vi "FRAM.vi"() -> ()   [LabVIEW 2019]
panel:
  out "PI-02- Bruto":dbl
  in  "P2-LIMITE":bool
  out "SHD-PI-02-AUX":dbl
  in  "Atualizar_Velocidades":bool
  out "JW_aux":dbl
  out "JK_aux":dbl
  out "JG_aux":dbl
  in  "JG_Title":string
  in  "JK_Title":string
  in  "JW_Title":string
  out "JG_Lam [m/s]":dbl
  out "T_K [°C]":dbl
  out "T_W [°C]":dbl
  in  "automatico/M_manual":bool
  in  "M_manual":dbl
  out "T_mis [°C]":dbl
  out "T_Atm_CLP":dbl
  out "Ll":dbl
  out "Lm":dbl
  out "T_Atm [°C]":dbl
  out "Lk":dbl
  out "Lw":dbl
  out "JL [m/s]":dbl
  out "T_W_CLP":dbl
  out "T_K_CLP":dbl
  out "SKM-NC-CV-COR":bool
  out "SKM-NC-CV-LAM":bool
  out "T_Ar_CLP":dbl
  out "DP_Lam_CLP":dbl
  out "SKM-AI-KF-COR_CLP [kg/m³]":dbl
  out "P_Bar_CLP":dbl
  out "P_Lam_CLP":dbl
  out "M_K_CLP":dbl
  out "P_Lam [KPa]":dbl
  out "P_Bar [KPa]":dbl
  out "Q_W_CLP":dbl
  out "Q_W [m³/s]":dbl
  out "DP_Lam [KPa]":dbl
  out "SKM-FIC-AR-COR_CLP  [kg/s]":dbl
  out "T_Ar [°C]":dbl
  out "Rho_K [Kg/m³]":dbl
  out "Rho_W [Kg/m³]":dbl
  out "SIT-NC-CV-001":bool
  out "SIA-NC-CV-001":bool
  out "SKS-NC-CV-006":bool
  out "SIW-NC-CV-001":bool
  out "SKS-NC-CV-003":bool
  out "SKS-NC-CV-002":bool
  out "SIT-NC-CV-002":bool
  in  "Certificado_Calibracao 2":bool
  in  "Certificado_Calibracao1":bool
  out "Execution:State":T1(ring)
  out "SHD-PI-02":dbl(knob) scale=2.0..2000.0
  out "STRING":string
  in  "Teste 234":bool
  in  "MWU2987":i16
  out "String Caracter de Comunicação":string
  out "JG [m/s]":dbl
  out "JW [m/s]":dbl
  out "JK [m/s]":dbl
  in  "MWU2986":i16
  in  "MWU2985":i16
  in  "MWU2984":i16
  in  "MWU2983":i16
  in  "MWU2982":i16
  in  "MWU2981":i16
  in  "MWU2980":i16
  in  "MWU2979":i16
  in  "MWU2978":i16
  in  "MWU2977":i16
  in  "MWU2976":i16
  in  "MWU2975":i16
  in  "MWU2925":i16
  out "MWU1100":i16
  in  "caixinha":bool
  out "Altura Líquido-régua":dbl
  out "Altura Kerosene-régua":dbl
  out "Altura Água-régua":dbl
  out "Hk Mer erro":dbl format="%.6g"
  out "Hw Mer erro":dbl format="%.6g"
  out "Vazio Mer erro":dbl format="%.6g"
  out "Hk Free erro":dbl format="%.6g"
  out "Hw Free erro":dbl format="%.6g"
  out "Vazio Free erro":dbl format="%.6g"
  out "Hk  Misto erro":dbl format="%.6g"
  out "Hw Misto erro":dbl format="%.6g"
  out "Vazio Misto erro":dbl format="%.6g"
  out "led Hw":bool
  out "led Hk":bool
  out "led Vazio":bool
  out "led SHD":bool
  out "Altura Liquido erro":dbl format="%#_1g"
  in  "Calibração":bool
  out "Altura Kerosene erro":dbl format="%#_4g"
  out "Altura Água erro":dbl format="%#_4g"
  out "Hw Mer":dbl format="%#_3g"
  out "Hk Mer":dbl format="%#_3g"
  out "Vazio Mer":dbl format="%#_3g"
  in  "Documentação":bool
  in  "Cluster 2":T2
  in  "Cluster":T3 {"Progresso Sensor" scale=0.0..90.0}
  out "SHD-PI-01":dbl(knob) scale=2.0..2000.0
  out "Gráfico":dbl[][](graph)
  out "Hw Free":dbl format="%#_3g"
  out "Hk Free":dbl format="%#_3g"
  out "Vazio  Free":dbl format="%#_3g"
  out "Hw":dbl format="%#_3g"
  out "Hk":dbl format="%#_3g"
  out "Vazio":dbl format="%#_3g"
  out "Altura Líquido":dbl
  in  "Alinhamento":bool
  in  "Gravar teste":bool
  in  "Parar Teste":bool
  out "SHD-PI-02-Ind.":dbl
  out "SHD-PI-01-Ind.":dbl
  out "T roxo":bool
  out "SIT-CV-AT":bool
  out "cano roxo h":bool
  out "SIT-CV-ST":bool
  out "SIT-CV-ST":bool
  out "cano roxo":bool
  out "Altura Kerosene":dbl
  out "Altura Água":dbl
  in  "Medição":bool
  in  "Teste":bool
  in  "stop VI":bool
  out "reference":refnum<vi>
  in  "Tempo de comunicação":i32
  in  "String 12":string
  in  "String 11":string
  in  "String 10":string
  in  "String 9":string
  in  "String 8":string
  in  "String 7":string
  in  "String 6":string
  in  "String 5":string
  in  "String 4":string
  in  "String 3":string
  in  "String 2":string
  in  "String 1":string
  out "UHk":dbl
  out "UHw":dbl
  out "Ua":dbl
  out "ULw":dbl
  out "Lw(valor mais provavel)":dbl
  out "Calculo de gama":dbl
  out "(Uwp2)²":dbl
  out "(Uwp1)²":dbl
  out "Lwp2":dbl
  out "Lwp1":dbl
  out "Uwd(incerteza free)":dbl
  out "L_w":dbl
  out "L_k":dbl
  in  "HELP-SIT":bool
  out "JANELA":bool
  out "HKSO":dbl
  out "HWSO":dbl
  out "L_a":dbl
  out "H L":dbl
  out "Rho_Ar [kg/m³]":dbl
  out "P1-P2":dbl
  out "PM":dbl
  out "Valores":T4
  out "Hexa p OPC":string
  in  "Pressão02-CLP[0-4095]":dbl
  in  "Pressão01_CLP[0-4095]":dbl
  out "T azul":bool
  out "cano azul h":bool
  out "cano verde":bool
  out "cano amarelo":bool
  out "cano azul v":bool
  # "FreeScale"
  # "Pressão"
  # "Ótico"
  # "Régua"
  # "Altura\nLíquido"
  # "+"
  # "mm"
  # "mm"
  # "mm"
  # "-"
  # "Altura\nÁgua"
  # "+"
  # "mm"
  # "mm"
  # "mm"
  # "-"
  # "Altura \nQuerosene"
  # "+"
  # "mm"
  # "mm"
  # "mm"
  # "-"
  # "Merge"
  # "FreeScale"
  # "Misto"
  # "[%]"
  # "[Erro]"
  # "[%]"
  # "[Erro]"
  # "[%]"
  # "[Erro]"
  # "+"
  # "+"
  # "Vazão Mássica - Manual"
  # "+"
  # "-"
  # "-"
  # "-"
  # "+"
  # "+"
  # "+"
  # "-"
  # "-"
  # "-"
  # "Variaveis Merge"
  # "+"
  # "+"
  # "+"
  # "-"
  # "-"
  # "-"
  # "mm"
  # "mmH2O"
  # "Smar"
  # "Emerson"
  # "Insira os valores de JW, JK e JG para criação do título do arquivo gravado:"
  # "mm"
  # "mm²"
  # "ms"
  # "mmH2O"
  # "mm"
  # "mm"
  # "mm²"
  # "mm"
  # "mm"
  # "JW [m/s]"
  # "COMUNICA敲O SERIAL"
  # "mm"
  # "mm"
  # "mm"
  # "JK [m/s]"
  # "mm"
  # "mm"
  # "Kg/m³"
  # "JG [m/s]"
  # "mm"
  # "mm"
  # "KPa Abs."
  # "mmH2O"
  # "[s]"
  # "MAX"
  # "MIN"
  # "mmH2O"
  # "mmH2O"
  # "mm"
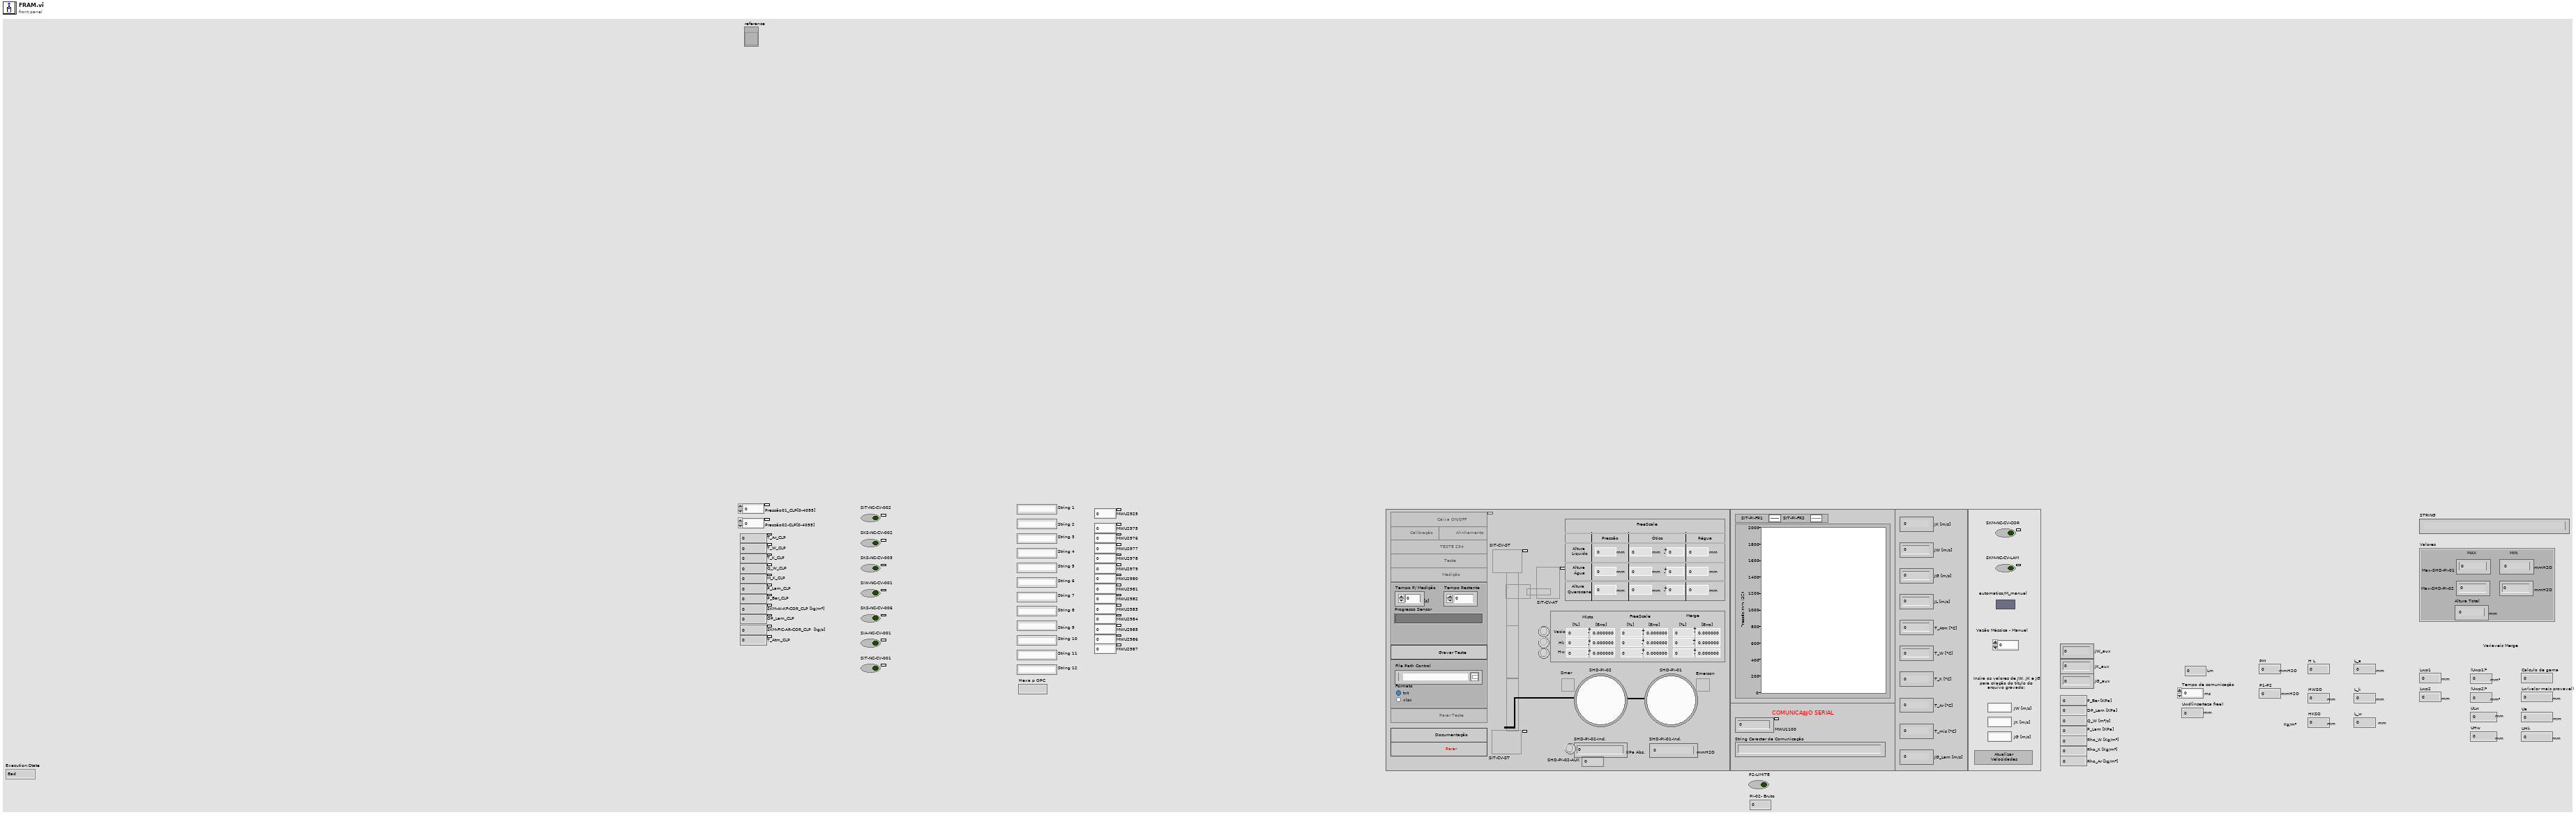
[diagram p1: front panel]
types:
  T1 = enum32{"Bad", "Idle", "Run top level", "Running"}
  T2 = cluster{"File Path Control":path, "Formato":enum32{"Item 0", "Item 1"}}
  T3 = cluster{"Tempo P/ Medição":dbl, "Tempo Restante":dbl, "Home":bool, "Progresso Sensor":dbl}
  T4 = cluster{"Max-SHD-PI-01":i32, "Min-SIT-PI-FR1":i32, "Max-SHD-PI-02":i32, "Min-SIT-PI-FR2":i32, "Altura Total":i32}
  T5 = enum8{"Enabled", "Disabled", "Disabled and Grayed Out"}
  T6 = enum32{"Invalid", "Standard", "Closed", "Hidden", "Minimized", "Maximized"}
  T7 = cluster{"String para labview 1":string, "String para labview 2":string, "String para labview 3":string, "String para labview 4":string, "String para labview 5":string, "String para labview 6":string, "String para labview 7":string, "String para labview 8":string, "String para labview 9":string, "String para labview 10":string, "String para labview 11":string, "String para labview 12":string}
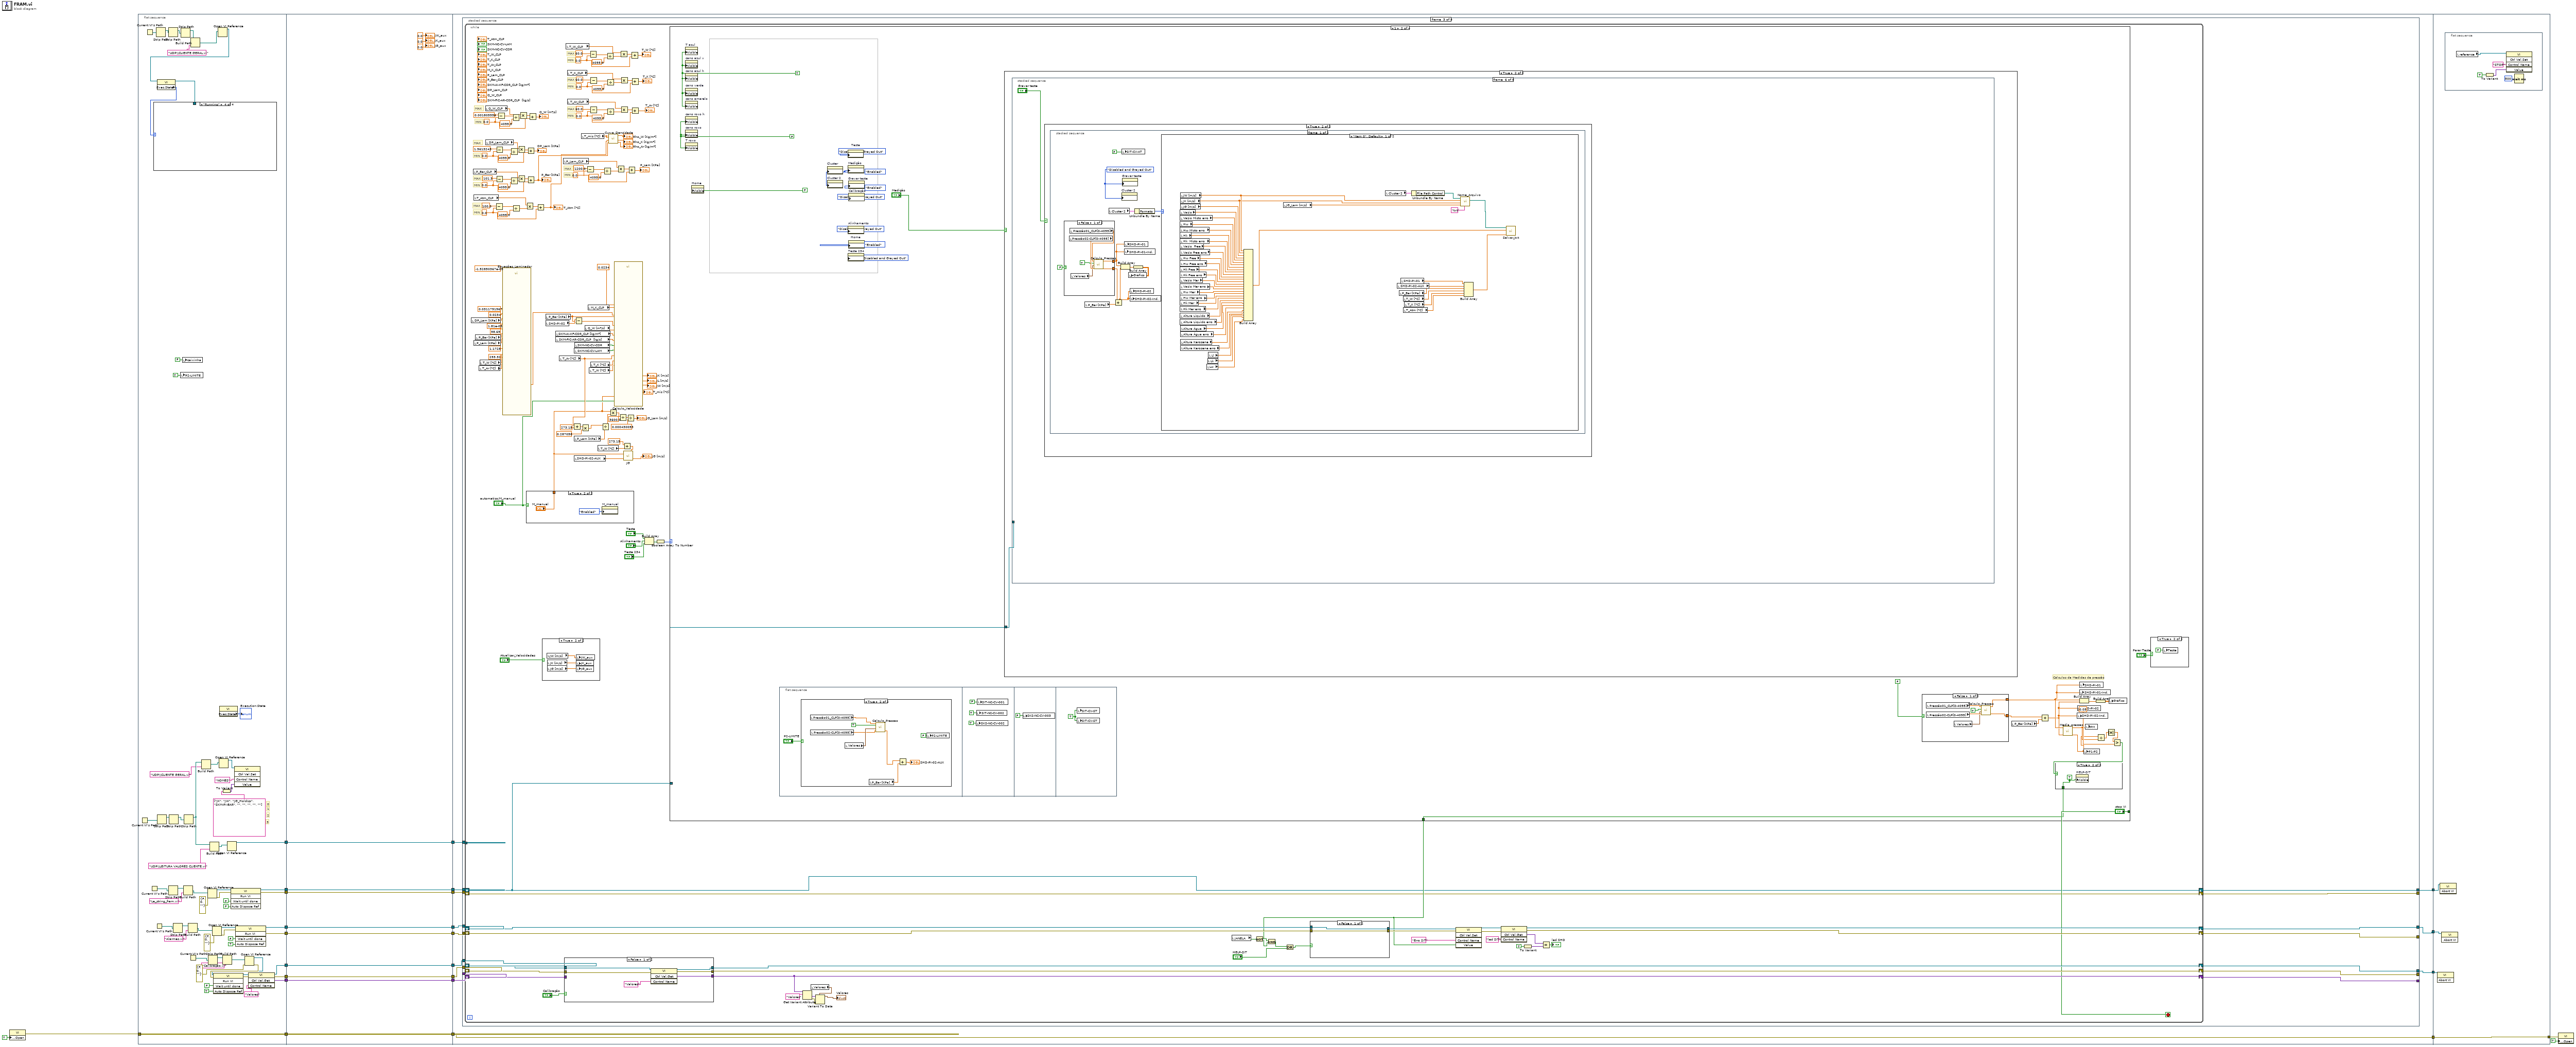
[diagram p0: block diagram]
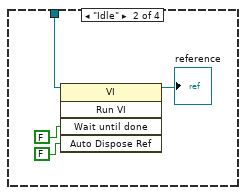
[diagram p3: hidden frame]
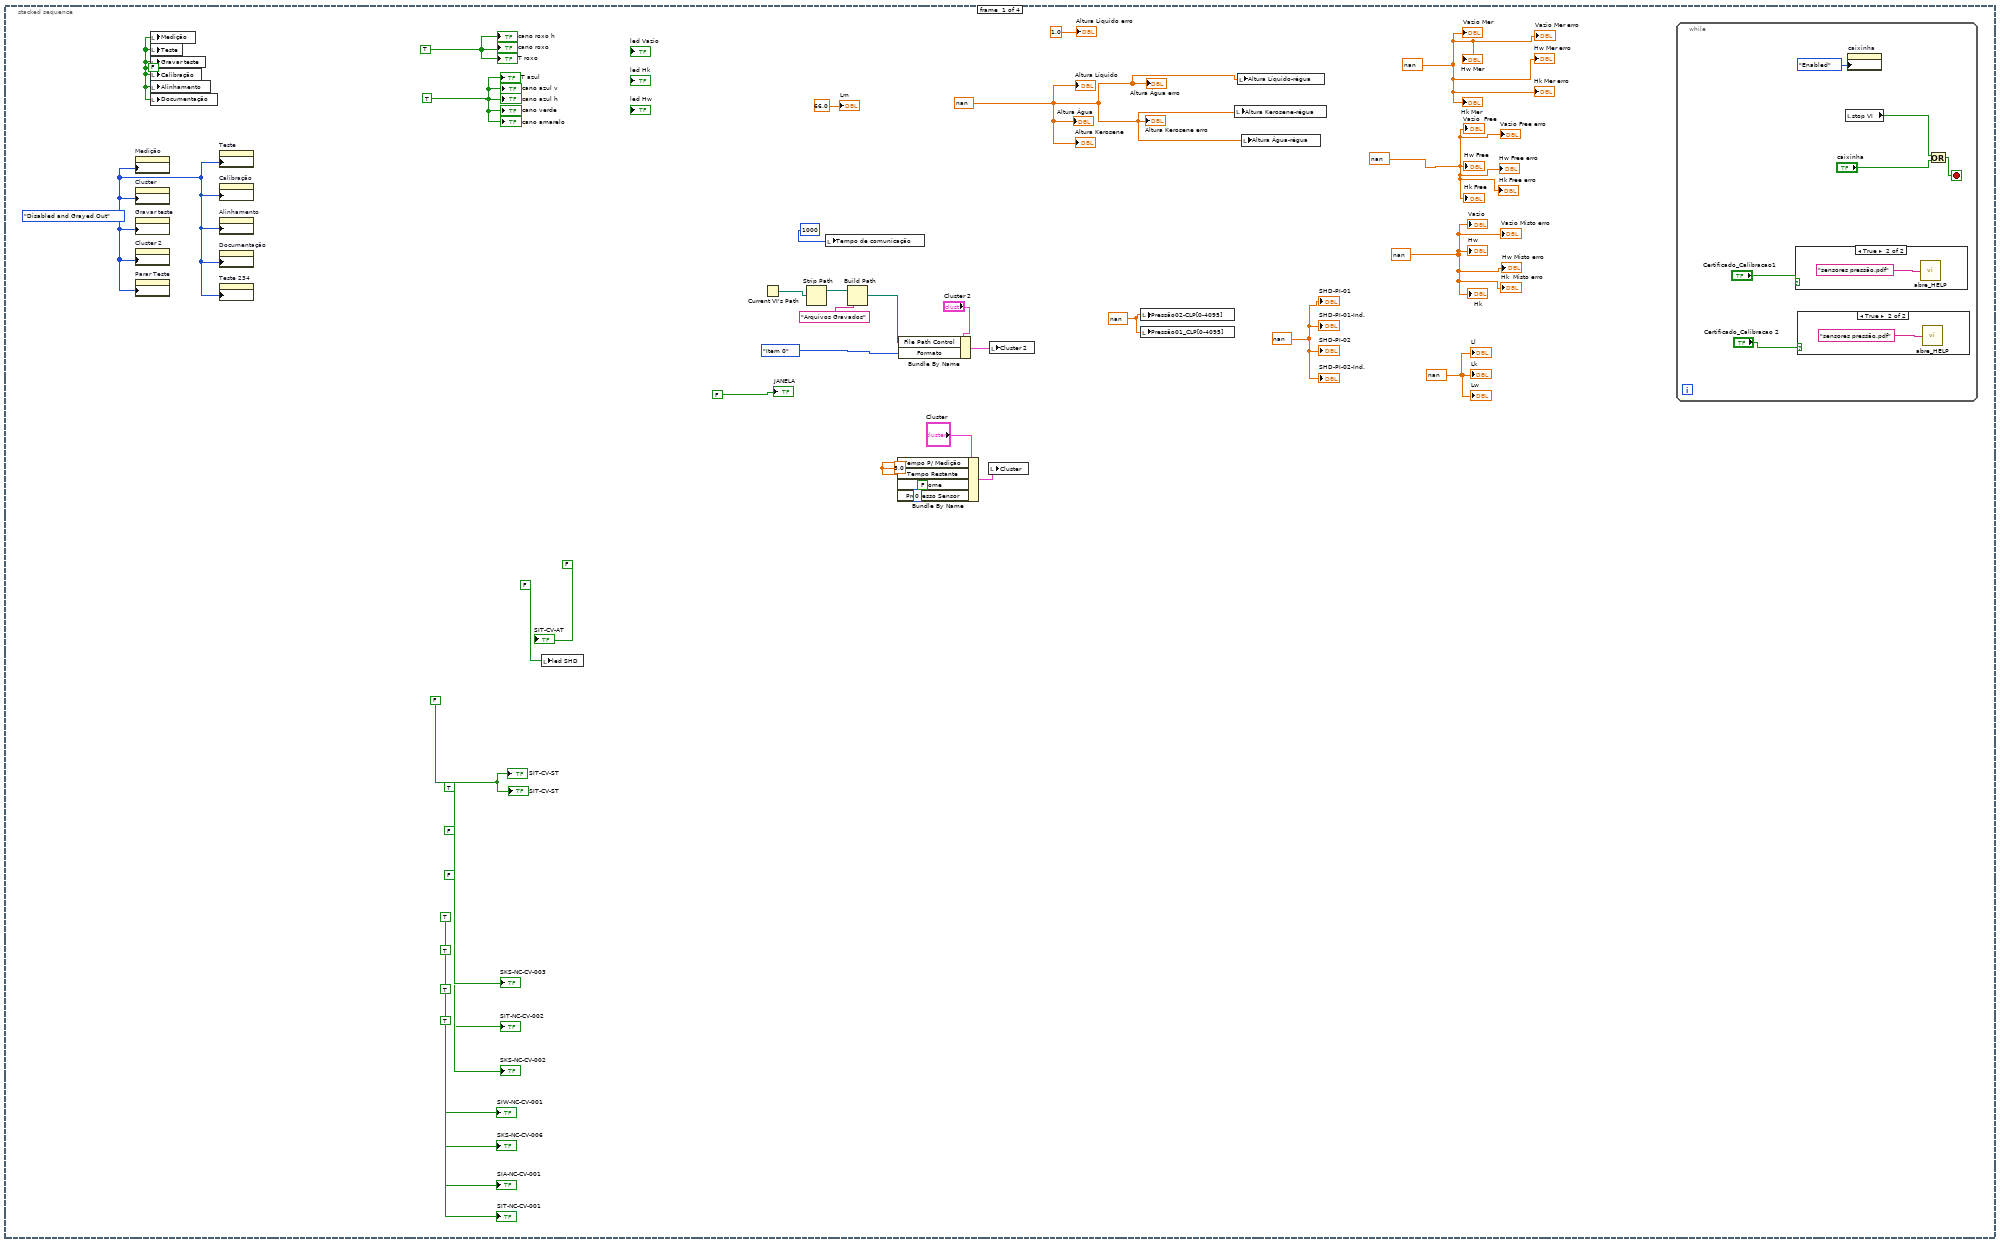
[diagram p5: hidden frame]
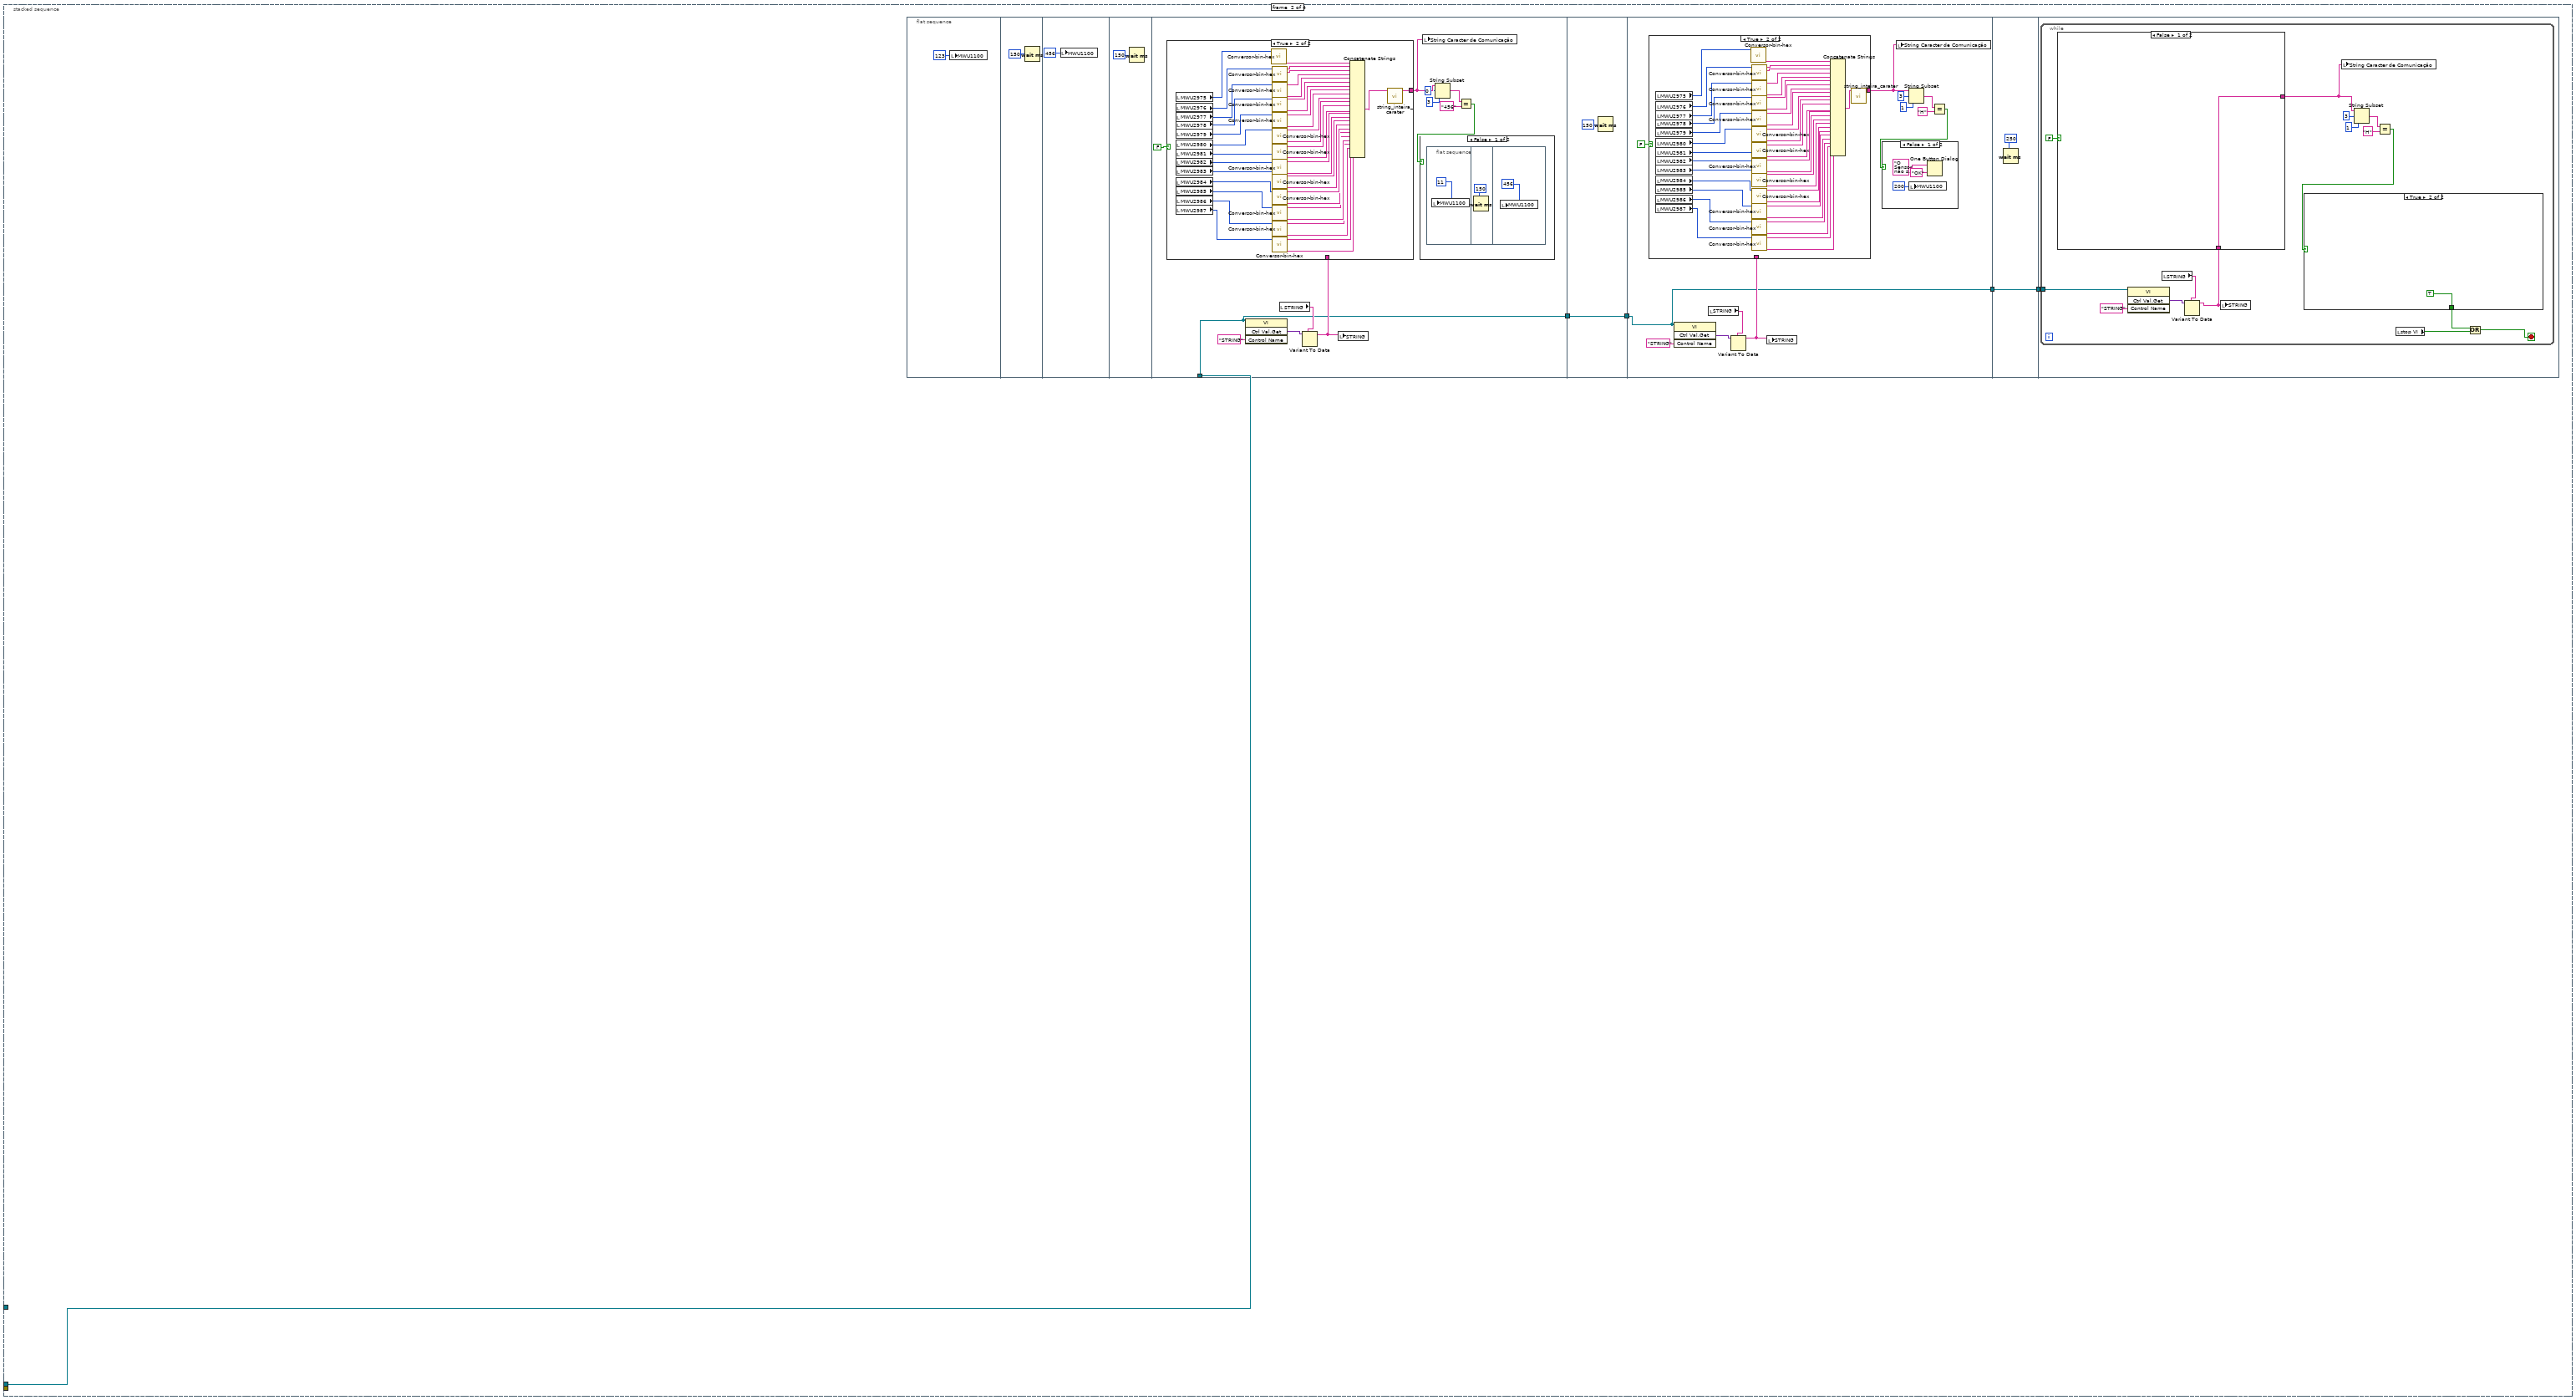
[diagram p8: hidden frame]
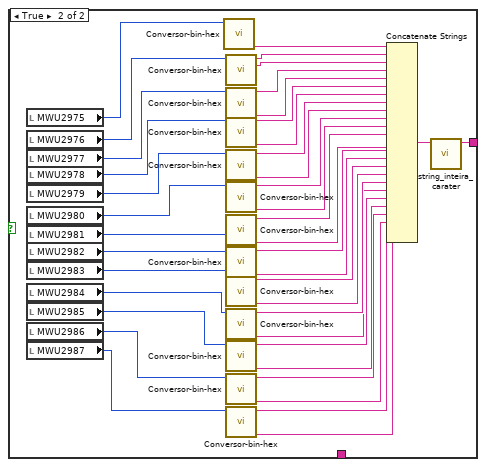
[diagram p13: hidden frame]
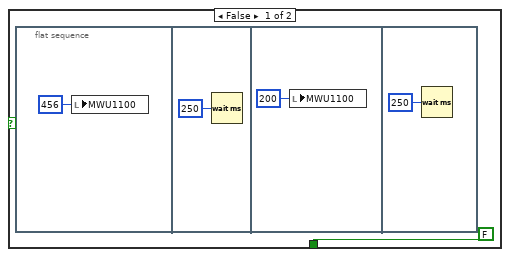
[diagram p14: hidden frame]
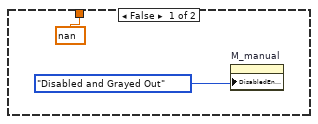
[diagram p16: hidden frame]
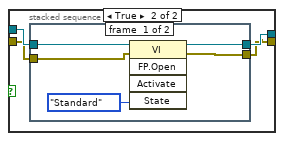
[diagram p17: hidden frame]
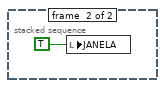
[diagram p18: hidden frame]
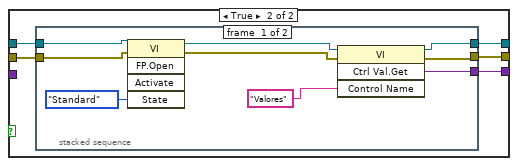
[diagram p19: hidden frame]
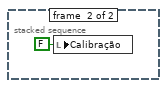
[diagram p20: hidden frame]
diagram:
  n1 = property class="VI"("Front Panel.Open"=TRUE ("Front Panel Window:Open")) -> (error out=w26:errorcluster)  [unwired: 2 in, 1 out]
  n2 = flat-sequence {
    tunnel: w26 -> [w89]
    tunnel: [w89] -> w18
    tunnel: [w73] -> w16
    tunnel: [w59] -> w14
    tunnel: [w58] -> w12
    tunnel: [w57] -> w10
    tunnel: [w44] -> w8
    tunnel: [w43] -> w6
    tunnel: [w33] -> w4
    tunnel: [w32] -> w2
    tunnel: w18 -> [w105]
    tunnel: [w105] -> w17
    tunnel: w16 -> [w104]
    tunnel: [w104] -> w15
    tunnel: w14 -> [w103]
    tunnel: [w103] -> w13
    tunnel: w12 -> [w102]
    tunnel: [w102] -> w11
    tunnel: w10 -> [w101]
    tunnel: [w101] -> w9
    tunnel: w8 -> [w100]
    tunnel: [w100] -> w7
    tunnel: w6 -> [w99]
    tunnel: [w99] -> w5
    tunnel: w4 -> [w98]
    tunnel: [w98] -> w3
    tunnel: w2 -> [w97]
    tunnel: [w97] -> w1
    tunnel: [w117] -> w22
    tunnel: w17 -> [w117]
    tunnel: w15 -> [w106]
    tunnel: w13 -> [w116]
    tunnel: w11 -> [w115]
    tunnel: w9 -> [w114]
    tunnel: [w113] -> w21
    tunnel: w7 -> [w112]
    tunnel: w5 -> [w111]
    tunnel: [w110] -> w20
    tunnel: w3 -> [w109]
    tunnel: w1 -> [w108]
    tunnel: [w107] -> w19
    tunnel: [w2033] -> w25
    tunnel: w22 -> [w2033]
    tunnel: w21 -> [w2032]
    tunnel: w20 -> [w2031]
    tunnel: w19 -> [w2030]
    frame #0 {
      # "3"
      # "2"
      # "1"
      # "0"
      n3 = Current VI's Path() -> (path=w77:path)
      n4 = Current VI's Path() -> (path=w84:path)
      n5 = Current VI's Path() -> (path=w37:path)
      n6 = Current VI's Path() -> (path=w50:path)
      n7 = Strip Path(path=w84) -> (stripped path=w85:path)  [unwired: 1 out]
      n8 = Strip Path(path=w77) -> (stripped path=w76:path)  [unwired: 1 out]
      n9 = Strip Path(path=w85) -> (stripped path=w86:path)  [unwired: 1 out]
      n10 = Strip Path(path=w37) -> (stripped path=w38:path)  [unwired: 1 out]
      n11 = Strip Path(path=w76) -> (stripped path=w79:path)  [unwired: 1 out]
      n12 = Strip Path(path=w50) -> (stripped path=w49:path)  [unwired: 1 out]
      n13 = local write "P2-LIMITE"(TRUE) -> ()
      n14 = Strip Path(path=w86) -> (stripped path=w87:path)  [unwired: 1 out]
      n15 = local write "caixinha"(FALSE ("caixinha")) -> ()
      n16 = Build Path(base path=w38, name or relative path="Le_string_fram.vi") -> (appended path=w35:path)
      n17 = Strip Path(path=w79) -> (stripped path=w80:path)  [unwired: 1 out]
      n18 = Build Path(base path=w49, name or relative path="Alarmes.vi") -> (appended path=w52:path)
      n19 = Current VI's Path() -> (path=w55:path)
      n20 = Build Path(base path=w87, name or relative path="UDP\\CLIENTE GERAL.vi") -> (appended path=w88:path)
      n21 = Build Path(base path=w80, name or relative path="UDP\\CLIENTE GERAL.vi") -> (appended path=w78:path)
      n22 = Open VI Reference(vi path=w35, error in (no error)=errorcluster {"status"=FALSE, "code"=0, "source"=""}) -> (vi reference=w36:refnum<vi>, error out=w34:errorcluster)  [unwired: 4 in]
      n23 = Strip Path(path=w55) -> (stripped path=w54:path)  [unwired: 1 out]
      n24 = Build Path(base path=w80, name or relative path="UDP\\LEITURA VALORES CLIENTE.vi") -> (appended path=w81:path)
      n25 = Open VI Reference(vi path=w52, error in (no error)=errorcluster {"status"=FALSE, "code"=0, "source"=""}) -> (vi reference=w51:refnum<vi>, error out=w53:errorcluster)  [unwired: 4 in]
      n26 = Open VI Reference(vi path=w88) -> (vi reference=w30:refnum<vi>)  [unwired: 5 in, 1 out]
      n27 = property class="VI"(reference=w30) -> (reference out=w28:refnum<vi>, "Exec.State"=w29:T1)  [unwired: 1 in, 1 out]
      n28 = case shown="\"Running\"" w29 {
        tunnel: w28 -> [_ w91 _ _]
        frame "Bad", Default {
        }
        frame "Idle" {
          n29 = invoke class="VI" method="Run VI"(reference=w91, "Wait until done"=FALSE ("Wait Until Done"), "Auto Dispose Ref"=FALSE ("Auto Dispose Reference")) -> (reference out=→"reference":refnum<vi>)  [unwired: 2 in, 4 out]
        }
        frame "Run top level" {
        }
        frame "Running" {
        }
      }
      n30 = Open VI Reference(vi path=w78) -> (vi reference=w69:refnum<vi>)  [unwired: 5 in, 1 out]
      n31 = property class="VI"() -> ("Exec.State"=→"Execution:State":T1)  [unwired: 2 in, 2 out]
      n32 = To Variant(anything=string[] ["JK", "JW", "JG_HoldUp", "SKM-PI-BAR", "", "", "", "", ""] ("NOMES")) -> (Variant=w72:variant)
      n33 = Build Path(base path=w54, name or relative path="Calibração.vi") -> (appended path=w67:path)
      n34 = Open VI Reference(vi path=w81) -> (vi reference=w73:refnum<vi>)  [unwired: 5 in, 1 out]
      n35 = invoke class="VI" method="Run VI"(reference=w36, error in=w34, "Wait until done"=FALSE ("Wait Until Done"), "Auto Dispose Ref"=FALSE ("Auto Dispose Reference")) -> (reference out=w33:refnum<vi>, error out=w32:errorcluster)  [unwired: 1 in, 3 out]
      n36 = invoke class="VI" method="Ctrl Val.Set"(reference=w69, "Control Name"="NOMES", "Value"=w72) -> ()  [unwired: 2 in, 5 out]
      n37 = invoke class="VI" method="Run VI"(reference=w51, error in=w53, "Wait until done"=FALSE ("Wait Until Done"), "Auto Dispose Ref"=TRUE ("Auto Dispose Reference")) -> (reference out=w44:refnum<vi>, error out=w43:errorcluster)  [unwired: 1 in, 3 out]
      n38 = Open VI Reference(vi path=w67, error in (no error)=errorcluster {"status"=FALSE, "code"=0, "source"=""}) -> (vi reference=w56:refnum<vi>, error out=w68:errorcluster)  [unwired: 4 in]
      n39 = invoke class="VI" method="Run VI"(reference=w56, error in=w68, "Wait until done"=FALSE ("Wait Until Done"), "Auto Dispose Ref"=TRUE ("Auto Dispose Reference")) -> (reference out=w65:refnum<vi>, error out=w66:errorcluster)  [unwired: 1 in, 3 out]
      n40 = invoke class="VI" method="Ctrl Val.Get"(reference=w65, error in=w66, "Control Name"="Valores") -> (reference out=w59:refnum<vi>, error out=w58:errorcluster, "Get Control Value Variant"=w57:variant)  [unwired: 1 in, 1 out]
    }
    frame #1 {
      "JG_aux" <- 0.0 ("JG_aux")
      "JK_aux" <- 0.0 ("JK_aux")
      "JW_aux" <- 0.0 ("JW_aux")
    }
    frame #2 {
      n41 = stacked-sequence {
        tunnel: w116 -> [_ _ w365 _]
        tunnel: w115 -> [_ _ w364 _]
        tunnel: w114 -> [_ _ w363 _]
        tunnel: [_ _ w362 _] -> w113
        tunnel: [_ _ w361 _] -> _
        tunnel: [_ _ w360 _] -> _
        tunnel: w112 -> [_ _ w359 _]
        tunnel: w111 -> [_ _ w358 _]
        tunnel: [_ _ w357 _] -> w110
        tunnel: [_ _ w356 _] -> _
        tunnel: w109 -> [_ w163 w355 _]
        tunnel: w108 -> [_ _ w354 _]
        tunnel: [_ _ w353 _] -> w107
        tunnel: [_ _ w352 _] -> _
        tunnel: w106 -> [_ _ w351 _]
        frame #0 {
          w118 = nan ("Ll")
          w119 = nan ("SKM1")
          w129 = T5."Disabled and Grayed Out" ("Disabled")
          w128 = nan
          w139 = nan
          w140 = nan
          w141 = nan
          w146 = 5.0 ("Tempo para Medir")
          w152 = nan ("SKM1")
          w145 = FALSE ("SKT 1")
          w132 = FALSE ("Alinhamento")
          w154 = TRUE
          w153 = TRUE
          n42 = property on="Medição" class="Bool (strict)"("DisabledEnum"=w129) -> ()  [unwired: 2 in, 2 out]
          n43 = property on="Cluster" class="Clust (strict)"("DisabledEnum"=w129) -> ()  [unwired: 2 in, 2 out]
          n44 = property on="Gravar teste" class="Bool (strict)"("DisabledEnum"=w129) -> ()  [unwired: 2 in, 2 out]
          n45 = property on="Cluster 2" class="Clust (strict)"("DisabledEnum"=w129) -> ()  [unwired: 2 in, 2 out]
          n46 = property on="Parar Teste" class="Bool"("DisabledEnum"=w129) -> ()  [unwired: 2 in, 2 out]
          n47 = local write "Medição"(w132) -> ()
          n48 = local write "Teste"(w132) -> ()
          n49 = local write "Gravar teste"(w132) -> ()
          n50 = local write "Calibração"(w132) -> ()
          n51 = local write "Alinhamento"(w132) -> ()
          n52 = local write "Documentação"(w132) -> ()
          n53 = property on="Teste" class="Bool (strict)"("DisabledEnum"=w129) -> ()  [unwired: 2 in, 2 out]
          n54 = property on="Calibração" class="Bool (strict)"("DisabledEnum"=w129) -> ()  [unwired: 2 in, 2 out]
          n55 = property on="Alinhamento" class="Bool (strict)"("DisabledEnum"=w129) -> ()  [unwired: 2 in, 2 out]
          n56 = property on="Documentação" class="Bool (strict)"("DisabledEnum"=w129) -> ()  [unwired: 2 in, 2 out]
          n57 = property on="Teste 234" class="Bool (strict)"("DisabledEnum"=w129) -> ()  [unwired: 2 in, 2 out]
          n58 = local write "led SHD"(FALSE ("Botão erro")) -> ()
          n59 = Current VI's Path() -> (path=w137:path)
          n60 = Strip Path(path=w137) -> (stripped path=w138:path)  [unwired: 1 out]
          n61 = local write "Tempo de comunicação"(1000 ("Tempo de comunicação")) -> ()
          n62 = Build Path(base path=w138, name or relative path="Arquivos Gravados") -> (appended path=w135:path)
          n63 = Bundle By Name(cluster="Cluster", "Tempo P/ Medição"=w146, "Tempo Restante"=w146, "Home"=FALSE, "Progresso Sensor"=0) -> (w151:T3)
          n64 = Bundle By Name(cluster="Cluster 2", "File Path Control"=w135, "Formato"=enum32{"Item 0", "Item 1"}."Item 0") -> (w150:T2)
          n65 = local write "Cluster"(w151) -> ()
          n66 = local write "Cluster 2"(w150) -> ()
          n67 = local write "Pressão02-CLP[0-4095]"(w119) -> ()
          n68 = local write "Pressão01_CLP[0-4095]"(w119) -> ()
          n69 = local write "Altura Kerosene-régua"(w128) -> ()
          n70 = local write "Altura Líquido-régua"(w128) -> ()
          n71 = local write "Altura Água-régua"(w128) -> ()
          n72 = while {
            stop <- w158 stop-if-true
            n73 = case shown="True" "Certificado_Calibracao1" {
              frame False {
              }
              frame True {
                n74 = call "abre_HELP.vi"("nome"="sensores pressão.pdf") -> ()  [unwired: 1 out]
              }
            }
            n75 = case shown="True" "Certificado_Calibracao 2" {
              frame False {
              }
              frame True {
                n76 = call "abre_HELP.vi"("nome"="sensores pressão.pdf") -> ()  [unwired: 1 out]
              }
            }
            n77 = local read "stop VI"() -> (w159:bool)
            n78 = property on="caixinha" class="Bool (strict)"("DisabledEnum"=T5."Enabled" ("Disabled")) -> ()  [unwired: 2 in, 2 out]
            n79 = Or(x=w159, y="caixinha") -> (x .or. y?=w158:bool)
          }
          "Altura Água" <- w128
          "Altura Kerosene" <- w128
          "Altura Líquido" <- w128
          "cano azul v" <- w153
          "cano amarelo" <- w153
          "cano verde" <- w153
          "cano roxo" <- w154
          "cano azul h" <- w153
          "cano roxo h" <- w154
          "SHD-PI-01" <- w152
          "SHD-PI-02" <- w152
          "T azul" <- w153
          "T roxo" <- w154
          "SHD-PI-01-Ind." <- w152
          "SHD-PI-02-Ind." <- w152
          "Vazio" <- w141
          "Hk" <- w141
          "Hw" <- w141
          "Vazio  Free" <- w140
          "Hk Free" <- w140
          "Hw Free" <- w140
          "Vazio Mer" <- w139
          "Hk Mer" <- w139
          "Hw Mer" <- w139
          "Altura Água erro" <- w128
          "Altura Kerosene erro" <- w128
          "SIT-CV-ST" <- w145
          "SIT-CV-ST" <- w145
          "SIT-CV-AT" <- FALSE ("SKT 3")
          "Altura Liquido erro" <- 1.0 ("Altura Liquido erro")
          "JANELA" <- FALSE ("ERRO-AUX")
          "Vazio Misto erro" <- w141
          "Hw Misto erro" <- w141
          "Hk  Misto erro" <- w141
          "Vazio Free erro" <- w140
          "Hw Free erro" <- w140
          "Hk Free erro" <- w140
          "Vazio Mer erro" <- w139
          "Hw Mer erro" <- w139
          "Hk Mer erro" <- w139
          "SIT-NC-CV-002" <- FALSE ("SIT-NC-CV-002")
          "SKS-NC-CV-002" <- FALSE ("SKS-NC-CV-002")
          "SKS-NC-CV-003" <- TRUE ("SKS-NC-CV-003")
          "SIW-NC-CV-001" <- TRUE ("SIW-NC-CV-001")
          "SKS-NC-CV-006" <- TRUE ("SKS-NC-CV-006")
          "SIA-NC-CV-001" <- TRUE ("SIA-NC-CV-001")
          "SIT-NC-CV-001" <- TRUE ("SIT-NC-CV-001")
          "Lm" <- 66.0 ("Ll")
          "Lk" <- w118
          "Lw" <- w118
          "Ll" <- w118
        }
        frame #1 {
          n80 = flat-sequence {
            tunnel: w163 -> [w173]
            tunnel: [w173] -> w167
            tunnel: w167 -> [w228]
            tunnel: [w228] -> w166
            tunnel: w166 -> [w230]
            tunnel: [w230] -> w165
            tunnel: w165 -> [w286]
            tunnel: [w286] -> w164
            tunnel: w164 -> [w288]
            frame #0 {
              n81 = local write "MWU1100"(i16 123 ("MWU1100")) -> ()
            }
            frame #1 {
              n82 = Wait (ms)(milliseconds to wait=u32 150) -> ()  [unwired: 1 out]
            }
            frame #2 {
              n83 = local write "MWU1100"(i16 456 ("MWU1100")) -> ()
            }
            frame #3 {
              n84 = Wait (ms)(milliseconds to wait=u32 150) -> ()  [unwired: 1 out]
            }
            frame #4 {
              n85 = invoke class="VI" method="Ctrl Val.Get"(reference=w173, "Control Name"="STRING") -> ("Get Control Value Variant"=w176:variant)  [unwired: 2 in, 3 out]
              n86 = local read "STRING"() -> (w177:string)
              n87 = Variant To Data(type=w177, Variant=w176) -> (data=w174:string)  [unwired: 1 in, 1 out]
              n88 = case shown="True" FALSE {
                tunnel: [w184 w185] -> w183
                tunnel: w174 -> [w184 _]
                frame False {
                }
                frame True {
                  n89 = local read "MWU2975"() -> (w202:i16)
                  n90 = local read "MWU2976"() -> (w201:i16)
                  n91 = local read "MWU2977"() -> (w200:i16)
                  n92 = local read "MWU2978"() -> (w199:i16)
                  n93 = local read "MWU2979"() -> (w198:i16)
                  n94 = local read "MWU2980"() -> (w197:i16)
                  n95 = local read "MWU2981"() -> (w196:i16)
                  n96 = local read "MWU2982"() -> (w195:i16)
                  n97 = local read "MWU2983"() -> (w194:i16)
                  n98 = local read "MWU2984"() -> (w193:i16)
                  n99 = local read "MWU2985"() -> (w192:i16)
                  n100 = local read "MWU2986"() -> (w191:i16)
                  n101 = local read "MWU2987"() -> (w190:i16)
                  n102 = call "Conversor-bin-hex.vi"("Numeric"=w202) -> ("hex integer string"=w224:string)  [unwired: 9 in, 1 out]
                  n103 = call "Conversor-bin-hex.vi"("Numeric"=w201) -> ("hex integer string"=w222:string, "hex integer string 2"=w223:string)  [unwired: 9 in]
                  n104 = call "Conversor-bin-hex.vi"("Numeric"=w200) -> ("hex integer string"=w220:string, "hex integer string 2"=w221:string)  [unwired: 9 in]
                  n105 = call "Conversor-bin-hex.vi"("Numeric"=w199) -> ("hex integer string"=w218:string, "hex integer string 2"=w219:string)  [unwired: 9 in]
                  n106 = call "Conversor-bin-hex.vi"("Numeric"=w198) -> ("hex integer string"=w216:string, "hex integer string 2"=w217:string)  [unwired: 9 in]
                  n107 = call "Conversor-bin-hex.vi"("Numeric"=w197) -> ("hex integer string"=w214:string, "hex integer string 2"=w215:string)  [unwired: 9 in]
                  n108 = call "Conversor-bin-hex.vi"("Numeric"=w196) -> ("hex integer string"=w212:string, "hex integer string 2"=w213:string)  [unwired: 9 in]
                  n109 = call "Conversor-bin-hex.vi"("Numeric"=w195) -> ("hex integer string"=w210:string, "hex integer string 2"=w211:string)  [unwired: 9 in]
                  n110 = call "Conversor-bin-hex.vi"("Numeric"=w194) -> ("hex integer string"=w208:string, "hex integer string 2"=w209:string)  [unwired: 9 in]
                  n111 = call "Conversor-bin-hex.vi"("Numeric"=w193) -> ("hex integer string"=w206:string, "hex integer string 2"=w207:string)  [unwired: 9 in]
                  n112 = call "Conversor-bin-hex.vi"("Numeric"=w192) -> ("hex integer string"=w204:string, "hex integer string 2"=w205:string)  [unwired: 9 in]
                  n113 = call "Conversor-bin-hex.vi"("Numeric"=w191) -> ("hex integer string"=w189:string, "hex integer string 2"=w203:string)  [unwired: 9 in]
                  n114 = call "Conversor-bin-hex.vi"("Numeric"=w190) -> ("hex integer string"=w187:string, "hex integer string 2"=w188:string)  [unwired: 9 in]
                  n115 = Concatenate Strings(w224, w223, w222, w221, w220, w219, w218, w217, w216, w215, w214, w213, w212, w211, w210, w209, w208, w207, w206, w205, w204, w203, w189, w188, w187) -> (w186:string)
                  n116 = call "string_inteira_carater.vi"("String in"=w186) -> ("String out"=w185:string)  [unwired: 10 in]
                }
              }
              n117 = local write "STRING"(w174) -> ()
              n118 = local write "String Caracter de Comunicação"(w183) -> ()
              n119 = String Subset(string=w183, offset (0)=0, length (rest)=3 ("length (rest)")) -> (substring=w180:string)
              n120 = Equal?(x=w180, y="456") -> (x = y?=w172:bool)
              n121 = case shown="False" w172 {
                frame False {
                  n122 = flat-sequence {
                    frame #0 {
                      n123 = local write "MWU1100"(i16 11 ("MWU1100")) -> ()
                    }
                    frame #1 {
                      n124 = Wait (ms)(milliseconds to wait=u32 150) -> ()  [unwired: 1 out]
                    }
                    frame #2 {
                      n125 = local write "MWU1100"(i16 456 ("MWU1100")) -> ()
                    }
                  }
                }
                frame True {
                }
              }
            }
            frame #5 {
              n126 = Wait (ms)(milliseconds to wait=u32 150) -> ()  [unwired: 1 out]
            }
            frame #6 {
              n127 = invoke class="VI" method="Ctrl Val.Get"(reference=w230, "Control Name"="STRING") -> ("Get Control Value Variant"=w233:variant)  [unwired: 2 in, 3 out]
              n128 = local read "STRING"() -> (w232:string)
              n129 = Variant To Data(type=w232, Variant=w233) -> (data=w231:string)  [unwired: 1 in, 1 out]
              n130 = case shown="True" FALSE {
                tunnel: [w242 w282] -> w236
                tunnel: w231 -> [w242 _]
                frame False {
                }
                frame True {
                  n131 = local read "MWU2975"() -> (w265:i16)
                  n132 = local read "MWU2976"() -> (w266:i16)
                  n133 = local read "MWU2977"() -> (w267:i16)
                  n134 = local read "MWU2978"() -> (w268:i16)
                  n135 = local read "MWU2979"() -> (w269:i16)
                  n136 = local read "MWU2980"() -> (w270:i16)
                  n137 = local read "MWU2981"() -> (w271:i16)
                  n138 = local read "MWU2982"() -> (w272:i16)
                  n139 = local read "MWU2983"() -> (w273:i16)
                  n140 = local read "MWU2984"() -> (w274:i16)
                  n141 = local read "MWU2985"() -> (w275:i16)
                  n142 = local read "MWU2986"() -> (w276:i16)
                  n143 = local read "MWU2987"() -> (w277:i16)
                  n144 = call "Conversor-bin-hex.vi"("Numeric"=w265) -> ("hex integer string"=w243:string)  [unwired: 9 in, 1 out]
                  n145 = call "Conversor-bin-hex.vi"("Numeric"=w266) -> ("hex integer string"=w245:string, "hex integer string 2"=w244:string)  [unwired: 9 in]
                  n146 = call "Conversor-bin-hex.vi"("Numeric"=w267) -> ("hex integer string"=w247:string, "hex integer string 2"=w246:string)  [unwired: 9 in]
                  n147 = call "Conversor-bin-hex.vi"("Numeric"=w268) -> ("hex integer string"=w249:string, "hex integer string 2"=w248:string)  [unwired: 9 in]
                  n148 = call "Conversor-bin-hex.vi"("Numeric"=w269) -> ("hex integer string"=w251:string, "hex integer string 2"=w250:string)  [unwired: 9 in]
                  n149 = call "Conversor-bin-hex.vi"("Numeric"=w270) -> ("hex integer string"=w253:string, "hex integer string 2"=w252:string)  [unwired: 9 in]
                  n150 = call "Conversor-bin-hex.vi"("Numeric"=w271) -> ("hex integer string"=w255:string, "hex integer string 2"=w254:string)  [unwired: 9 in]
                  n151 = call "Conversor-bin-hex.vi"("Numeric"=w272) -> ("hex integer string"=w257:string, "hex integer string 2"=w256:string)  [unwired: 9 in]
                  n152 = call "Conversor-bin-hex.vi"("Numeric"=w273) -> ("hex integer string"=w259:string, "hex integer string 2"=w258:string)  [unwired: 9 in]
                  n153 = call "Conversor-bin-hex.vi"("Numeric"=w274) -> ("hex integer string"=w261:string, "hex integer string 2"=w260:string)  [unwired: 9 in]
                  n154 = call "Conversor-bin-hex.vi"("Numeric"=w275) -> ("hex integer string"=w263:string, "hex integer string 2"=w262:string)  [unwired: 9 in]
                  n155 = call "Conversor-bin-hex.vi"("Numeric"=w276) -> ("hex integer string"=w278:string, "hex integer string 2"=w264:string)  [unwired: 9 in]
                  n156 = call "Conversor-bin-hex.vi"("Numeric"=w277) -> ("hex integer string"=w280:string, "hex integer string 2"=w279:string)  [unwired: 9 in]
                  n157 = Concatenate Strings(w243, w244, w245, w246, w247, w248, w249, w250, w251, w252, w253, w254, w255, w256, w257, w258, w259, w260, w261, w262, w263, w264, w278, w279, w280) -> (w281:string)
                  n158 = call "string_inteira_carater.vi"("String in"=w281) -> ("String out"=w282:string)  [unwired: 10 in]
                }
              }
              n159 = local write "STRING"(w231) -> ()
              n160 = local write "String Caracter de Comunicação"(w236) -> ()
              n161 = String Subset(string=w236, offset (0)=3, length (rest)=1 ("length (rest)")) -> (substring=w239:string)
              n162 = Equal?(x=w239, y="H") -> (x = y?=w241:bool)
              n163 = case shown="False" w241 {
                frame False {
                  n164 = local write "MWU1100"(i16 200 ("MWU1100")) -> ()
                  n165 = One Button Dialog(message="O Sensor não se encontra em HOME\nO comando já foi enviado, aguarde ele chegar", button name ("OK")="OK") -> ()  [unwired: 1 out]
                }
                frame True {
                }
              }
            }
            frame #7 {
              n166 = Wait (ms)(milliseconds to wait=u32 250) -> ()  [unwired: 1 out]
            }
            frame #8 {
              n167 = while {
                tunnel: w288 -> [w293]
                stop <- w290 stop-if-true
                n168 = invoke class="VI" method="Ctrl Val.Get"(reference=w293, "Control Name"="STRING") -> ("Get Control Value Variant"=w295:variant)  [unwired: 2 in, 3 out]
                n169 = local read "STRING"() -> (w296:string)
                n170 = Variant To Data(type=w296, Variant=w295) -> (data=w292:string)  [unwired: 1 in, 1 out]
                n171 = case shown="False" FALSE {
                  tunnel: [w304 w306] -> w303
                  tunnel: w292 -> [w304 _]
                  frame False {
                  }
                  frame True {
                    n172 = local read "MWU2975"() -> (w322:i16)
                    n173 = local read "MWU2976"() -> (w321:i16)
                    n174 = local read "MWU2977"() -> (w320:i16)
                    n175 = local read "MWU2978"() -> (w319:i16)
                    n176 = local read "MWU2979"() -> (w318:i16)
                    n177 = local read "MWU2980"() -> (w317:i16)
                    n178 = local read "MWU2981"() -> (w316:i16)
                    n179 = local read "MWU2982"() -> (w315:i16)
                    n180 = local read "MWU2983"() -> (w314:i16)
                    n181 = local read "MWU2984"() -> (w313:i16)
                    n182 = local read "MWU2985"() -> (w312:i16)
                    n183 = local read "MWU2986"() -> (w311:i16)
                    n184 = local read "MWU2987"() -> (w310:i16)
                    n185 = call "Conversor-bin-hex.vi"("Numeric"=w322) -> ("hex integer string"=w344:string)  [unwired: 9 in, 1 out]
                    n186 = call "Conversor-bin-hex.vi"("Numeric"=w321) -> ("hex integer string"=w342:string, "hex integer string 2"=w343:string)  [unwired: 9 in]
                    n187 = call "Conversor-bin-hex.vi"("Numeric"=w320) -> ("hex integer string"=w340:string, "hex integer string 2"=w341:string)  [unwired: 9 in]
                    n188 = call "Conversor-bin-hex.vi"("Numeric"=w319) -> ("hex integer string"=w338:string, "hex integer string 2"=w339:string)  [unwired: 9 in]
                    n189 = call "Conversor-bin-hex.vi"("Numeric"=w318) -> ("hex integer string"=w336:string, "hex integer string 2"=w337:string)  [unwired: 9 in]
                    n190 = call "Conversor-bin-hex.vi"("Numeric"=w317) -> ("hex integer string"=w334:string, "hex integer string 2"=w335:string)  [unwired: 9 in]
                    n191 = call "Conversor-bin-hex.vi"("Numeric"=w316) -> ("hex integer string"=w332:string, "hex integer string 2"=w333:string)  [unwired: 9 in]
                    n192 = call "Conversor-bin-hex.vi"("Numeric"=w315) -> ("hex integer string"=w330:string, "hex integer string 2"=w331:string)  [unwired: 9 in]
                    n193 = call "Conversor-bin-hex.vi"("Numeric"=w314) -> ("hex integer string"=w328:string, "hex integer string 2"=w329:string)  [unwired: 9 in]
                    n194 = call "Conversor-bin-hex.vi"("Numeric"=w313) -> ("hex integer string"=w326:string, "hex integer string 2"=w327:string)  [unwired: 9 in]
                    n195 = call "Conversor-bin-hex.vi"("Numeric"=w312) -> ("hex integer string"=w324:string, "hex integer string 2"=w325:string)  [unwired: 9 in]
                    n196 = call "Conversor-bin-hex.vi"("Numeric"=w311) -> ("hex integer string"=w309:string, "hex integer string 2"=w323:string)  [unwired: 9 in]
                    n197 = call "Conversor-bin-hex.vi"("Numeric"=w310) -> ("hex integer string"=w307:string, "hex integer string 2"=w308:string)  [unwired: 9 in]
                    n198 = Concatenate Strings(w344, w343, w342, w341, w340, w339, w338, w337, w336, w335, w334, w333, w332, w331, w330, w329, w328, w327, w326, w325, w324, w323, w309, w308, w307) -> (w305:string)
                    n199 = call "string_inteira_carater.vi"("String in"=w305) -> ("String out"=w306:string)  [unwired: 10 in]
                  }
                }
                n200 = local write "STRING"(w292) -> ()
                n201 = local write "String Caracter de Comunicação"(w303) -> ()
                n202 = String Subset(string=w303, offset (0)=3, length (rest)=1 ("length (rest)")) -> (substring=w300:string)
                n203 = Equal?(x=w300, y="H") -> (x = y?=w298:bool)
                n204 = case shown="True" w298 {
                  tunnel: [FALSE TRUE] -> w291
                  frame False {
                    n205 = flat-sequence {
                      frame #0 {
                        n206 = local write "MWU1100"(i16 456 ("MWU1100")) -> ()
                      }
                      frame #1 {
                        n207 = Wait (ms)(milliseconds to wait=u32 250) -> ()  [unwired: 1 out]
                      }
                      frame #2 {
                        n208 = local write "MWU1100"(i16 200 ("MWU1100")) -> ()
                      }
                      frame #3 {
                        n209 = Wait (ms)(milliseconds to wait=u32 250) -> ()  [unwired: 1 out]
                      }
                    }
                  }
                  frame True {
                  }
                }
                n210 = local read "stop VI"() -> (w289:bool)
                n211 = Or(x=w291, y=w289) -> (x .or. y?=w290:bool)
              }
            }
          }
        }
        frame #2 {
          n212 = while {
            shift-right: [w514] -> w362
            shift-left: w365 -> [w518]
            shift-right: [w515] -> w361
            shift-left: w364 -> [w517]
            shift-right: [w513] -> w360
            shift-left: w363 -> [w516]
            shift-right: [w501] -> w356
            shift-left: w358 -> [w507]
            shift-right: [w502] -> w357
            shift-left: w359 -> [w508]
            tunnel: w351 -> [_]
            shift-right: [w483] -> w353
            shift-left: w355 -> [w483]
            shift-right: [w484] -> w352
            shift-left: w354 -> [w484]
            stop <- w485 stop-if-true
            w399 = 0.0 ("y")
            w476 = 0.0 ("y")
            w468 = 0.0 ("y")
            w459 = 0.0 ("y")
            w452 = 0.0 ("y")
            w444 = 0.0 ("y")
            w437 = 0.0 ("y")
            w433 = 0.0 ("y")
            # "MIN"
            # "MAX"
            # "MIN"
            # "MAX"
            # "MIN"
            # "MAX"
            # "MIN"
            # "MAX"
            # "MIN"
            # "MAX"
            # "MIN"
            # "MAX"
            # "MIN"
            # "MAX"
            # "MIN"
            # "MAX"
            n213 = local read "DP_Lam [KPa]"() -> (w426:dbl)
            n214 = local read "P_Bar_CLP"() -> (w463:dbl)
            n215 = local read "T_Atm_CLP"() -> (w396:dbl)
            n216 = local read "P_Lam [KPa]"() -> (w422:dbl)
            n217 = local read "P_Bar [KPa]"() -> (w423:dbl)
            n218 = local read "T_Ar [°C]"() -> (w418:dbl)
            n219 = local read "T_W [°C]"() -> (w419:dbl)
            n220 = local read "Q_W_CLP"() -> (w471:dbl)
            n221 = local read "DP_Lam_CLP"() -> (w479:dbl)
            n222 = Subtract(x=100.0, y=w399) -> (x-y=w400:dbl)
            n223 = Subtract(x=1.9613243, y=w476) -> (x-y=w475:dbl)
            n224 = Subtract(x=101.3, y=w459) -> (x-y=w460:dbl)
            n225 = Subtract(x=0.001805556, y=w468) -> (x-y=w467:dbl)
            n226 = call "Equações_Laminador.vi"("DP_Lam [KPa]"=w426, "B [(m³/h)/mmCA²]"=-1.52850367e-05, "C [(m³/h)/mmCA]"=0.0311791967, "P* [KPa]"=98.69, "T* [K]"=293.32, "P_Bar [KPa]"=w423, "P_Lam [KPa]"=w422, "T_Lam [ºC]"=w418, "Rho* [Kg/m³]"=1.1725, "Mu* [Pa.s]"=1.81e-05, "Diâmetro da tubulação [m]"=0.0234, "T_Agua [ºC]"=w419) -> ("M_Lam [Kg/h]"=w379:dbl)  [unwired: 6 in, 9 out]
            n227 = Divide(x=w475, y=4095.0) -> (x/y=w474:dbl)
            n228 = Divide(x=w460, y=4095.0) -> (x/y=w461:dbl)
            n229 = Divide(x=w467, y=4095.0) -> (x/y=w466:dbl)
            n230 = Divide(x=w400, y=4095.0) -> (x/y=w401:dbl)
            n231 = Multiply(x=w479, y=w474) -> (x*y=w473:dbl)
            n232 = Multiply(x=w463, y=w461) -> (x*y=w462:dbl)
            n233 = Multiply(x=w471, y=w466) -> (x*y=w465:dbl)
            n234 = Multiply(x=w396, y=w401) -> (x*y=w402:dbl)
            n235 = Add(x=w473, y=w476) -> (x+y=→"DP_Lam [KPa]":dbl)
            n236 = Add(x=w462, y=w459) -> (x+y=w403:dbl)
            "P_Bar [KPa]" <- w403
            n237 = case shown="True" "automatico/M_manual" {
              tunnel: [nan ("M_manual") "M_manual"] -> w367
              frame False {
                n238 = property on="M_manual" class="DigNum (strict)"("DisabledEnum"=T5."Disabled and Grayed Out" ("Disabled")) -> ()  [unwired: 2 in, 2 out]
              }
              frame True {
                n239 = property on="M_manual" class="DigNum (strict)"("DisabledEnum"=T5."Enabled" ("Disabled")) -> ()  [unwired: 2 in, 2 out]
              }
            }
            n240 = Add(x=w465, y=w468) -> (x+y=→"Q_W [m³/s]":dbl)
            n241 = Add(x=w402, y=w399) -> (x+y=w394:dbl)
            "T_Atm [°C]" <- w394
            n242 = case shown="True" "Atualizar_Velocidades" {
              frame False {
              }
              frame True {
                n243 = local read "JW [m/s]"() -> (w524:dbl)
                n244 = local read "JK [m/s]"() -> (w525:dbl)
                n245 = local read "JG [m/s]"() -> (w526:dbl)
                n246 = local write "JW_aux"(w524) -> ()
                n247 = local write "JK_aux"(w525) -> ()
                n248 = local write "JG_aux"(w526) -> ()
              }
            }
            n249 = local read "P_Bar [KPa]"() -> (w374:dbl)
            n250 = local read "SHD-PI-02"() -> (w375:dbl)
            n251 = local read "SKM-AI-KF-COR_CLP [kg/m³]"() -> (w414:dbl)
            n252 = local read "SKM-FIC-AR-COR_CLP  [kg/s]"() -> (w413:dbl)
            n253 = local read "T_Ar [°C]"() -> (w383:dbl)
            n254 = local read "P_Lam_CLP"() -> (w454:dbl)
            n255 = case shown="False" "Calibração" {
              tunnel: [w545 w553] -> w514
              tunnel: [w546 w552] -> w515
              tunnel: [w547 w551] -> w513
              tunnel: w518 -> [w544 w550]
              tunnel: w517 -> [w543 w549]
              tunnel: w516 -> [_ _]
              frame False {
                n256 = invoke class="VI" method="Ctrl Val.Get"(reference=w544, error in=w543, "Control Name"="Valores") -> (reference out=w545:refnum<vi>, error out=w546:errorcluster, "Get Control Value Variant"=w547:variant)  [unwired: 1 in, 1 out]
              }
              frame True {
                n257 = stacked-sequence {
                  tunnel: [w558 _] -> w553
                  tunnel: [w557 _] -> w552
                  tunnel: [w556 _] -> w551
                  tunnel: w550 -> [w555 _]
                  tunnel: w549 -> [w554 _]
                  frame #0 {
                    n258 = invoke class="VI" method="FP.Open"(reference=w555, error in=w554, "State"=T6."Standard") -> (reference out=w560:refnum<vi>, error out=w559:errorcluster)  [unwired: 2 in, 3 out]
                    n259 = invoke class="VI" method="Ctrl Val.Get"(reference=w560, error in=w559, "Control Name"="Valores") -> (reference out=w558:refnum<vi>, error out=w557:errorcluster, "Get Control Value Variant"=w556:variant)  [unwired: 1 in, 1 out]
                  }
                  frame #1 {
                    n260 = local write "Calibração"(FALSE ("Calibração")) -> ()
                  }
                }
              }
            }
            n261 = local read "T_W_CLP"() -> (w441:dbl)
            n262 = local read "T_K_CLP"() -> (w442:dbl)
            n263 = local read "T_Ar_CLP"() -> (w448:dbl)
            n264 = Add(x=w383, y=273.15) -> (x+y=w388:dbl)
            n265 = local read "P_Lam [KPa]"() -> (w376:dbl)
            n266 = local read "SHD-PI-02-AUX"() -> (w366:dbl)
            n267 = Subtract(x=w375, y=w374) -> (x-y=w373:dbl)
            n268 = local read "SKM-NC-CV-LAM"() -> (w411:bool)
            n269 = local read "SKM-NC-CV-COR"() -> (w412:bool)
            n270 = Multiply(x=w388, y=0.287058 ("x")) -> (x*y=w377:dbl)
            n271 = local read "T_mis [°C]"() -> (w392:dbl)
            n272 = local read "Q_W [m³/s]"() -> (w415:dbl)
            n273 = Subtract(x=1200.0, y=w452) -> (x-y=w451:dbl)
            n274 = local read "M_K_CLP"() -> (w416:dbl)
            n275 = Subtract(x=60.0, y=w433) -> (x-y=w432:dbl)
            n276 = Subtract(x=60.0, y=w437) -> (x-y=w438:dbl)
            n277 = Subtract(x=60.0, y=w444) -> (x-y=w445:dbl)
            n278 = local read "T_W [°C]"() -> (w409:dbl)
            n279 = local read "T_K [°C]"() -> (w410:dbl)
            n280 = local read "T_W [°C]"() -> (w371:dbl)
            n281 = Divide(x=w377, y=w376) -> (x/y=w382:dbl)
            n282 = Divide(x=w451, y=4095.0) -> (x/y=w450:dbl)
            n283 = Divide(x=w432, y=4095.0) -> (x/y=w431:dbl)
            n284 = Divide(x=w438, y=4095.0) -> (x/y=w439:dbl)
            n285 = Divide(x=w445, y=4095.0) -> (x/y=w446:dbl)
            n286 = call "Curva_Densidade.vi"("P_Ar [KPa]"=w403, "T_Ar [°C]"=w394, "T_K [°C]"=w392, "T_W [°C]"=w392) -> ("Rho_Ar [Kg/m³]"=→"Rho_Ar [kg/m³]":dbl, "Rho_K [Kg/m³]"=→"Rho_K [Kg/m³]":dbl, "Rho_W [Kg/m³]"=→"Rho_W [Kg/m³]":dbl)
            n287 = Multiply(x=w367, y=w382) -> (x*y=w386:dbl)
            n288 = call "Calculo_Velocidade.vi"("SKM-NC-CV-COR"=w412, "SKM-NC-CV-LAM"=w411, "SKM-FIC-AR-COR [Kg/s]"=w413, "M_Lam [Kg/h]"=w379, "Q_W [m³/s]"=w415, "M_K [Kg/s]"=w416, "T_W [°C]"=w409, "T_K [°C]"=w410, "T_Ar [°C]"=w383, "Diametro_Tubo [m]"=0.0234, "M_Manual"="automatico/M_manual", "M_Lam_Manual [Kg/h]"=w367, "P_lam [KPa]"=w373, "P_Bar [KPa]"=w374, "SKM-AI-KF_COR"=w414) -> ("T_Mistura [K]"=→"T_mis [°C]":dbl, "JK [m/s]"=→"JK [m/s]":dbl, "JW [m/s]"=→"JW [m/s]":dbl, "JL [m/s]"=→"JL [m/s]":dbl)  [unwired: 8 in, 1 out]
            n289 = Multiply(x=w454, y=w450) -> (x*y=w449:dbl)
            n290 = Divide(x=w386, y=3600.0) -> (x/y=w385:dbl)
            n291 = Multiply(x=w441, y=w431) -> (x*y=w430:dbl)
            n292 = Multiply(x=w442, y=w439) -> (x*y=w440:dbl)
            n293 = Multiply(x=w448, y=w446) -> (x*y=w447:dbl)
            n294 = Add(x=273.15 ("y"), y=w371) -> (x+y=w369:dbl)
            n295 = call "JG.vi"("T_W[°C]"=w369, "SHD-PI-02"=w366, "M_manual"=w367) -> ("JG [m/s]"=→"JG [m/s]":dbl)
            n296 = Divide(x=w385, y=0.000430053) -> (x/y=→"JG_Lam [m/s]":dbl)
            n297 = Add(x=w449, y=w452) -> (x+y=→"P_Lam [KPa]":dbl)
            n298 = Add(x=w430, y=w433) -> (x+y=→"T_W [°C]":dbl)
            n299 = Add(x=w440, y=w437) -> (x+y=→"T_K [°C]":dbl)
            n300 = Add(x=w447, y=w444) -> (x+y=→"T_Ar [°C]":dbl)
            n301 = Build Array("Teste", "Alinhamento", "Teste 234") -> (w523:bool[])
            n302 = Boolean Array To Number(Boolean array=w523) -> (number=w522:u32)
            n303 = case shown="1" w522 {
              tunnel: [w594 "stop VI" w2002 w2014] -> w485
              tunnel: [w587 w638 FALSE ("alarme") FALSE ("alarme")] -> w489
              tunnel: w483 -> [_ w629 _ _]
              frame 0, Default {
                w595 = FALSE ("Medição")
                w592 = T5."Disabled and Grayed Out" ("Disabled")
                w593 = T5."Disabled and Grayed Out" ("Disabled")
                w596 = TRUE
                w597 = FALSE
                # "Válvulas de entrada e saída ABERTAS"
                # "Cálculos da Medidas de pressão"
                n304 = local write "Gravar teste"(w595) -> ()
                n305 = local write "SIT-CV-AT"(FALSE ("SIT-CV-AT")) -> ()
                n306 = local write "Medição"(w595) -> ()
                n307 = property on="T azul" class="Bool (strict)"("Visible"=w597) -> ()  [unwired: 2 in, 2 out]
                n308 = property on="cano azul v" class="Bool (strict)"("Visible"=w597) -> ()  [unwired: 2 in, 2 out]
                n309 = property on="cano azul h" class="Bool (strict)"("Visible"=w597) -> ()  [unwired: 2 in, 2 out]
                n310 = property on="cano verde" class="Bool (strict)"("Visible"=w597) -> ()  [unwired: 2 in, 2 out]
                n311 = property on="cano amarelo" class="Bool (strict)"("Visible"=w597) -> ()  [unwired: 2 in, 2 out]
                n312 = local write "caixinha"(TRUE ("caixinha")) -> ()
                n313 = property on="cano roxo h" class="Bool (strict)"("Visible"=w596) -> ()  [unwired: 2 in, 2 out]
                n314 = property on="T roxo" class="Bool (strict)"("Visible"=w596) -> ()  [unwired: 2 in, 2 out]
                n315 = property on="cano roxo" class="Bool (strict)"("Visible"=w596) -> ()  [unwired: 2 in, 2 out]
                n316 = property on="Documentação" class="Bool (strict)"("DisabledEnum"=T5."Enabled" ("Disabled")) -> ()  [unwired: 2 in, 2 out]
                n317 = property on="Teste 234" class="Bool (strict)"("DisabledEnum"=T5."Enabled" ("Disabled")) -> ()  [unwired: 2 in, 2 out]
                n318 = property on="Alinhamento" class="Bool (strict)"("DisabledEnum"=T5."Enabled" ("Disabled")) -> ()  [unwired: 2 in, 2 out]
                n319 = property on="Calibração" class="Bool (strict)"("DisabledEnum"=T5."Enabled" ("Disabled")) -> ()  [unwired: 2 in, 2 out]
                n320 = property on="Teste" class="Bool (strict)"("DisabledEnum"=T5."Enabled" ("Disabled")) -> ()  [unwired: 2 in, 2 out]
                n321 = case shown="True" "Documentação" {
                  frame False {
                  }
                  frame True {
                    n322 = stacked-sequence {
                      frame #0 {
                        n323 = Current VI's Path() -> (path=w619:path)
                        n324 = Strip Path(path=w619) -> (stripped path=w618:path)  [unwired: 1 out]
                        n325 = Build Path(base path=w618, name or relative path="documentos.vi") -> (appended path=w616:path)
                        n326 = Open VI Reference(vi path=w616) -> (vi reference=w615:refnum<vi>)  [unwired: 5 in, 1 out]
                        n327 = invoke class="VI" method="Run VI"(reference=w615, "Wait until done"=FALSE ("Wait Until Done"), "Auto Dispose Ref"=FALSE ("Auto Dispose Reference")) -> ()  [unwired: 2 in, 5 out]
                      }
                      frame #1 {
                        n328 = local write "Documentação"(FALSE ("Documentação")) -> ()
                      }
                    }
                  }
                }
                n329 = property on="Parar Teste" class="Bool"("DisabledEnum"=T5."Disabled and Grayed Out" ("Disabled")) -> ()  [unwired: 2 in, 2 out]
                n330 = property on="Medição" class="Bool (strict)"("DisabledEnum"=w593) -> ()  [unwired: 2 in, 2 out]
                n331 = property on="caixinha" class="Bool (strict)"("DisabledEnum"=T5."Disabled and Grayed Out" ("Disabled")) -> ()  [unwired: 2 in, 2 out]
                n332 = property on="Gravar teste" class="Bool (strict)"("DisabledEnum"=w592) -> ()  [unwired: 2 in, 2 out]
                n333 = local write "P2-LIMITE"(TRUE ("Teste")) -> ()
                n334 = property on="Cluster" class="Clust (strict)"("DisabledEnum"=w593) -> ()  [unwired: 2 in, 2 out]
                n335 = property on="Cluster 2" class="Clust (strict)"("DisabledEnum"=w592) -> ()  [unwired: 2 in, 2 out]
                n336 = case shown="False" FALSE {
                  tunnel: [w598 w605] -> w566
                  tunnel: [w599 w604] -> w569
                  frame False {
                    n337 = local read "Valores"() -> (w600:T4)
                    n338 = call "Calculo_Pressao.vi"("X2"="Pressão02-CLP[0-4095]", "Valores"=w600, "Calibrador"=TRUE, "X"="Pressão01_CLP[0-4095]") -> ("Pressao 2"=w598:dbl, "Pressao"=w599:dbl)  [unwired: 2 in]
                  }
                  frame True {
                    n339 = call "TESTE_PRESSAO_OFICINA.vi"() -> ("Pressão 2"=w605:dbl, "Pressão 1"=w604:dbl)  [unwired: 10 in]
                  }
                }
                "PI-02- Bruto" <- w566
                n340 = flat-sequence {
                  frame #0 {
                    n341 = local write "SKS-NC-CV-003"(TRUE ("SKS-NC-CV-003")) -> ()
                  }
                  frame #1 {
                    w607 = FALSE ("SKT 2")
                    n342 = local write "SIT-CV-ST"(w607) -> ()
                    n343 = local write "SIT-CV-ST"(w607) -> ()
                  }
                  frame #2 {
                    n344 = local write "SIT-NC-CV-001"(TRUE ("SIT-NC-CV-001")) -> ()
                  }
                  frame #3 {
                    n345 = Wait (ms)(milliseconds to wait=u32 500) -> ()  [unwired: 1 out]
                  }
                  frame #4 {
                    n346 = local write "SKS-NC-CV-002"(FALSE ("SKS-NC-CV-002")) -> ()
                  }
                  frame #5 {
                    n347 = Wait (ms)(milliseconds to wait=u32 500) -> ()  [unwired: 1 out]
                  }
                  frame #6 {
                    n348 = local write "SIT-NC-CV-002"(FALSE ("SIT-NC-CV-002")) -> ()
                  }
                }
                n349 = local read "P_Bar [KPa]"() -> (w568:dbl)
                n350 = Add(x=w566, y=w568) -> (x+y=w572:dbl)
                n351 = Build Array(w569, w572) -> (w571:dbl[])
                n352 = local write "SHD-PI-02-Ind."(w572) -> ()
                n353 = local write "SHD-PI-01-Ind."(w569) -> ()
                n354 = local write "SHD-PI-02"(w572) -> ()
                n355 = local write "SHD-PI-01"(w569) -> ()
                n356 = Build Array(w571) -> (→"Gráfico":dbl[][])
                n357 = local read "SHD-PI-02"() -> (w584:dbl)
                n358 = local read "SHD-PI-01"() -> (w585:dbl)
                n359 = call "Media_pressao.vi"("Pressao 2"=w584, "Pressao 1"=w585) -> ("Diferenca pressao"=w582:dbl, "Pressao media"=w583:dbl)  [unwired: 8 in]
                "P1-P2" <- w582
                n360 = Divide(x=w582, y=w583) -> (x/y=w590:dbl)
                n361 = Absolute Value(x=w590) -> (abs(x)=w589:dbl)
                n362 = Greater?(x=w589, y=0.05) -> (0:w588:bool)
                n363 = case shown="True" w588 {
                  tunnel: [FALSE TRUE] -> w587
                  frame False {
                    n364 = local write "JANELA"(FALSE ("JANELA")) -> ()
                    n365 = property on="HELP-SIT" class="Bool"("Visible"=FALSE) -> ()  [unwired: 2 in, 2 out]
                  }
                  frame True {
                    n366 = property on="HELP-SIT" class="Bool"("Visible"=TRUE) -> ()  [unwired: 2 in, 2 out]
                  }
                }
                n367 = local read "stop VI"() -> (w594:bool)
              }
              frame 1 {
                w637 = T5."Enabled" ("Disabled")
                w645 = FALSE
                w644 = TRUE
                # "Cálculos da Medidas de pressão"
                n368 = property on="T azul" class="Bool (strict)"("Visible"=w644) -> ()  [unwired: 2 in, 2 out]
                n369 = property on="cano azul v" class="Bool (strict)"("Visible"=w644) -> ()  [unwired: 2 in, 2 out]
                n370 = property on="cano azul h" class="Bool (strict)"("Visible"=w644) -> ()  [unwired: 2 in, 2 out]
                n371 = property on="cano verde" class="Bool (strict)"("Visible"=w644) -> ()  [unwired: 2 in, 2 out]
                n372 = property on="cano amarelo" class="Bool (strict)"("Visible"=w644) -> ()  [unwired: 2 in, 2 out]
                n373 = property on="cano roxo h" class="Bool (strict)"("Visible"=w645) -> ()  [unwired: 2 in, 2 out]
                n374 = property on="cano roxo" class="Bool (strict)"("Visible"=w645) -> ()  [unwired: 2 in, 2 out]
                n375 = property on="T roxo" class="Bool (strict)"("Visible"=w645) -> ()  [unwired: 2 in, 2 out]
                n376 = property on="Home" class="Bool (strict)"("Visible"=FALSE) -> ()  [unwired: 2 in, 2 out]
                n377 = flat-sequence {
                  frame #0 {
                    n378 = case shown="True" "P2-LIMITE" {
                      frame False {
                      }
                      frame True {
                        n379 = local read "Pressão01_CLP[0-4095]"() -> (w656:dbl)
                        n380 = local read "Pressão02-CLP[0-4095]"() -> (w655:dbl)
                        n381 = local read "Valores"() -> (w657:T4)
                        n382 = local read "P_Bar [KPa]"() -> (w659:dbl)
                        n383 = call "Calculo_Pressao.vi"("X2"=w655, "Valores"=w657, "Calibrador"=TRUE, "X"=w656) -> ("Pressao 2"=w660:dbl)  [unwired: 2 in, 1 out]
                        n384 = Add(x=w660, y=w659) -> (x+y=→"SHD-PI-02-AUX":dbl)
                        n385 = local write "P2-LIMITE"(FALSE ("Boolean")) -> ()
                      }
                    }
                  }
                  frame #1 {
                    n386 = local write "SKS-NC-CV-002"(TRUE ("SKS-NC-CV-002")) -> ()
                    n387 = local write "SIT-NC-CV-002"(TRUE ("SIT-NC-CV-002")) -> ()
                    n388 = local write "SIT-NC-CV-001"(FALSE ("SIT-NC-CV-001")) -> ()
                  }
                  frame #2 {
                    n389 = local write "SKS-NC-CV-003"(FALSE ("SKS-NC-CV-003")) -> ()
                  }
                  frame #3 {
                    w666 = TRUE ("SKT 1")
                    n390 = local write "SIT-CV-ST"(w666) -> ()
                    n391 = local write "SIT-CV-ST"(w666) -> ()
                  }
                }
                n392 = property on="Cluster" class="Clust (strict)"("DisabledEnum"=w637) -> ()  [unwired: 2 in, 2 out]
                n393 = property on="Cluster 2" class="Clust (strict)"("DisabledEnum"=w637) -> ()  [unwired: 2 in, 2 out]
                n394 = property on="Teste" class="Bool (strict)"("DisabledEnum"=T5."Disabled and Grayed Out" ("Disabled")) -> ()  [unwired: 2 in, 2 out]
                n395 = property on="Medição" class="Bool (strict)"("DisabledEnum"=w637) -> ()  [unwired: 2 in, 2 out]
                n396 = property on="Alinhamento" class="Bool (strict)"("DisabledEnum"=T5."Disabled and Grayed Out" ("Disabled")) -> ()  [unwired: 2 in, 2 out]
                n397 = property on="Teste 234" class="Bool (strict)"("DisabledEnum"=T5."Disabled and Grayed Out" ("Disabled")) -> ()  [unwired: 2 in, 2 out]
                n398 = property on="Gravar teste" class="Bool (strict)"("DisabledEnum"=T5."Enabled" ("Disabled")) -> ()  [unwired: 2 in, 2 out]
                n399 = property on="Home" class="Bool (strict)"("DisabledEnum"=T5."Enabled" ("Disabled")) -> ()  [unwired: 2 in, 2 out]
                n400 = property on="Calibração" class="Bool (strict)"("DisabledEnum"=T5."Disabled and Grayed Out" ("Disabled")) -> ()  [unwired: 2 in, 2 out]
                n401 = case shown="True" "Medição" {
                  tunnel: w629 -> [_ w808]
                  frame False {
                    n402 = local read "Gravar teste"() -> (w679:bool)
                    n403 = case shown="True" w679 {
                      frame False {
                      }
                      frame True {
                        n404 = stacked-sequence {
                          frame #0 {
                            w688 = T5."Disabled and Grayed Out" ("Disabled")
                            n405 = case shown="False" FALSE {
                              tunnel: [w693 w699] -> w687
                              tunnel: [w692 w698] -> w682
                              frame False {
                                n406 = local read "Pressão02-CLP[0-4095]"() -> (w696:dbl)
                                n407 = local read "Pressão01_CLP[0-4095]"() -> (w697:dbl)
                                n408 = local read "Valores"() -> (w694:T4)
                                n409 = call "Calculo_Pressao.vi"("X2"=w696, "Valores"=w694, "Calibrador"=TRUE, "X"=w697) -> ("Pressao 2"=w692:dbl, "Pressao"=w693:dbl)  [unwired: 2 in]
                              }
                              frame True {
                                n410 = call "TESTE_PRESSAO_OFICINA.vi"() -> ("Pressão 2"=w698:dbl, "Pressão 1"=w699:dbl)  [unwired: 10 in]
                              }
                            }
                            n411 = local write "SIT-CV-AT"(FALSE ("SKT 3")) -> ()
                            n412 = local read "P_Bar [KPa]"() -> (w681:dbl)
                            n413 = Add(x=w682, y=w681) -> (x+y=w680:dbl)
                            n414 = property on="Cluster 2" class="Clust (strict)"("DisabledEnum"=w688) -> ()  [unwired: 2 in, 2 out]
                            n415 = local write "SHD-PI-01-Ind."(w687) -> ()
                            n416 = local write "SHD-PI-01"(w687) -> ()
                            n417 = property on="Gravar teste" class="Bool (strict)"("DisabledEnum"=w688) -> ()  [unwired: 2 in, 2 out]
                            n418 = local write "SHD-PI-02-Ind."(w680) -> ()
                            n419 = local write "SHD-PI-02"(w680) -> ()
                            n420 = Build Array(w687, w680) -> (w686:dbl[])
                            n421 = local read "Cluster 2"() -> (w690:T2)
                            n422 = Build Array(w686) -> (w685:dbl[][])
                            n423 = local write "Gráfico"(w685) -> ()
                            n424 = Wait (ms)(milliseconds to wait=u32 1000) -> ()  [unwired: 1 out]
                            n425 = Unbundle By Name(w690) -> ("Formato"=w689:enum32{"Item 0", "Item 1"})
                            n426 = case shown="\"Item 1\"" w689 {
                              frame "Item 0", Default {
                                (unwired) FALSE
                                n427 = local read "JW_aux"() -> (w708:dbl)
                                n428 = local read "JK_aux"() -> (w707:dbl)
                                n429 = local read "JG_aux"() -> (w706:dbl)
                                n430 = local read "Vazio"() -> (w745:dbl)
                                n431 = local read "Vazio Misto erro"() -> (w744:dbl)
                                n432 = local read "Hw"() -> (w743:dbl)
                                n433 = local read "Hw Misto erro"() -> (w742:dbl)
                                n434 = local read "Hk"() -> (w741:dbl)
                                n435 = local read "Hk  Misto erro"() -> (w740:dbl)
                                n436 = local read "Vazio  Free"() -> (w739:dbl)
                                n437 = local read "Vazio Free erro"() -> (w738:dbl)
                                n438 = local read "Hw Free"() -> (w737:dbl)
                                n439 = local read "Hw Free erro"() -> (w736:dbl)
                                n440 = local read "Hk Free"() -> (w735:dbl)
                                n441 = local read "Hk Free erro"() -> (w734:dbl)
                                n442 = local read "Vazio Mer"() -> (w733:dbl)
                                n443 = local read "Vazio Mer erro"() -> (w732:dbl)
                                n444 = local read "Hw Mer"() -> (w731:dbl)
                                n445 = local read "Hw Mer erro"() -> (w730:dbl)
                                n446 = local read "Hk Mer"() -> (w729:dbl)
                                n447 = local read "Hk Mer erro"() -> (w728:dbl)
                                n448 = Build Array(w708, w707, w706, w745, w744, w743, w742, w741, w740, w739, w738, w737, w736, w735, w734, w733, w732, w731, w730, w729, w728) -> (w727:dbl[])
                                n449 = local read "Altura Líquido"() -> (w751:dbl)
                                n450 = local read "Altura Liquido erro"() -> (w750:dbl)
                                n451 = local read "Altura Água"() -> (w749:dbl)
                                n452 = local read "Altura Água erro"() -> (w748:dbl)
                                n453 = local read "Altura Kerosene"() -> (w747:dbl)
                                n454 = local read "Altura Kerosene erro"() -> (w746:dbl)
                                n455 = local read "Cluster 2"() -> (w754:T2)
                                n456 = local read "Lk"() -> (w722:dbl)
                                n457 = local read "Lw"() -> (w723:dbl)
                                n458 = local read "Ll"() -> (w724:dbl)
                                n459 = Unbundle By Name(w754) -> ("File Path Control"=w715:path)
                                n460 = local read "JW_Title"() -> (w711:string)
                                n461 = local read "JG_Title"() -> (w709:string)
                                n462 = local read "JK_Title"() -> (w710:string)
                                n463 = Build Array(w751, w750, w749, w748, w747, w746, w724, w723, w722) -> (w726:dbl[])
                                n464 = Path To String(path=w715) -> (string=w714:string)
                                n465 = local read "SHD-PI-02-AUX"() -> (w753:dbl)
                                n466 = local read "JG_Lam [m/s]"() -> (w717:dbl)
                                n467 = local read "P_Bar [KPa]"() -> (w721:dbl)
                                n468 = local read "P_Lam [KPa]"() -> (w716:dbl)
                                n469 = local read "SHD-PI-01"() -> (w752:dbl)
                                n470 = local read "T_W [°C]"() -> (w720:dbl)
                                n471 = local read "T_Atm [°C]"() -> (w718:dbl)
                                n472 = Concatenate Strings(w714, "\\" ("string"), w711, "_" ("string"), w710, "_" ("string"), w709, ".txt" ("input 10")) -> (w713:string)
                                n473 = local read "T_K [°C]"() -> (w719:dbl)
                                n474 = local read "T_Ar [°C]"() -> (w705:dbl)
                                n475 = local read "M_manual"() -> (w700:dbl)
                                n476 = String To Path(string=w713) -> (path=w712:path)
                                n477 = Build Array(w752, w753, w721, w720, w719, w718, w717, w716, w705, w700) -> (w725:dbl[])
                                n478 = call "Salvar_txt.vi"("path"=w712, "Array"=w727, "Array 2"=w726, "Array 3"=w725) -> ()  [unwired: 2 in]
                              }
                              frame "Item 1" {
                                (unwired) FALSE
                                n479 = local read "SHD-PI-02-AUX"() -> (w776:dbl)
                                n480 = local read "JW_aux"() -> (w757:dbl)
                                n481 = local read "JK_aux"() -> (w756:dbl)
                                n482 = local read "JG_aux"() -> (w755:dbl)
                                n483 = local read "Vazio"() -> (w805:dbl)
                                n484 = local read "Vazio Misto erro"() -> (w804:dbl)
                                n485 = local read "Hw"() -> (w803:dbl)
                                n486 = local read "Hw Misto erro"() -> (w802:dbl)
                                n487 = local read "Hk"() -> (w801:dbl)
                                n488 = local read "Hk  Misto erro"() -> (w800:dbl)
                                n489 = local read "Vazio  Free"() -> (w799:dbl)
                                n490 = local read "Vazio Free erro"() -> (w798:dbl)
                                n491 = local read "Hw Free"() -> (w797:dbl)
                                n492 = local read "Hw Free erro"() -> (w796:dbl)
                                n493 = local read "Hk Free"() -> (w795:dbl)
                                n494 = local read "Hk Free erro"() -> (w794:dbl)
                                n495 = local read "Vazio Mer"() -> (w793:dbl)
                                n496 = local read "Vazio Mer erro"() -> (w792:dbl)
                                n497 = local read "Hw Mer"() -> (w791:dbl)
                                n498 = local read "Hw Mer erro"() -> (w790:dbl)
                                n499 = local read "Hk Mer"() -> (w789:dbl)
                                n500 = local read "Hk Mer erro"() -> (w788:dbl)
                                n501 = local read "Altura Líquido"() -> (w787:dbl)
                                n502 = local read "Altura Liquido erro"() -> (w786:dbl)
                                n503 = local read "Altura Água"() -> (w785:dbl)
                                n504 = local read "Altura Água erro"() -> (w784:dbl)
                                n505 = local read "Altura Kerosene"() -> (w783:dbl)
                                n506 = local read "Altura Kerosene erro"() -> (w782:dbl)
                                n507 = local read "P_Bar [KPa]"() -> (w775:dbl)
                                n508 = local read "SHD-PI-01"() -> (w777:dbl)
                                n509 = local read "JG_Lam [m/s]"() -> (w771:dbl)
                                n510 = local read "P_Lam [KPa]"() -> (w770:dbl)
                                n511 = local read "T_W [°C]"() -> (w774:dbl)
                                n512 = local read "T_Atm [°C]"() -> (w772:dbl)
                                n513 = local read "T_K [°C]"() -> (w773:dbl)
                                n514 = local read "Lk"() -> (w778:dbl)
                                n515 = local read "Lw"() -> (w779:dbl)
                                n516 = local read "Ll"() -> (w780:dbl)
                                n517 = local read "Cluster 2"() -> (w769:T2)
                                n518 = Build Array(w757, w756, w755, w805, w804, w803, w802, w801, w800, w799, w798, w797, w796, w795, w794, w793, w792, w791, w790, w789, w788, w787, w786, w785, w784, w783, w782, w780, w779, w778, w777, w776, w775, w774, w773, w772, w771, w770) -> (w781:dbl[])
                                n519 = Unbundle By Name(w769) -> ("File Path Control"=w768:path)
                                n520 = local read "JW_Title"() -> (w765:string)
                                n521 = local read "JG_Title"() -> (w763:string)
                                n522 = local read "JK_Title"() -> (w764:string)
                                n523 = Path To String(path=w768) -> (string=w767:string)
                                n524 = Concatenate Strings(w767, "\\" ("string"), w765, "_" ("string"), w764, "_" ("string"), w763, ".xlsx" ("input 10")) -> (w766:string)
                                n525 = String To Path(string=w766) -> (path=w758:path)
                                n526 = call "Salvar_excel.vi"("Array"=w781, "Filename"=w758) -> ()  [unwired: 10 in]
                              }
                            }
                          }
                          frame #1 {
                            w806 = T5."Enabled" ("Disabled")
                            n527 = local write "Gravar teste"(FALSE ("Gravar teste")) -> ()
                            n528 = property on="Cluster 2" class="Clust (strict)"("DisabledEnum"=w806) -> ()  [unwired: 2 in, 2 out]
                            n529 = property on="Gravar teste" class="Bool (strict)"("DisabledEnum"=w806) -> ()  [unwired: 2 in, 2 out]
                          }
                        }
                      }
                    }
                  }
                  frame True {
                    n530 = stacked-sequence {
                      tunnel: w808 -> [_ _ w841 w1050 _ _ _ w1831 _]
                      frame #0 {
                        n531 = local read "Cluster"() -> (w811:T3)
                        n532 = local write "SIT-CV-AT"(TRUE ("SKT 3")) -> ()
                        n533 = property on="Medição" class="Bool (strict)"("DisabledEnum"=T5."Disabled and Grayed Out" ("Disabled")) -> ()  [unwired: 2 in, 2 out]
                        n534 = Bundle By Name(cluster=w811, "Home"=FALSE) -> (w810:T3)
                        n535 = local write "Cluster"(w810) -> ()
                      }
                      frame #1 {
                        n536 = local read "Cluster"() -> (w824:T3)
                        n537 = Unbundle By Name(w824) -> ("Tempo P/ Medição"=w821:dbl)
                        n538 = Multiply(x=w821, y=1000.0) -> (x*y=w822:dbl)
                        n539 = Wait (ms)(milliseconds to wait=w822) -> ()  [unwired: 1 out]
                        n540 = for {
                          N: w821 -> [w835]
                          i -> [w834]
                          n541 = Subtract(x=w835, y=w834) -> (x-y=w833:i32)
                          n542 = Wait (ms)(milliseconds to wait=u32 1000) -> ()  [unwired: 1 out]
                          n543 = local read "Cluster"() -> (w837:T3)
                          n544 = Bundle By Name(cluster=w837, "Tempo Restante"=w833) -> (w836:T3)
                          n545 = local write "Cluster"(w836) -> ()
                        }
                        n546 = case shown="True" FALSE {
                          tunnel: [w830 w832] -> w820
                          tunnel: [w829 w831] -> w816
                          frame False {
                            n547 = local read "Pressão02-CLP[0-4095]"() -> (w827:dbl)
                            n548 = local read "Pressão01_CLP[0-4095]"() -> (w828:dbl)
                            n549 = local read "Valores"() -> (w825:T4)
                            n550 = call "Calculo_Pressao.vi"("X2"=w827, "Valores"=w825, "Calibrador"=TRUE, "X"=w828) -> ("Pressao 2"=w829:dbl, "Pressao"=w830:dbl)  [unwired: 2 in]
                          }
                          frame True {
                            n551 = call "TESTE_PRESSAO_OFICINA.vi"() -> ("Pressão 2"=w831:dbl, "Pressão 1"=w832:dbl)  [unwired: 10 in]
                          }
                        }
                        n552 = local read "P_Bar [KPa]"() -> (w815:dbl)
                        n553 = Add(x=w816, y=w815) -> (x+y=w814:dbl)
                        n554 = Build Array(w820, w814) -> (w819:dbl[])
                        n555 = local write "SHD-PI-01-Ind."(w820) -> ()
                        n556 = local write "SHD-PI-01"(w820) -> ()
                        n557 = Build Array(w819) -> (w818:dbl[][])
                        n558 = local write "Gráfico"(w818) -> ()
                        n559 = local write "SHD-PI-02"(w814) -> ()
                        n560 = local write "SHD-PI-02-Ind."(w814) -> ()
                      }
                      frame #2 {
                        n561 = flat-sequence {
                          tunnel: w841 -> [w845]
                          tunnel: [w845] -> w839
                          tunnel: [w847] -> w840
                          tunnel: w839 -> [w847]
                          tunnel: [w848] -> w842
                          tunnel: w840 -> [w848]
                          tunnel: [w850] -> w843
                          tunnel: w842 -> [w850]
                          tunnel: w843 -> [w860]
                          frame #0 {
                            n562 = local write "MWU1100"(i16 124 ("MWU1100")) -> ()
                          }
                          frame #1 {
                            n563 = Wait (ms)(milliseconds to wait=u32 150) -> ()  [unwired: 1 out]
                          }
                          frame #2 {
                            n564 = local write "MWU1100"(i16 100 ("MWU1100")) -> ()
                          }
                          frame #3 {
                            n565 = Wait (ms)(milliseconds to wait=u32 150) -> ()  [unwired: 1 out]
                          }
                          frame #4 {
                            n566 = invoke class="VI" method="Ctrl Val.Get"(reference=w860, "Control Name"="STRING") -> ("Get Control Value Variant"=w861:variant)  [unwired: 2 in, 3 out]
                            n567 = local read "STRING"() -> (w862:string)
                            n568 = Variant To Data(type=w862, Variant=w861) -> (data=w855:string)  [unwired: 1 in, 1 out]
                            n569 = One Button Dialog(message="O sensor já começou a subir, aguarde terminar as medidas", button name ("OK")="OK") -> ()  [unwired: 1 out]
                            n570 = String Subset(string=w855, offset (0)=0, length (rest)=3 ("length (rest)")) -> (substring=w857:string)
                            n571 = local write "STRING"(w855) -> ()
                            n572 = Equal?(x=w857, y="100") -> (x = y?=w854:bool)
                            n573 = case shown="False" w854 {
                              frame False {
                                n574 = flat-sequence {
                                frame #0 {
                                n575 = local write "MWU1100"(i16 11 ("MWU1100")) -> ()
                                }
                                frame #1 {
                                n576 = Wait (ms)(milliseconds to wait=u32 250) -> ()  [unwired: 1 out]
                                }
                                frame #2 {
                                n577 = local write "MWU1100"(i16 100 ("MWU1100")) -> ()
                                }
                                }
                              }
                              frame True {
                              }
                            }
                            n578 = while {
                              shift-right: [w877] -> _
                              shift-left: 0.0 -> [w882]
                              tunnel: w860 -> [w876]
                              stop <- w884 stop-if-true
                              n579 = flat-sequence {
                                tunnel: [w888] -> w883
                                tunnel: w882 -> [w888]
                                tunnel: w876 -> [w887]
                                tunnel: [w887] -> w875
                                tunnel: w883 -> [w891]
                                tunnel: [w891] -> w881
                                tunnel: w875 -> [w890]
                                tunnel: [w890] -> w874
                                tunnel: [w893] -> w885
                                tunnel: w881 -> [w899]
                                tunnel: [w896] -> w880
                                tunnel: w874 -> [w894]
                                tunnel: [w894] -> w873
                                tunnel: [w893] -> w870
                                tunnel: w880 -> [w969]
                                tunnel: [w969] -> w879
                                tunnel: w873 -> [w968]
                                tunnel: [w968] -> w872
                                tunnel: w870 -> [w967]
                                tunnel: [w967] -> w869
                                tunnel: w879 -> [w973]
                                tunnel: [w973] -> w878
                                tunnel: w872 -> [w972]
                                tunnel: [w972] -> w871
                                tunnel: w869 -> [w971]
                                tunnel: [w971] -> w868
                                tunnel: [w983] -> w886
                                tunnel: w878 -> [w980]
                                tunnel: [w978] -> w877
                                tunnel: w871 -> [w976]
                                tunnel: w868 -> [w975]
                                frame #0 {
                                n580 = local write "MWU1100"(i16 123 ("MWU1100")) -> ()
                                }
                                frame #1 {
                                n581 = Wait (ms)(milliseconds to wait=u32 250) -> ()  [unwired: 1 out]
                                }
                                frame #2 {
                                n582 = case shown="False" FALSE {
                                tunnel: [w916 w966] -> w906
                                tunnel: w894 -> [w915 _]
                                frame False {
                                n583 = invoke class="VI" method="Ctrl Val.Get"(reference=w915, "Control Name"="STRING") -> ("Get Control Value Variant"=w918:variant)  [unwired: 2 in, 3 out]
                                n584 = case shown="False" FALSE {
                                tunnel: [w924 w926] -> w911
                                tunnel: [w923 w925] -> w907
                                frame False {
                                n585 = local read "Pressão02-CLP[0-4095]"() -> (w921:dbl)
                                n586 = local read "Pressão01_CLP[0-4095]"() -> (w922:dbl)
                                n587 = local read "Valores"() -> (w919:T4)
                                n588 = call "Calculo_Pressao.vi"("X2"=w921, "Valores"=w919, "Calibrador"=TRUE, "X"=w922) -> ("Pressao 2"=w923:dbl, "Pressao"=w924:dbl)  [unwired: 2 in]
                                }
                                frame True {
                                n589 = call "TESTE_PRESSAO_OFICINA.vi"() -> ("Pressão 2"=w925:dbl, "Pressão 1"=w926:dbl)  [unwired: 10 in]
                                }
                                }
                                n590 = local read "STRING"() -> (w917:string)
                                n591 = Variant To Data(type=w917, Variant=w918) -> (data=w916:string)  [unwired: 1 in, 1 out]
                                n592 = local read "P_Bar [KPa]"() -> (w908:dbl)
                                n593 = Add(x=w907, y=w908) -> (x+y=w909:dbl)
                                n594 = local write "STRING"(w916) -> ()
                                n595 = Build Array(w911, w909) -> (w912:dbl[])
                                n596 = local write "SHD-PI-02-Ind."(w909) -> ()
                                n597 = local write "SHD-PI-02"(w909) -> ()
                                n598 = local write "SHD-PI-01-Ind."(w911) -> ()
                                n599 = local write "SHD-PI-01"(w911) -> ()
                                n600 = Build Array(w912) -> (w913:dbl[][])
                                n601 = local write "Gráfico"(w913) -> ()
                                }
                                frame True {
                                n602 = local read "MWU2975"() -> (w949:i16)
                                n603 = local read "MWU2976"() -> (w950:i16)
                                n604 = local read "MWU2977"() -> (w951:i16)
                                n605 = local read "MWU2978"() -> (w952:i16)
                                n606 = local read "MWU2979"() -> (w953:i16)
                                n607 = local read "MWU2980"() -> (w954:i16)
                                n608 = local read "MWU2981"() -> (w955:i16)
                                n609 = local read "MWU2982"() -> (w956:i16)
                                n610 = local read "MWU2983"() -> (w957:i16)
                                n611 = local read "MWU2984"() -> (w958:i16)
                                n612 = local read "MWU2985"() -> (w959:i16)
                                n613 = local read "MWU2986"() -> (w960:i16)
                                n614 = local read "MWU2987"() -> (w961:i16)
                                n615 = call "Conversor-bin-hex.vi"("Numeric"=w949) -> ("hex integer string"=w927:string)  [unwired: 9 in, 1 out]
                                n616 = call "Conversor-bin-hex.vi"("Numeric"=w950) -> ("hex integer string"=w929:string, "hex integer string 2"=w928:string)  [unwired: 9 in]
                                n617 = call "Conversor-bin-hex.vi"("Numeric"=w951) -> ("hex integer string"=w931:string, "hex integer string 2"=w930:string)  [unwired: 9 in]
                                n618 = call "Conversor-bin-hex.vi"("Numeric"=w952) -> ("hex integer string"=w933:string, "hex integer string 2"=w932:string)  [unwired: 9 in]
                                n619 = call "Conversor-bin-hex.vi"("Numeric"=w953) -> ("hex integer string"=w935:string, "hex integer string 2"=w934:string)  [unwired: 9 in]
                                n620 = call "Conversor-bin-hex.vi"("Numeric"=w954) -> ("hex integer string"=w937:string, "hex integer string 2"=w936:string)  [unwired: 9 in]
                                n621 = call "Conversor-bin-hex.vi"("Numeric"=w955) -> ("hex integer string"=w939:string, "hex integer string 2"=w938:string)  [unwired: 9 in]
                                n622 = call "Conversor-bin-hex.vi"("Numeric"=w956) -> ("hex integer string"=w941:string, "hex integer string 2"=w940:string)  [unwired: 9 in]
                                n623 = call "Conversor-bin-hex.vi"("Numeric"=w957) -> ("hex integer string"=w943:string, "hex integer string 2"=w942:string)  [unwired: 9 in]
                                n624 = call "Conversor-bin-hex.vi"("Numeric"=w958) -> ("hex integer string"=w945:string, "hex integer string 2"=w944:string)  [unwired: 9 in]
                                n625 = call "Conversor-bin-hex.vi"("Numeric"=w959) -> ("hex integer string"=w947:string, "hex integer string 2"=w946:string)  [unwired: 9 in]
                                n626 = call "Conversor-bin-hex.vi"("Numeric"=w960) -> ("hex integer string"=w962:string, "hex integer string 2"=w948:string)  [unwired: 9 in]
                                n627 = call "Conversor-bin-hex.vi"("Numeric"=w961) -> ("hex integer string"=w964:string, "hex integer string 2"=w963:string)  [unwired: 9 in]
                                n628 = Concatenate Strings(w927, w928, w929, w930, w931, w932, w933, w934, w935, w936, w937, w938, w939, w940, w941, w942, w943, w944, w945, w946, w947, w948, w962, w963, w964) -> (w965:string)
                                n629 = call "string_inteira_carater.vi"("String in"=w965) -> ("String out"=w966:string)  [unwired: 10 in]
                                }
                                }
                                n630 = Add(x=w899, y=5.0) -> (x+y=w896:dbl)
                                n631 = local read "Cluster"() -> (w898:T3)
                                n632 = Bundle By Name(cluster=w898, "Progresso Sensor"=w896) -> (w897:T3)
                                n633 = local write "Cluster"(w897) -> ()
                                n634 = Wait (ms)(milliseconds to wait=u32 4750) -> ()  [unwired: 1 out]
                                n635 = local write "String Caracter de Comunicação"(w906) -> ()
                                n636 = String Subset(string=w906, offset (0)=24, length (rest)=1 ("length (rest)")) -> (substring=w903:string)
                                n637 = Equal?(x=w903, y=">") -> (x = y?=w893:bool)
                                }
                                frame #3 {
                                n638 = local write "MWU1100"(i16 456 ("MWU1100")) -> ()
                                }
                                frame #4 {
                                n639 = Wait (ms)(milliseconds to wait=u32 250) -> ()  [unwired: 1 out]
                                }
                                frame #5 {
                                n640 = case shown="False" w975 {
                                frame False {
                                n641 = Wait (ms)(milliseconds to wait=u32 4750) -> ()  [unwired: 1 out]
                                }
                                frame True {
                                }
                                }
                                n642 = case shown="False" FALSE {
                                tunnel: [w997 w1010] -> w984
                                tunnel: w976 -> [w998 _]
                                frame False {
                                n643 = case shown="False" FALSE {
                                tunnel: [w1007 w1009] -> w995
                                tunnel: [w1006 w1008] -> w991
                                frame False {
                                n644 = local read "Pressão02-CLP[0-4095]"() -> (w1004:dbl)
                                n645 = local read "Pressão01_CLP[0-4095]"() -> (w1005:dbl)
                                n646 = local read "Valores"() -> (w1002:T4)
                                n647 = call "Calculo_Pressao.vi"("X2"=w1004, "Valores"=w1002, "Calibrador"=TRUE, "X"=w1005) -> ("Pressao 2"=w1006:dbl, "Pressao"=w1007:dbl)  [unwired: 2 in]
                                }
                                frame True {
                                n648 = call "TESTE_PRESSAO_OFICINA.vi"() -> ("Pressão 2"=w1008:dbl, "Pressão 1"=w1009:dbl)  [unwired: 10 in]
                                }
                                }
                                n649 = local read "P_Bar [KPa]"() -> (w992:dbl)
                                n650 = invoke class="VI" method="Ctrl Val.Get"(reference=w998, "Control Name"="STRING") -> ("Get Control Value Variant"=w1000:variant)  [unwired: 2 in, 3 out]
                                n651 = local read "STRING"() -> (w1001:string)
                                n652 = Add(x=w991, y=w992) -> (x+y=w990:dbl)
                                n653 = Build Array(w995, w990) -> (w994:dbl[])
                                n654 = Variant To Data(type=w1001, Variant=w1000) -> (data=w997:string)  [unwired: 1 in, 1 out]
                                n655 = local write "SHD-PI-02"(w990) -> ()
                                n656 = local write "SHD-PI-02-Ind."(w990) -> ()
                                n657 = local write "SHD-PI-01-Ind."(w995) -> ()
                                n658 = local write "SHD-PI-01"(w995) -> ()
                                n659 = local write "STRING"(w997) -> ()
                                n660 = Build Array(w994) -> (w993:dbl[][])
                                n661 = local write "Gráfico"(w993) -> ()
                                }
                                frame True {
                                n662 = local read "MWU2975"() -> (w1027:i16)
                                n663 = local read "MWU2976"() -> (w1026:i16)
                                n664 = local read "MWU2977"() -> (w1025:i16)
                                n665 = local read "MWU2978"() -> (w1024:i16)
                                n666 = local read "MWU2979"() -> (w1023:i16)
                                n667 = local read "MWU2980"() -> (w1022:i16)
                                n668 = local read "MWU2981"() -> (w1021:i16)
                                n669 = local read "MWU2982"() -> (w1020:i16)
                                n670 = local read "MWU2983"() -> (w1019:i16)
                                n671 = local read "MWU2984"() -> (w1018:i16)
                                n672 = local read "MWU2985"() -> (w1017:i16)
                                n673 = local read "MWU2986"() -> (w1016:i16)
                                n674 = local read "MWU2987"() -> (w1015:i16)
                                n675 = call "Conversor-bin-hex.vi"("Numeric"=w1027) -> ("hex integer string"=w1049:string)  [unwired: 9 in, 1 out]
                                n676 = call "Conversor-bin-hex.vi"("Numeric"=w1026) -> ("hex integer string"=w1047:string, "hex integer string 2"=w1048:string)  [unwired: 9 in]
                                n677 = call "Conversor-bin-hex.vi"("Numeric"=w1025) -> ("hex integer string"=w1045:string, "hex integer string 2"=w1046:string)  [unwired: 9 in]
                                n678 = call "Conversor-bin-hex.vi"("Numeric"=w1024) -> ("hex integer string"=w1043:string, "hex integer string 2"=w1044:string)  [unwired: 9 in]
                                n679 = call "Conversor-bin-hex.vi"("Numeric"=w1023) -> ("hex integer string"=w1041:string, "hex integer string 2"=w1042:string)  [unwired: 9 in]
                                n680 = call "Conversor-bin-hex.vi"("Numeric"=w1022) -> ("hex integer string"=w1039:string, "hex integer string 2"=w1040:string)  [unwired: 9 in]
                                n681 = call "Conversor-bin-hex.vi"("Numeric"=w1021) -> ("hex integer string"=w1037:string, "hex integer string 2"=w1038:string)  [unwired: 9 in]
                                n682 = call "Conversor-bin-hex.vi"("Numeric"=w1020) -> ("hex integer string"=w1035:string, "hex integer string 2"=w1036:string)  [unwired: 9 in]
                                n683 = call "Conversor-bin-hex.vi"("Numeric"=w1019) -> ("hex integer string"=w1033:string, "hex integer string 2"=w1034:string)  [unwired: 9 in]
                                n684 = call "Conversor-bin-hex.vi"("Numeric"=w1018) -> ("hex integer string"=w1031:string, "hex integer string 2"=w1032:string)  [unwired: 9 in]
                                n685 = call "Conversor-bin-hex.vi"("Numeric"=w1017) -> ("hex integer string"=w1029:string, "hex integer string 2"=w1030:string)  [unwired: 9 in]
                                n686 = call "Conversor-bin-hex.vi"("Numeric"=w1016) -> ("hex integer string"=w1014:string, "hex integer string 2"=w1028:string)  [unwired: 9 in]
                                n687 = call "Conversor-bin-hex.vi"("Numeric"=w1015) -> ("hex integer string"=w1012:string, "hex integer string 2"=w1013:string)  [unwired: 9 in]
                                n688 = Concatenate Strings(w1049, w1048, w1047, w1046, w1045, w1044, w1043, w1042, w1041, w1040, w1039, w1038, w1037, w1036, w1035, w1034, w1033, w1032, w1031, w1030, w1029, w1028, w1014, w1013, w1012) -> (w1011:string)
                                n689 = call "string_inteira_carater.vi"("String in"=w1011) -> ("String out"=w1010:string)  [unwired: 10 in]
                                }
                                }
                                n690 = Add(x=5.0, y=w980) -> (x+y=w978:dbl)
                                n691 = local read "Cluster"() -> (w982:T3)
                                n692 = Bundle By Name(cluster=w982, "Progresso Sensor"=w978) -> (w981:T3)
                                n693 = local write "Cluster"(w981) -> ()
                                n694 = local write "String Caracter de Comunicação"(w984) -> ()
                                n695 = String Subset(string=w984, offset (0)=24, length (rest)=1 ("length (rest)")) -> (substring=w987:string)
                                n696 = Equal?(x=w987, y=">") -> (x = y?=w983:bool)
                                }
                              }
                              n697 = Or(x=w886, y=w885) -> (x .or. y?=w884:bool)
                            }
                          }
                        }
                      }
                      frame #3 {
                        n698 = stacked-sequence {
                          tunnel: w1050 -> [w1053 _ _ _ _]
                          frame #0 {
                            n699 = invoke class="VI" method="Ctrl Val.Get"(reference=w1053, "Control Name"="STRING") -> ("Get Control Value Variant"=w1055:variant)  [unwired: 2 in, 3 out]
                            n700 = local read "STRING"() -> (w1054:string)
                            n701 = Variant To Data(type=w1054, Variant=w1055) -> (data=w1051:string)  [unwired: 1 in, 1 out]
                            "STRING" <- w1051
                            n702 = case shown="False" FALSE {
                              tunnel: [w1179 w1224] -> w1057
                              tunnel: w1051 -> [w1178 _]
                              frame False {
                                n703 = case shown="True" TRUE {
                                tunnel: [w1181 w1183] -> w1179
                                tunnel: w1178 -> [w1181 _]
                                frame False {
                                }
                                frame True {
                                n704 = call "Conversor-bin-hex.vi"("Numeric"="MWU2975") -> ("hex integer string"=w1209:string)  [unwired: 9 in, 1 out]
                                n705 = call "Conversor-bin-hex.vi"("Numeric"="MWU2976") -> ("hex integer string"=w1207:string, "hex integer string 2"=w1208:string)  [unwired: 9 in]
                                n706 = call "Conversor-bin-hex.vi"("Numeric"="MWU2977") -> ("hex integer string"=w1205:string, "hex integer string 2"=w1206:string)  [unwired: 9 in]
                                n707 = call "Conversor-bin-hex.vi"("Numeric"="MWU2978") -> ("hex integer string"=w1203:string, "hex integer string 2"=w1204:string)  [unwired: 9 in]
                                n708 = call "Conversor-bin-hex.vi"("Numeric"="MWU2979") -> ("hex integer string"=w1201:string, "hex integer string 2"=w1202:string)  [unwired: 9 in]
                                n709 = call "Conversor-bin-hex.vi"("Numeric"="MWU2980") -> ("hex integer string"=w1199:string, "hex integer string 2"=w1200:string)  [unwired: 9 in]
                                n710 = call "Conversor-bin-hex.vi"("Numeric"="MWU2981") -> ("hex integer string"=w1197:string, "hex integer string 2"=w1198:string)  [unwired: 9 in]
                                n711 = call "Conversor-bin-hex.vi"("Numeric"="MWU2982") -> ("hex integer string"=w1195:string, "hex integer string 2"=w1196:string)  [unwired: 9 in]
                                n712 = call "Conversor-bin-hex.vi"("Numeric"="MWU2983") -> ("hex integer string"=w1193:string, "hex integer string 2"=w1194:string)  [unwired: 9 in]
                                n713 = call "Conversor-bin-hex.vi"("Numeric"="MWU2984") -> ("hex integer string"=w1191:string, "hex integer string 2"=w1192:string)  [unwired: 9 in]
                                n714 = call "Conversor-bin-hex.vi"("Numeric"="MWU2985") -> ("hex integer string"=w1189:string, "hex integer string 2"=w1190:string)  [unwired: 9 in]
                                n715 = call "Conversor-bin-hex.vi"("Numeric"="MWU2986") -> ("hex integer string"=w1187:string, "hex integer string 2"=w1188:string)  [unwired: 9 in]
                                n716 = call "Conversor-bin-hex.vi"("Numeric"="MWU2987") -> ("hex integer string"=w1184:string, "hex integer string 2"=w1185:string)  [unwired: 9 in]
                                n717 = Concatenate Strings(w1209, w1208, w1207, w1206, w1205, w1204, w1203, w1202, w1201, w1200, w1199, w1198, w1197, w1196, w1195, w1194, w1193, w1192, w1191, w1190, w1189, w1188, w1187, w1185, w1184) -> (w1183:string)
                                n718 = call "string_inteira_carater.vi"("String in"=w1183) -> ("String out"=→"String Caracter de Comunicação":string)  [unwired: 10 in]
                                }
                                }
                              }
                              frame True {
                                # "Tempo para perguntar \npara a placa freescale"
                                n719 = Type Cast(type=0, x="10") -> (*(type *) &x=w1241:i32)
                                n720 = Number To Hexadecimal String(2:w1241) -> (0:w1239:string)  [unwired: 1 in]
                                n721 = String Subset(string=w1239, length (rest)=4 ("length (rest)")) -> (substring=w1222:string)  [unwired: 1 in]
                                "Hexa p OPC" <- w1222
                                n722 = case shown="True" FALSE {
                                tunnel: [w1260 "String 1"] -> w1236
                                tunnel: [w1259 "String 2"] -> w1235
                                tunnel: [w1258 "String 3"] -> w1234
                                tunnel: [w1257 "String 4"] -> w1233
                                tunnel: [w1256 "String 5"] -> w1225
                                tunnel: [w1255 "String 6"] -> w1232
                                tunnel: [w1254 "String 7"] -> w1231
                                tunnel: [w1253 "String 8"] -> w1230
                                tunnel: [w1252 "String 9"] -> w1229
                                tunnel: [w1251 "String 10"] -> w1228
                                tunnel: [w1250 "String 11"] -> w1227
                                tunnel: [w1249 "String 12"] -> w1226
                                tunnel: w1222 -> [w1243 _]
                                tunnel: "Tempo de comunicação" -> [w1244 _]
                                frame False {
                                n723 = call "Simulador OPC.vi"("String vindo do labview"=w1243) -> ("String para CLP"=w1248:string)  [unwired: 6 in, 12 out]
                                n724 = call "Simulador CLP.vi"("String vindo do OPC"=w1248) -> ("String para Placa Freescale"=w1247:string)  [unwired: 9 in, 1 out]
                                n725 = call "FreeScale.vi"("milliseconds to wait"=w1244, "String para Freescale"=w1247) -> ("string Lido Freescale"=w1246:string)  [unwired: 8 in, 1 out]
                                n726 = call "Simulador CLP.vi"("String lido da placa"=w1246) -> ("String para OPC"=w1245:string)  [unwired: 9 in, 1 out]
                                n727 = call "Simulador OPC.vi"("String vindo do CLP"=w1245) -> ("String para labview 12"=w1262:string, "String para labview 11"=w1263:string, "String para labview 10"=w1264:string, "String para labview 9"=w1265:string, "String para labview 8"=w1266:string, "String para labview 7"=w1267:string, "String para labview 6"=w1268:string, "String para labview 1"=w1273:string, "String para labview 2"=w1272:string, "String para labview 3"=w1271:string, "String para labview 4"=w1270:string, "String para labview 5"=w1269:string)  [unwired: 6 in, 1 out]
                                n728 = Bundle("String para labview 1"=w1273, "String para labview 2"=w1272, "String para labview 3"=w1271, "String para labview 4"=w1270, "String para labview 5"=w1269, "String para labview 6"=w1268, "String para labview 7"=w1267, "String para labview 8"=w1266, "String para labview 9"=w1265, "String para labview 10"=w1264, "String para labview 11"=w1263, "String para labview 12"=w1262) -> (w1261:T7)  [unwired: 1 in]
                                n729 = Unbundle(w1261) -> ("String para labview 1"=w1260:string, "String para labview 2"=w1259:string, "String para labview 3"=w1258:string, "String para labview 4"=w1257:string, "String para labview 5"=w1256:string, "String para labview 6"=w1255:string, "String para labview 7"=w1254:string, "String para labview 8"=w1253:string, "String para labview 9"=w1252:string, "String para labview 10"=w1251:string, "String para labview 11"=w1250:string, "String para labview 12"=w1249:string)
                                }
                                frame True {
                                }
                                }
                                n730 = Wait (ms)(milliseconds to wait="Tempo de comunicação") -> ()  [unwired: 1 out]
                                n731 = Concatenate Strings(w1236, w1235, w1234, w1233, w1225, w1232, w1231, w1230, w1229, w1228, w1227, w1226) -> (w1224:string)
                              }
                            }
                            n732 = local read "Cluster"() -> (w1177:T3)
                            n733 = Bundle By Name(cluster=w1177, "Tempo Restante"=0.0 ("Tempo restante")) -> (w1176:T3)
                            n734 = String Subset(string=w1057, offset (0)=28, length (rest)=2 ("length (rest)")) -> (substring=w1063:string)
                            n735 = String Subset(string=w1057, offset (0)=30, length (rest)=2 ("length (rest)")) -> (substring=w1062:string)
                            n736 = String Subset(string=w1057, offset (0)=32, length (rest)=2 ("length (rest)")) -> (substring=w1061:string)
                            n737 = String Subset(string=w1057, offset (0)=34, length (rest)=2 ("length (rest)")) -> (substring=w1060:string)
                            n738 = String Subset(string=w1057, offset (0)=18, length (rest)=2 ("length (rest)")) -> (substring=w1075:string)
                            n739 = String Subset(string=w1057, offset (0)=20, length (rest)=2 ("length (rest)")) -> (substring=w1074:string)
                            n740 = String Subset(string=w1057, offset (0)=22, length (rest)=2 ("length (rest)")) -> (substring=w1073:string)
                            n741 = String Subset(string=w1057, offset (0)=24, length (rest)=2 ("length (rest)")) -> (substring=w1072:string)
                            n742 = String Subset(string=w1057, offset (0)=26, length (rest)=2 ("length (rest)")) -> (substring=w1071:string)
                            n743 = String Subset(string=w1057, offset (0)=8, length (rest)=2 ("length (rest)")) -> (substring=w1099:string)
                            n744 = String Subset(string=w1057, offset (0)=10, length (rest)=2 ("length (rest)")) -> (substring=w1098:string)
                            n745 = String Subset(string=w1057, offset (0)=12, length (rest)=2 ("length (rest)")) -> (substring=w1097:string)
                            n746 = String Subset(string=w1057, offset (0)=14, length (rest)=2 ("length (rest)")) -> (substring=w1096:string)
                            n747 = String Subset(string=w1057, offset (0)=16, length (rest)=2 ("length (rest)")) -> (substring=w1095:string)
                            n748 = local write "Cluster"(w1176) -> ()
                            n749 = Decimal String To Number(string=w1063) -> (number=w1069:i32)  [unwired: 2 in, 1 out]
                            n750 = Decimal String To Number(string=w1099) -> (number=w1085:i32)  [unwired: 2 in, 1 out]
                            n751 = Decimal String To Number(string=w1062) -> (number=w1068:i32)  [unwired: 2 in, 1 out]
                            n752 = Decimal String To Number(string=w1098) -> (number=w1086:i32)  [unwired: 2 in, 1 out]
                            n753 = Decimal String To Number(string=w1095) -> (number=w1089:i32)  [unwired: 2 in, 1 out]
                            n754 = Decimal String To Number(string=w1075) -> (number=w1084:i32)  [unwired: 2 in, 1 out]
                            n755 = Decimal String To Number(string=w1061) -> (number=w1067:i32)  [unwired: 2 in, 1 out]
                            n756 = Decimal String To Number(string=w1097) -> (number=w1087:i32)  [unwired: 2 in, 1 out]
                            n757 = Decimal String To Number(string=w1074) -> (number=w1083:i32)  [unwired: 2 in, 1 out]
                            n758 = Decimal String To Number(string=w1073) -> (number=w1082:i32)  [unwired: 2 in, 1 out]
                            n759 = Decimal String To Number(string=w1060) -> (number=w1058:i32)  [unwired: 2 in, 1 out]
                            n760 = Decimal String To Number(string=w1096) -> (number=w1088:i32)  [unwired: 2 in, 1 out]
                            n761 = Decimal String To Number(string=w1071) -> (number=w1070:i32)  [unwired: 2 in, 1 out]
                            n762 = Decimal String To Number(string=w1072) -> (number=w1081:i32)  [unwired: 2 in, 1 out]
                            n763 = Subtract(x=w1069, y=30) -> (x-y=w1147:i32)
                            n764 = Subtract(x=w1068, y=30) -> (x-y=w1146:i32)
                            n765 = Subtract(x=w1067, y=30) -> (x-y=w1145:i32)
                            n766 = Subtract(x=w1085, y=30) -> (x-y=w1153:i32)
                            n767 = Subtract(x=w1086, y=30) -> (x-y=w1154:i32)
                            n768 = Subtract(x=w1087, y=30) -> (x-y=w1155:i32)
                            n769 = Subtract(x=w1089, y=30) -> (x-y=w1157:i32)
                            n770 = Subtract(x=w1058, y=30) -> (x-y=w1144:i32)
                            n771 = Subtract(x=w1088, y=30) -> (x-y=w1156:i32)
                            n772 = Subtract(x=w1084, y=30) -> (x-y=w1148:i32)
                            n773 = Subtract(x=w1083, y=30) -> (x-y=w1149:i32)
                            n774 = Subtract(x=w1082, y=30) -> (x-y=w1150:i32)
                            n775 = Subtract(x=w1070, y=30) -> (x-y=w1152:i32)
                            n776 = Subtract(x=w1081, y=30) -> (x-y=w1151:i32)
                            n777 = Number To Decimal String(number=w1153) -> (decimal integer string=w1173:string)  [unwired: 1 in]
                            n778 = Number To Decimal String(number=w1154) -> (decimal integer string=w1172:string)  [unwired: 1 in]
                            n779 = Number To Decimal String(number=w1155) -> (decimal integer string=w1171:string)  [unwired: 1 in]
                            n780 = Number To Decimal String(number=w1156) -> (decimal integer string=w1170:string)  [unwired: 1 in]
                            n781 = Number To Decimal String(number=w1157) -> (decimal integer string=w1169:string)  [unwired: 1 in]
                            n782 = Number To Decimal String(number=w1148) -> (decimal integer string=w1163:string)  [unwired: 1 in]
                            n783 = Number To Decimal String(number=w1149) -> (decimal integer string=w1164:string)  [unwired: 1 in]
                            n784 = Number To Decimal String(number=w1150) -> (decimal integer string=w1165:string)  [unwired: 1 in]
                            n785 = Number To Decimal String(number=w1151) -> (decimal integer string=w1166:string)  [unwired: 1 in]
                            n786 = Number To Decimal String(number=w1152) -> (decimal integer string=w1167:string)  [unwired: 1 in]
                            n787 = Number To Decimal String(number=w1147) -> (decimal integer string=w1162:string)  [unwired: 1 in]
                            n788 = Number To Decimal String(number=w1146) -> (decimal integer string=w1161:string)  [unwired: 1 in]
                            n789 = Number To Decimal String(number=w1145) -> (decimal integer string=w1160:string)  [unwired: 1 in]
                            n790 = Number To Decimal String(number=w1144) -> (decimal integer string=w1159:string)  [unwired: 1 in]
                            n791 = Concatenate Strings(w1173, w1172, w1171, w1170, w1169) -> (w1128:string)
                            n792 = Concatenate Strings(w1163, w1164, w1165, w1166, w1167) -> (w1168:string)
                            n793 = Concatenate Strings(w1162, w1161, w1160, w1159) -> (w1158:string)
                            n794 = Decimal String To Number(string=w1168) -> (number=w1141:i32)  [unwired: 2 in, 1 out]
                            n795 = Decimal String To Number(string=w1158) -> (number=w1139:i32)  [unwired: 2 in, 1 out]
                            n796 = Decimal String To Number(string=w1128) -> (number=w1143:i32)  [unwired: 2 in, 1 out]
                            n797 = Divide(x=w1139, y=10.0) -> (x/y=w1135:dbl)
                            "Uwd(incerteza free)" <- w1135
                            n798 = Divide(x=w1141, y=10.0) -> (x/y=w1131:dbl)
                            "Altura Água-régua" <- w1131
                            n799 = Divide(x=w1143, y=10.0) -> (x/y=w1130:dbl)
                            "Altura Líquido-régua" <- w1130
                            n800 = local write "Altura Água erro"(w1135) -> ()
                            n801 = Subtract(x=w1130, y=18.0) -> (x-y=w1134:dbl)
                            n802 = Subtract(x=w1130, y=w1131) -> (x-y=→"Altura Kerosene-régua":dbl)
                            n803 = Subtract(x=w1131, y=18.0) -> (x-y=w1132:dbl)
                            n804 = local write "Altura Líquido"(w1134) -> ()
                            n805 = Subtract(x=w1134, y=w1132) -> (x-y=w1133:dbl)
                            n806 = local write "Altura Água"(w1132) -> ()
                            n807 = local write "Altura Kerosene"(w1133) -> ()
                            "MWU1100" <- i16 123 ("MWU1100")
                          }
                          frame #1 {
                            # "Lp"
                            # "Lp"
                            n808 = local read "Rho_W [Kg/m³]"() -> (w1301:dbl)
                            n809 = local read "Rho_Ar [kg/m³]"() -> (w1287:dbl)
                            n810 = local read "Rho_W [Kg/m³]"() -> (w1328:dbl)
                            n811 = local read "Rho_Ar [kg/m³]"() -> (w1286:dbl)
                            n812 = local read "Rho_W [Kg/m³]"() -> (w1321:dbl)
                            n813 = local read "Rho_W [Kg/m³]"() -> (w1314:dbl)
                            n814 = local read "SHD-PI-01-Ind."() -> (w1300:dbl)
                            n815 = local read "SHD-PI-01-Ind."() -> (w1299:dbl)
                            n816 = local read "Rho_K [Kg/m³]"() -> (w1304:dbl)
                            n817 = local read "Rho_K [Kg/m³]"() -> (w1320:dbl)
                            n818 = local read "Rho_K [Kg/m³]"() -> (w1315:dbl)
                            n819 = local read "Altura Líquido"() -> (w1303:dbl)
                            n820 = local read "Altura Líquido"() -> (w1305:dbl)
                            n821 = local read "Altura Líquido"() -> (w1327:dbl)
                            n822 = local read "Lm"() -> (w1302:dbl)
                            n823 = local read "Lm"() -> (w1306:dbl)
                            n824 = local read "Lm"() -> (w1326:dbl)
                            n825 = Multiply(x=1000.0, y=w1300) -> (x*y=w1308:dbl)
                            n826 = Multiply(x=w1301, y=w1302) -> (x*y=w1309:dbl)
                            n827 = Multiply(x=w1304, y=w1303) -> (x*y=w1311:dbl)
                            n828 = Add(x=w1305, y=w1306) -> (x+y=w1307:dbl)
                            n829 = Subtract(x=w1328, y=w1286) -> (x-y=w1325:dbl)
                            n830 = Add(x=w1327, y=w1326) -> (x+y=w1324:dbl)
                            n831 = Multiply(x=1000.0, y=w1299) -> (x*y=w1322:dbl)
                            n832 = Subtract(x=w1321, y=w1320) -> (x-y=w1318:dbl)
                            n833 = Subtract(x=w1314, y=w1315) -> (x-y=w1316:dbl)
                            n834 = Subtract(x=w1308, y=w1309) -> (x-y=w1310:dbl)
                            n835 = Multiply(x=w1307, y=w1287) -> (x*y=w1312:dbl)
                            n836 = Multiply(x=w1325, y=w1324) -> (x*y=w1323:dbl)
                            n837 = Subtract(x=w1310, y=w1311) -> (x-y=w1313:dbl)
                            n838 = Subtract(x=w1323, y=w1322) -> (x-y=w1319:dbl)
                            n839 = Add(x=w1313, y=w1312) -> (x+y=w1317:dbl)
                            n840 = Divide(x=w1317, y=w1316) -> (x/y=w1296:dbl)
                            n841 = Divide(x=w1319, y=w1318) -> (x/y=w1297:dbl)
                            n842 = local write "Lw"(w1296) -> ()
                            n843 = local write "Lk"(w1297) -> ()
                            n844 = Add(x=w1297, y=w1296) -> (x+y=w1298:dbl)
                            n845 = local write "Ll"(w1298) -> ()
                            n846 = local read "JW [m/s]"() -> (w1293:dbl)
                            n847 = local read "JK [m/s]"() -> (w1290:dbl)
                            n848 = Greater?(x=w1293, y=0.0) -> ()  [unwired: 1 out]
                            n849 = Greater?(x=w1290, y=0.0) -> ()  [unwired: 1 out]
                            n850 = case shown="True" FALSE {
                              frame False {
                              }
                              frame True {
                                # "Lp"
                                n851 = local read "Rho_Ar [kg/m³]"() -> (w1352:dbl)
                                n852 = local read "Rho_Ar [kg/m³]"() -> (w1345:dbl)
                                n853 = local read "Rho_W [Kg/m³]"() -> (w1347:dbl)
                                n854 = local read "Rho_Ar [kg/m³]"() -> (w1348:dbl)
                                n855 = local read "Rho_K [Kg/m³]"() -> (w1351:dbl)
                                n856 = local read "Rho_K [Kg/m³]"() -> (w1346:dbl)
                                n857 = local read "SHD-PI-01-Ind."() -> (w1349:dbl)
                                n858 = local read "Lm"() -> (w1342:dbl)
                                n859 = Subtract(x=w1347, y=w1348) -> (x-y=w1344:dbl)
                                n860 = Subtract(x=w1351, y=w1352) -> (x-y=w1353:dbl)
                                n861 = Subtract(x=w1346, y=w1345) -> (x-y=w1343:dbl)
                                n862 = Divide(x=1000.0, y=w1353) -> (x/y=w1350:dbl)
                                n863 = Divide(x=w1344, y=w1343) -> (x/y=w1341:dbl)
                                n864 = Multiply(x=w1350, y=w1349) -> (x*y=w1340:dbl)
                                n865 = Multiply(x=w1341, y=w1342) -> (x*y=w1339:dbl)
                                n866 = Subtract(x=w1340, y=w1339) -> (x-y=w1338:dbl)
                                n867 = local write "Lk"(w1338) -> ()
                              }
                            }
                            n868 = case shown="True" FALSE {
                              frame False {
                              }
                              frame True {
                                # "Lp"
                                n869 = local read "Rho_W [Kg/m³]"() -> (w1337:dbl)
                                n870 = local read "Rho_Ar [kg/m³]"() -> (w1336:dbl)
                                n871 = local read "SHD-PI-01-Ind."() -> (w1333:dbl)
                                n872 = local read "Lm"() -> (w1332:dbl)
                                n873 = Subtract(x=w1337, y=w1336) -> (x-y=w1335:dbl)
                                n874 = Subtract(x=w1333, y=w1332) -> (x-y=w1331:dbl)
                                n875 = Divide(x=1000.0, y=w1335) -> (x/y=w1330:dbl)
                                n876 = Multiply(x=w1331, y=w1330) -> (x*y=w1329:dbl)
                                n877 = local write "Lw"(w1329) -> ()
                              }
                            }
                          }
                          frame #2 {
                            # "RHOW"
                            # "LT(definir)"
                            # "RHOW"
                            n878 = local read "Valores"() -> (w1401:T4)
                            n879 = Unbundle By Name(w1401) -> ("Altura Total"=w1358:i32)
                            n880 = local read "Altura Água"() -> (w1410:dbl)
                            n881 = local read "Altura Líquido"() -> (w1409:dbl)
                            n882 = local read "Altura Líquido"() -> (w1408:dbl)
                            n883 = local read "Ll"() -> (w1359:dbl)
                            n884 = local read "Lw"() -> (w1362:dbl)
                            n885 = local read "Lk"() -> (w1369:dbl)
                            n886 = Divide(x=w1359, y=w1358) -> (x/y=w1360:dbl)
                            n887 = Divide(x=w1369, y=w1358) -> (x/y=w1368:dbl)
                            n888 = Divide(x=w1362, y=w1358) -> (x/y=w1364:dbl)
                            n889 = Divide(x=w1410, y=w1358) -> (x/y=→"HWSO":dbl)
                            n890 = Subtract(x=1.0, y=w1360) -> (x-y=w1356:dbl)
                            n891 = Subtract(x=w1408, y=w1409) -> (x-y=w1413:dbl)
                            n892 = Multiply(x=w1368, y=100.0) -> (x*y=w1366:dbl)
                            n893 = Multiply(x=w1364, y=100.0) -> (x*y=w1363:dbl)
                            n894 = Divide(x=w1413, y=w1358) -> (x/y=→"HKSO":dbl)
                            n895 = Multiply(x=w1356, y=100.0) -> (x*y=w1355:dbl)
                            n896 = local write "Hw"(w1363) -> ()
                            n897 = local write "Hk"(w1366) -> ()
                            n898 = local write "Vazio"(w1355) -> ()
                            n899 = local read "Altura Líquido"() -> (w1407:dbl)
                            n900 = local read "Valores"() -> (w1402:T4)
                            n901 = Unbundle By Name(w1402) -> ("Altura Total"=w1384:i32)
                            n902 = Divide(x=w1407, y=w1384) -> (x/y=w1374:dbl)
                            "H L" <- w1374
                            n903 = local read "Altura Líquido"() -> (w1406:dbl)
                            n904 = local read "Altura Água"() -> (w1385:dbl)
                            n905 = Subtract(x=1.0, y=w1374) -> (x-y=w1417:dbl)
                            n906 = local read "Altura Kerosene"() -> (w1405:dbl)
                            n907 = Subtract(x=1.0, y=w1374) -> (x-y=w1400:dbl)
                            n908 = Multiply(x=w1417, y=w1384) -> (x*y=→"L_a":dbl)
                            n909 = local read "Rho_Ar [kg/m³]"() -> (w1373:dbl)
                            n910 = Multiply(x=100.0, y=w1400) -> ()  [unwired: 1 out]
                            n911 = local read "Valores"() -> (w1404:T4)
                            n912 = local read "Rho_W [Kg/m³]"() -> (w1379:dbl)
                            n913 = Divide(x=w1406, y=w1384) -> (x/y=w1421:dbl)
                            n914 = Divide(x=w1405, y=w1384) -> (x/y=w1391:dbl)
                            n915 = Divide(x=w1385, y=w1384) -> (x/y=w1388:dbl)
                            n916 = Subtract(x=1.0, y=w1421) -> (x-y=w1394:dbl)
                            n917 = Multiply(x=100.0, y=w1391) -> (x*y=w1389:dbl)
                            n918 = Multiply(x=100.0, y=w1388) -> (x*y=w1386:dbl)
                            n919 = Unbundle By Name(w1404) -> ("Altura Total"=w1403:i32)
                            n920 = Multiply(x=100.0, y=w1394) -> (x*y=w1392:dbl)
                            n921 = local write "Hk Free"(w1389) -> ()
                            n922 = local write "Hw Free"(w1386) -> ()
                            n923 = local write "Vazio  Free"(w1392) -> ()
                            n924 = local read "Rho_K [Kg/m³]"() -> (w1377:dbl)
                            n925 = local read "Rho_W [Kg/m³]"() -> (w1378:dbl)
                            n926 = Divide(x=w1373, y=w1379) -> (x/y=w1430:dbl)
                            n927 = Subtract(x=1.0, y=w1374) -> (x-y=w1375:dbl)
                            n928 = Subtract(x=1.0, y=w1430) -> (x-y=w1429:dbl)
                            n929 = local read "PM"() -> (w1427:dbl)
                            n930 = Divide(x=w1377, y=w1378) -> (x/y=w1422:dbl)
                            n931 = Multiply(x=w1375, y=w1429) -> (x*y=w1428:dbl)
                            n932 = Divide(x=w1427, y=w1403) -> (x/y=w1426:dbl)
                            n933 = Subtract(x=w1428, y=w1426) -> (x-y=w1425:dbl)
                            n934 = Subtract(x=1.0, y=w1422) -> (x-y=w1423:dbl)
                            n935 = Divide(x=w1425, y=w1423) -> (x/y=w1398:dbl)
                            n936 = Multiply(x=w1398, y=w1384) -> (x*y=→"L_k":dbl)
                            n937 = Subtract(x=w1374, y=w1398) -> (x-y=w1395:dbl)
                            n938 = Multiply(x=w1395, y=w1384) -> (x*y=→"L_w":dbl)
                            n939 = Multiply(x=100.0, y=w1395) -> ()  [unwired: 1 out]
                            n940 = Multiply(x=100.0, y=w1398) -> ()  [unwired: 1 out]
                            n941 = case shown="False" FALSE {
                              tunnel: [w1437 w1439] -> w1383
                              tunnel: [w1436 w1438] -> w1371
                              frame False {
                                n942 = local read "Pressão02-CLP[0-4095]"() -> (w1434:dbl)
                                n943 = local read "Pressão01_CLP[0-4095]"() -> (w1435:dbl)
                                n944 = local read "Valores"() -> (w1432:T4)
                                n945 = call "Calculo_Pressao.vi"("X2"=w1434, "Valores"=w1432, "Calibrador"=TRUE, "X"=w1435) -> ("Pressao 2"=w1436:dbl, "Pressao"=w1437:dbl)  [unwired: 2 in]
                              }
                              frame True {
                                n946 = call "TESTE_PRESSAO_OFICINA.vi"() -> ("Pressão 2"=w1438:dbl, "Pressão 1"=w1439:dbl)  [unwired: 10 in]
                              }
                            }
                            n947 = local read "P_Bar [KPa]"() -> (w1372:dbl)
                            n948 = Add(x=w1371, y=w1372) -> (x+y=w1370:dbl)
                            n949 = Build Array(w1383, w1370) -> (w1382:dbl[])
                            n950 = local write "SHD-PI-01-Ind."(w1383) -> ()
                            n951 = local write "SHD-PI-01"(w1383) -> ()
                            n952 = Build Array(w1382) -> (w1381:dbl[][])
                            n953 = local write "Gráfico"(w1381) -> ()
                            n954 = local write "SHD-PI-02-Ind."(w1370) -> ()
                            n955 = local write "SHD-PI-02"(w1370) -> ()
                          }
                          frame #3 {
                            # "ALFA"
                            # "Ult"
                            # "Ull"
                            # "ult"
                            # "uLpk"
                            # "uLL"
                            # "uLp2"
                            # "pw"
                            # "uLpk"
                            # "uLL"
                            # "uLp1"
                            # "pw"
                            n956 = local read "Rho_W [Kg/m³]"() -> (w1457:dbl)
                            n957 = local read "Rho_W [Kg/m³]"() -> (w1456:dbl)
                            n958 = local read "Rho_W [Kg/m³]"() -> (w1449:dbl)
                            n959 = local read "Rho_K [Kg/m³]"() -> (w1441:dbl)
                            n960 = local read "Rho_W [Kg/m³]"() -> (w1450:dbl)
                            n961 = local read "SHD-PI-02-Ind."() -> (w1513:dbl)
                            n962 = local read "Altura Líquido"() -> (w1512:dbl)
                            n963 = local read "Rho_K [Kg/m³]"() -> (w1440:dbl)
                            n964 = local read "Rho_W [Kg/m³]"() -> (w1451:dbl)
                            n965 = local read "Rho_K [Kg/m³]"() -> (w1448:dbl)
                            n966 = local read "Rho_K [Kg/m³]"() -> (w1442:dbl)
                            n967 = local read "Rho_K [Kg/m³]"() -> (w1447:dbl)
                            n968 = local read "SHD-PI-01-Ind."() -> (w1511:dbl)
                            n969 = local read "Altura Líquido"() -> (w1510:dbl)
                            n970 = local read "Rho_W [Kg/m³]"() -> (w1453:dbl)
                            n971 = local read "Rho_K [Kg/m³]"() -> (w1444:dbl)
                            n972 = local read "Rho_W [Kg/m³]"() -> (w1452:dbl)
                            n973 = local read "Rho_K [Kg/m³]"() -> (w1443:dbl)
                            n974 = local read "SHD-PI-02-Ind."() -> (w1582:dbl)
                            n975 = local read "Altura Líquido"() -> (w1585:dbl)
                            n976 = Subtract(x=w1513, y=w1512) -> (x-y=w1550:dbl)
                            n977 = Subtract(x=w1451, y=w1442) -> (x-y=w1538:dbl)
                            n978 = Subtract(x=w1449, y=w1440) -> (x-y=w1553:dbl)
                            n979 = Subtract(x=w1450, y=w1441) -> (x-y=w1548:dbl)
                            n980 = Subtract(x=w1457, y=w1448) -> (x-y=w1581:dbl)
                            n981 = Divide(x=w1451, y=w1538) -> (x/y=w1539:dbl)
                            n982 = Subtract(x=w1511, y=w1510) -> (x-y=w1569:dbl)
                            n983 = Subtract(x=w1457, y=w1448) -> (x-y=w1571:dbl)
                            n984 = Multiply(x=w1550, y=w1449) -> (x*y=w1551:dbl)
                            n985 = Subtract(x=w1456, y=w1447) -> (x-y=w1566:dbl)
                            n986 = Square(x=w1553) -> (x^2=w1554:dbl)
                            n987 = Divide(x=w1450, y=w1548) -> (x/y=w1547:dbl)
                            n988 = Divide(x=w1457, y=w1581) -> (x/y=w1580:dbl)
                            n989 = Square(x=w1539) -> (x^2=w1542:dbl)
                            n990 = Multiply(x=w1569, y=w1456) -> (x*y=w1568:dbl)
                            n991 = Square(x=10.0) -> (x^2=w1541:dbl)
                            n992 = Divide(x=w1443, y=w1452) -> (x/y=w1588:dbl)
                            n993 = Divide(x=w1457, y=w1571) -> (x/y=w1572:dbl)
                            n994 = Square(x=w1566) -> (x^2=w1565:dbl)
                            n995 = Square(x=w1547) -> (x^2=w1544:dbl)
                            n996 = Divide(x=w1444, y=w1453) -> (x/y=w1584:dbl)
                            n997 = Square(x=w1580) -> (x^2=w1577:dbl)
                            n998 = Divide(x=w1551, y=w1554) -> (x/y=w1555:dbl)
                            n999 = Square(x=1.0) -> (x^2=w1545:dbl)
                            n1000 = Square(x=10.0) -> (x^2=w1578:dbl)
                            n1001 = Square(x=w1572) -> (x^2=w1575:dbl)
                            n1002 = Divide(x=w1568, y=w1565) -> (x/y=w1564:dbl)
                            n1003 = Square(x=1.0) -> (x^2=w1574:dbl)
                            n1004 = Multiply(x=w1542, y=w1541) -> (x*y=w1543:dbl)
                            n1005 = Square(x=w1555) -> (x^2=w1557:dbl)
                            n1006 = Multiply(x=w1544, y=w1545) -> (x*y=w1549:dbl)
                            n1007 = Multiply(x=w1584, y=w1585) -> (x*y=w1586:dbl)
                            n1008 = Subtract(x=1.0, y=w1588) -> (x-y=w1589:dbl)
                            n1009 = Square(x=5.0) -> (x^2=w1556:dbl)
                            n1010 = Multiply(x=w1577, y=w1578) -> (x*y=w1576:dbl)
                            n1011 = Square(x=w1564) -> (x^2=w1562:dbl)
                            n1012 = Multiply(x=w1575, y=w1574) -> (x*y=w1570:dbl)
                            n1013 = Subtract(x=w1582, y=w1586) -> (x-y=w1583:dbl)
                            n1014 = Square(x=5.0) -> (x^2=w1563:dbl)
                            n1015 = Multiply(x=w1557, y=w1556) -> (x*y=w1558:dbl)
                            n1016 = Add(x=w1543, y=w1549) -> (x+y=w1559:dbl)
                            n1017 = Multiply(x=w1562, y=w1563) -> (x*y=w1561:dbl)
                            n1018 = Add(x=w1576, y=w1570) -> (x+y=w1560:dbl)
                            n1019 = Divide(x=w1583, y=w1589) -> (x/y=w1525:dbl)
                            "Lwp2" <- w1525
                            n1020 = Add(x=w1559, y=w1558) -> (x+y=w1532:dbl)
                            "(Uwp2)²" <- w1532
                            n1021 = Add(x=w1560, y=w1561) -> (x+y=w1537:dbl)
                            "(Uwp1)²" <- w1537
                            n1022 = Divide(x=1.0, y=w1532) -> (x/y=w1526:dbl)
                            n1023 = Divide(x=1.0, y=w1537) -> (x/y=w1529:dbl)
                            n1024 = Multiply(x=w1525, y=w1526) -> (x*y=w1524:dbl)
                            n1025 = local read "Rho_W [Kg/m³]"() -> (w1454:dbl)
                            n1026 = local read "Rho_K [Kg/m³]"() -> (w1445:dbl)
                            n1027 = local read "Uwd(incerteza free)"() -> (w1485:dbl)
                            n1028 = local read "Rho_W [Kg/m³]"() -> (w1455:dbl)
                            n1029 = local read "Rho_K [Kg/m³]"() -> (w1446:dbl)
                            n1030 = local read "SHD-PI-01-Ind."() -> (w1597:dbl)
                            n1031 = local read "Altura Líquido"() -> (w1595:dbl)
                            n1032 = Divide(x=w1445, y=w1454) -> (x/y=w1591:dbl)
                            n1033 = Divide(x=w1446, y=w1455) -> (x/y=w1596:dbl)
                            n1034 = Multiply(x=w1596, y=w1595) -> (x*y=w1594:dbl)
                            n1035 = Subtract(x=1.0, y=w1591) -> (x-y=w1590:dbl)
                            n1036 = Square(x=w1485) -> (x^2=w1534:dbl)
                            n1037 = Subtract(x=w1597, y=w1594) -> (x-y=w1593:dbl)
                            n1038 = local read "Altura Água"() -> (w1527:dbl)
                            n1039 = Divide(x=1.0, y=w1534) -> (x/y=w1484:dbl)
                            n1040 = Divide(x=w1593, y=w1590) -> (x/y=w1528:dbl)
                            "Lwp1" <- w1528
                            n1041 = Multiply(x=w1527, y=w1484) -> (x*y=w1523:dbl)
                            n1042 = local read "Valores"() -> (w1499:T4)
                            n1043 = Compound Arithmetic op=ADD(w1529, w1484, w1526) -> (w1530:dbl)
                            "Calculo de gama" <- w1530
                            n1044 = local read "Altura Líquido"() -> (w1492:dbl)
                            n1045 = Unbundle By Name(w1499) -> ("Altura Total"=w1458:i32)
                            n1046 = Multiply(x=w1528, y=w1529) -> (x*y=w1522:dbl)
                            n1047 = Divide(x=1.0, y=w1530) -> (x/y=w1520:dbl)
                            n1048 = Square(x=w1458) -> (x^2=w1459:i32)
                            n1049 = Compound Arithmetic op=ADD(w1522, w1523, w1524) -> (w1521:dbl)
                            n1050 = Square Root(x=w1520) -> (sqrt(x)=w1461:dbl)
                            "ULw" <- w1461
                            n1051 = Multiply(x=w1521, y=w1520) -> (x*y=w1460:dbl)
                            "Lw(valor mais provavel)" <- w1460
                            n1052 = Divide(x=w1492, y=w1459) -> (x/y=w1491:dbl)
                            n1053 = Divide(x=1.0, y=w1458) -> (x/y=w1497:dbl)
                            n1054 = local read "Altura Água"() -> (w1505:dbl)
                            n1055 = Square(x=1.0 ("y")) -> (x^2=w1494:dbl)
                            n1056 = Square(x=w1491) -> (x^2=w1490:dbl)
                            n1057 = Square(x=1.0 ("y")) -> (x^2=w1489:dbl)
                            n1058 = Square(x=w1497) -> (x^2=w1496:dbl)
                            n1059 = Multiply(x=w1496, y=w1494) -> (x*y=w1493:dbl)
                            n1060 = Multiply(x=w1490, y=w1489) -> (x*y=w1487:dbl)
                            n1061 = local read "Altura Liquido erro"() -> (w1482:dbl)
                            n1062 = local read "Altura Água erro"() -> (w1481:dbl)
                            n1063 = Divide(x=w1505, y=w1459) -> (x/y=w1504:dbl)
                            n1064 = local read "Valores"() -> (w1519:T4)
                            n1065 = local read "Altura Líquido"() -> (w1518:dbl)
                            n1066 = Divide(x=1.0, y=w1458) -> (x/y=w1508:dbl)
                            n1067 = Square(x=w1504) -> (x^2=w1503:dbl)
                            n1068 = Square(x=1.0) -> (x^2=w1502:dbl)
                            n1069 = Square(x=w1461) -> (x^2=w1486:dbl)
                            n1070 = Unbundle By Name(w1519) -> ("Altura Total"=w1516:i32)
                            n1071 = local read "H L"() -> (w1515:dbl)
                            n1072 = Divide(x=w1460, y=w1458) -> (x/y=w1470:dbl)
                            n1073 = Square(x=w1508) -> (x^2=w1507:dbl)
                            n1074 = Multiply(x=w1503, y=w1502) -> (x*y=w1501:dbl)
                            n1075 = Subtract(x=w1515, y=w1470) -> (x-y=w1472:dbl)
                            n1076 = Multiply(x=w1507, y=w1486) -> (x*y=w1506:dbl)
                            n1077 = Multiply(x=w1470, y=100.0) -> (x*y=w1468:dbl)
                            n1078 = Square(x=w1482) -> (x^2=w1480:dbl)
                            n1079 = Square(x=w1481) -> (x^2=w1479:dbl)
                            n1080 = Multiply(x=w1472, y=100.0) -> (x*y=w1471:dbl)
                            n1081 = Add(x=w1506, y=w1501) -> (x+y=w1483:dbl)
                            n1082 = local write "Hw Mer"(w1468) -> ()
                            n1083 = Subtract(x=w1516, y=w1518) -> (x-y=w1517:dbl)
                            n1084 = Divide(x=w1517, y=w1516) -> (x/y=w1476:dbl)
                            n1085 = Add(x=w1480, y=w1479) -> (x+y=w1478:dbl)
                            n1086 = Square Root(x=w1483) -> (sqrt(x)=w1464:dbl)
                            "UHw" <- w1464
                            n1087 = local write "Hk Mer"(w1471) -> ()
                            n1088 = Compound Arithmetic op=ADD(w1493, w1487, w1483) -> (w1500:dbl)
                            n1089 = Multiply(x=w1476, y=100.0) -> (x*y=w1474:dbl)
                            n1090 = Square Root(x=w1478) -> (sqrt(x)=w1477:dbl)
                            n1091 = Multiply(x=100.0, y=w1464) -> (x*y=w1463:dbl)
                            n1092 = Square Root(x=w1500) -> (sqrt(x)=w1466:dbl)
                            "UHk" <- w1466
                            n1093 = local write "Altura Kerosene erro"(w1477) -> ()
                            n1094 = local write "Vazio Mer"(w1474) -> ()
                            n1095 = Multiply(x=100.0, y=w1466) -> (x*y=w1462:dbl)
                            n1096 = local write "Hw Mer erro"(w1463) -> ()
                            n1097 = local write "Hk Mer erro"(w1462) -> ()
                          }
                          frame #4 {
                            # "Upk"
                            # "UHL"
                            # "ULT"
                            # "ULL"
                            # "Uhk"
                            # "ULpm"
                            # "incerteza misto"
                            # "Ult"
                            # "Ult"
                            # "incerteza freescale"
                            # "Ult"
                            # "ULL"
                            n1098 = local read "Rho_W [Kg/m³]"() -> (w1602:dbl)
                            n1099 = local read "Rho_K [Kg/m³]"() -> (w1599:dbl)
                            n1100 = local read "Valores"() -> (w1695:T4)
                            n1101 = Unbundle By Name(w1695) -> ("Altura Total"=w1612:i32)
                            n1102 = local read "Altura Líquido"() -> (w1646:dbl)
                            n1103 = local read "Rho_W [Kg/m³]"() -> (w1600:dbl)
                            n1104 = local read "Rho_K [Kg/m³]"() -> (w1598:dbl)
                            n1105 = Square Root(x=2.0) -> (sqrt(x)=w1659:dbl)
                            n1106 = Subtract(x=w1602, y=w1599) -> (x-y=w1617:dbl)
                            n1107 = Divide(x=10.0, y=w1659) -> (x/y=w1634:dbl)
                            n1108 = Compound Arithmetic op=MULTIPLY(w1612, w1617) -> (w1657:dbl)
                            n1109 = Divide(x=1.0, y=w1612) -> (x/y=w1651:dbl)
                            n1110 = local read "Rho_W [Kg/m³]"() -> (w1603:dbl)
                            n1111 = Square(x=w1612) -> (x^2=w1645:i32)
                            n1112 = local read "Altura Líquido"() -> (w1688:dbl)
                            n1113 = Square(x=w1651) -> (x^2=w1650:dbl)
                            n1114 = Square(x=1.0) -> (x^2=w1649:dbl)
                            n1115 = Divide(x=w1603, y=w1657) -> (x/y=w1656:dbl)
                            n1116 = local read "Rho_W [Kg/m³]"() -> (w1601:dbl)
                            n1117 = local read "PM"() -> (w1615:dbl)
                            n1118 = local read "Altura Líquido"() -> (w1616:dbl)
                            n1119 = Divide(x=w1646, y=w1645) -> (x/y=w1644:dbl)
                            n1120 = Square(x=w1634) -> (x^2=w1633:dbl)
                            n1121 = Square(x=w1656) -> (x^2=w1655:dbl)
                            n1122 = Multiply(x=w1650, y=w1649) -> (x*y=w1647:dbl)
                            n1123 = Square(x=1.0) -> (x^2=w1642:dbl)
                            n1124 = Square(x=w1644) -> (x^2=w1643:dbl)
                            n1125 = Multiply(x=w1655, y=w1633) -> (x*y=w1654:dbl)
                            n1126 = Square(x=w1612) -> (x^2=w1661:i32)
                            n1127 = Multiply(x=w1643, y=w1642) -> (x*y=w1640:dbl)
                            n1128 = Add(x=w1647, y=w1640) -> (x+y=w1639:dbl)
                            n1129 = Subtract(x=w1600, y=w1598) -> (x-y=w1611:dbl)
                            n1130 = Divide(x=w1688, y=w1661) -> (x/y=w1689:dbl)
                            n1131 = Divide(x=1.0, y=w1612) -> (x/y=w1694:dbl)
                            n1132 = Square(x=w1611) -> (x^2=w1610:dbl)
                            n1133 = Square Root(x=w1639) -> (sqrt(x)=w1638:dbl)
                            n1134 = Subtract(x=w1616, y=w1615) -> (x-y=w1614:dbl)
                            n1135 = Square(x=w1694) -> (x^2=w1693:dbl)
                            n1136 = Square(x=1.0 ("y")) -> (x^2=w1692:dbl)
                            n1137 = Square(x=w1689) -> (x^2=w1690:dbl)
                            n1138 = Square(x=1.0 ("y")) -> (x^2=w1691:dbl)
                            n1139 = Multiply(x=w1612, y=w1610) -> (x*y=w1609:dbl)
                            n1140 = Multiply(x=w1693, y=w1692) -> (x*y=w1662:dbl)
                            n1141 = Multiply(x=w1690, y=w1691) -> (x*y=w1687:dbl)
                            n1142 = local read "Altura Água"() -> (w1666:dbl)
                            n1143 = Multiply(x=w1601, y=w1614) -> (x*y=w1613:dbl)
                            n1144 = Divide(x=w1613, y=w1609) -> (x/y=w1608:dbl)
                            n1145 = Add(x=w1662, y=w1687) -> (x+y=w1686:dbl)
                            n1146 = Square Root(x=w1686) -> (sqrt(x)=w1630:dbl)
                            "Ua" <- w1630
                            n1147 = Square(x=w1608) -> (x^2=w1607:dbl)
                            n1148 = Square(x=5.0) -> (x^2=w1606:dbl)
                            n1149 = local read "Altura Água erro"() -> (w1677:dbl)
                            n1150 = Multiply(x=w1630, y=100.0) -> (x*y=w1631:dbl)
                            n1151 = Multiply(x=w1607, y=w1606) -> (x*y=w1604:dbl)
                            n1152 = Divide(x=1.0, y=w1612) -> (x/y=w1679:dbl)
                            n1153 = Divide(x=w1666, y=w1661) -> (x/y=w1682:dbl)
                            n1154 = Square(x=1.0) -> (x^2=w1680:dbl)
                            n1155 = Square(x=w1682) -> (x^2=w1681:dbl)
                            n1156 = Square(x=w1679) -> (x^2=w1678:dbl)
                            n1157 = local write "Vazio Mer erro"(w1631) -> ()
                            n1158 = local write "Vazio Free erro"(w1631) -> ()
                            n1159 = local write "Vazio Misto erro"(w1631) -> ()
                            n1160 = Square(x=w1677) -> (x^2=w1676:dbl)
                            n1161 = Multiply(x=w1681, y=w1680) -> (x*y=w1675:dbl)
                            n1162 = Multiply(x=w1678, y=w1676) -> (x*y=w1673:dbl)
                            n1163 = Add(x=w1675, y=w1673) -> (x+y=w1674:dbl)
                            n1164 = Square Root(x=w1674) -> (sqrt(x)=w1619:dbl)
                            n1165 = Compound Arithmetic op=ADD(w1654, w1604) -> (w1653:dbl)
                            n1166 = Multiply(x=100.0, y=w1619) -> (x*y=w1618:dbl)
                            n1167 = local write "Hw Free erro"(w1618) -> ()
                            n1168 = Square Root(x=w1653) -> (sqrt(x)=w1629:dbl)
                            n1169 = Square(x=w1638) -> (x^2=w1636:dbl)
                            n1170 = Square(x=w1629) -> (x^2=w1637:dbl)
                            n1171 = Multiply(x=100.0, y=w1629) -> (x*y=w1627:dbl)
                            n1172 = local write "Hk  Misto erro"(w1627) -> ()
                            n1173 = local read "Altura Kerosene"() -> (w1672:dbl)
                            n1174 = Add(x=w1637, y=w1636) -> (x+y=w1635:dbl)
                            n1175 = Square Root(x=w1635) -> (sqrt(x)=w1625:dbl)
                            n1176 = Multiply(x=100.0, y=w1625) -> (x*y=w1624:dbl)
                            n1177 = Divide(x=w1672, y=w1661) -> (x/y=w1671:dbl)
                            n1178 = Square(x=1.0) -> (x^2=w1670:dbl)
                            n1179 = Square(x=w1671) -> (x^2=w1669:dbl)
                            n1180 = local write "Hw Misto erro"(w1624) -> ()
                            n1181 = Multiply(x=w1669, y=w1670) -> (x*y=w1668:dbl)
                            n1182 = Compound Arithmetic op=ADD(w1662, w1668, w1673) -> (w1667:dbl)
                            n1183 = Square Root(x=w1667) -> (sqrt(x)=w1622:dbl)
                            n1184 = Multiply(x=100.0, y=w1622) -> (x*y=w1621:dbl)
                            n1185 = local write "Hk Free erro"(w1621) -> ()
                          }
                        }
                      }
                      frame #4 {
                        n1186 = while {
                          stop <- w1704 stop-if-true
                          w1703 = T5."Enabled" ("Disabled")
                          n1187 = case shown="False" FALSE {
                            tunnel: [w1715 w1717] -> w1702
                            tunnel: [w1714 w1716] -> w1697
                            frame False {
                              n1188 = local read "Pressão02-CLP[0-4095]"() -> (w1712:dbl)
                              n1189 = local read "Pressão01_CLP[0-4095]"() -> (w1713:dbl)
                              n1190 = local read "Valores"() -> (w1710:T4)
                              n1191 = call "Calculo_Pressao.vi"("X2"=w1712, "Valores"=w1710, "Calibrador"=TRUE, "X"=w1713) -> ("Pressao 2"=w1714:dbl, "Pressao"=w1715:dbl)  [unwired: 2 in]
                            }
                            frame True {
                              n1192 = call "TESTE_PRESSAO_OFICINA.vi"() -> ("Pressão 2"=w1716:dbl, "Pressão 1"=w1717:dbl)  [unwired: 10 in]
                            }
                          }
                          n1193 = local read "P_Bar [KPa]"() -> (w1698:dbl)
                          n1194 = Add(x=w1697, y=w1698) -> (x+y=w1696:dbl)
                          n1195 = Build Array(w1702, w1696) -> (w1701:dbl[])
                          n1196 = Build Array(w1701) -> (w1700:dbl[][])
                          n1197 = local write "Gráfico"(w1700) -> ()
                          n1198 = local write "SHD-PI-01-Ind."(w1702) -> ()
                          n1199 = local write "SHD-PI-01"(w1702) -> ()
                          n1200 = local write "SHD-PI-02-Ind."(w1696) -> ()
                          n1201 = local write "SHD-PI-02"(w1696) -> ()
                          n1202 = property on="Cluster 2" class="Clust (strict)"("DisabledEnum"=w1703) -> ()  [unwired: 2 in, 2 out]
                          n1203 = property on="Gravar teste" class="Bool (strict)"("DisabledEnum"=w1703) -> ()  [unwired: 2 in, 2 out]
                          n1204 = local read "Cluster"() -> (w1709:T3)
                          n1205 = local read "Gravar teste"() -> (w1705:bool)
                          n1206 = local read "stop VI"() -> (w1707:bool)
                          n1207 = Unbundle By Name(w1709) -> ("Home"=w1706:bool)
                          n1208 = Compound Arithmetic op=OR(w1707, w1706, w1705) -> (w1704:bool)
                          n1209 = property on="Home" class="Bool (strict)"("Visible"=TRUE) -> ()  [unwired: 2 in, 2 out]
                        }
                      }
                      frame #5 {
                        n1210 = case shown="True" "Gravar teste" {
                          frame False {
                          }
                          frame True {
                            n1211 = stacked-sequence {
                              frame #0 {
                                w1726 = T5."Disabled and Grayed Out" ("Disabled")
                                n1212 = case shown="False" FALSE {
                                tunnel: [w1735 w1737] -> w1723
                                tunnel: [w1734 w1736] -> w1720
                                frame False {
                                n1213 = local read "Pressão02-CLP[0-4095]"() -> (w1732:dbl)
                                n1214 = local read "Pressão01_CLP[0-4095]"() -> (w1733:dbl)
                                n1215 = local read "Valores"() -> (w1730:T4)
                                n1216 = call "Calculo_Pressao.vi"("X2"=w1732, "Valores"=w1730, "Calibrador"=TRUE, "X"=w1733) -> ("Pressao 2"=w1734:dbl, "Pressao"=w1735:dbl)  [unwired: 2 in]
                                }
                                frame True {
                                n1217 = call "TESTE_PRESSAO_OFICINA.vi"() -> ("Pressão 2"=w1736:dbl, "Pressão 1"=w1737:dbl)  [unwired: 10 in]
                                }
                                }
                                n1218 = local read "P_Bar [KPa]"() -> (w1721:dbl)
                                n1219 = local read "Cluster 2"() -> (w1728:T2)
                                n1220 = Add(x=w1720, y=w1721) -> (x+y=w1719:dbl)
                                n1221 = Build Array(w1723, w1719) -> (w1724:dbl[])
                                n1222 = property on="Cluster 2" class="Clust (strict)"("DisabledEnum"=w1726) -> ()  [unwired: 2 in, 2 out]
                                n1223 = local write "SIT-CV-AT"(FALSE ("SKT 3")) -> ()
                                n1224 = property on="Gravar teste" class="Bool (strict)"("DisabledEnum"=w1726) -> ()  [unwired: 2 in, 2 out]
                                n1225 = local write "SHD-PI-01-Ind."(w1723) -> ()
                                n1226 = local write "SHD-PI-01"(w1723) -> ()
                                n1227 = local write "SHD-PI-02-Ind."(w1719) -> ()
                                n1228 = local write "SHD-PI-02"(w1719) -> ()
                                n1229 = Build Array(w1724) -> (w1725:dbl[][])
                                n1230 = local write "Gráfico"(w1725) -> ()
                                n1231 = Unbundle By Name(w1728) -> ("Formato"=w1727:enum32{"Item 0", "Item 1"})
                                n1232 = case shown="\"Item 0\", Default" w1727 {
                                frame "Item 0", Default {
                                n1233 = local read "Vazio"() -> (w1778:dbl)
                                n1234 = local read "Vazio Misto erro"() -> (w1777:dbl)
                                n1235 = local read "Hw"() -> (w1776:dbl)
                                n1236 = local read "Hw Misto erro"() -> (w1775:dbl)
                                n1237 = local read "Hk"() -> (w1774:dbl)
                                n1238 = local read "Hk  Misto erro"() -> (w1773:dbl)
                                n1239 = local read "Vazio  Free"() -> (w1772:dbl)
                                n1240 = local read "Vazio Free erro"() -> (w1771:dbl)
                                n1241 = local read "Hw Free"() -> (w1770:dbl)
                                n1242 = local read "Hw Free erro"() -> (w1769:dbl)
                                n1243 = local read "Hk Free"() -> (w1768:dbl)
                                n1244 = local read "Hk Free erro"() -> (w1767:dbl)
                                n1245 = local read "Vazio Mer"() -> (w1766:dbl)
                                n1246 = local read "Vazio Mer erro"() -> (w1765:dbl)
                                n1247 = local read "Hw Mer"() -> (w1764:dbl)
                                n1248 = local read "Hw Mer erro"() -> (w1763:dbl)
                                n1249 = local read "Hk Mer"() -> (w1762:dbl)
                                n1250 = local read "Hk Mer erro"() -> (w1761:dbl)
                                n1251 = local read "Altura Líquido"() -> (w1748:dbl)
                                n1252 = local read "Altura Liquido erro"() -> (w1747:dbl)
                                n1253 = local read "JW [m/s]"() -> (w1755:dbl)
                                n1254 = local read "JK [m/s]"() -> (w1754:dbl)
                                n1255 = local read "JG [m/s]"() -> (w1753:dbl)
                                n1256 = local read "Altura Água"() -> (w1746:dbl)
                                n1257 = local read "Altura Água erro"() -> (w1745:dbl)
                                n1258 = local read "Altura Kerosene"() -> (w1744:dbl)
                                n1259 = local read "Altura Kerosene erro"() -> (w1743:dbl)
                                n1260 = local read "Lw"() -> (w1740:dbl)
                                n1261 = local read "Lk"() -> (w1741:dbl)
                                n1262 = local read "Ll"() -> (w1742:dbl)
                                n1263 = Build Array(w1755, w1754, w1753, w1778, w1777, w1776, w1775, w1774, w1773, w1772, w1771, w1770, w1769, w1768, w1767, w1766, w1765, w1764, w1763, w1762, w1761, w1748, w1747, w1746, w1745, w1744, w1743, w1742, w1741, w1740) -> (w1757:dbl[])
                                n1264 = local read "JG_Lam [m/s]"() -> (w1739:dbl)
                                n1265 = local read "Cluster 2"() -> (w1780:T2)
                                n1266 = local read "SHD-PI-02-AUX"() -> (w1738:dbl)
                                n1267 = local read "P_Bar [KPa]"() -> (w1752:dbl)
                                n1268 = local read "SHD-PI-01"() -> (w1779:dbl)
                                n1269 = local read "T_W [°C]"() -> (w1751:dbl)
                                n1270 = local read "T_Atm [°C]"() -> (w1749:dbl)
                                n1271 = local read "T_K [°C]"() -> (w1750:dbl)
                                n1272 = Unbundle By Name(w1780) -> ("File Path Control"=w1760:path)
                                n1273 = call "Nome_Arquivo.vi"("formato"="txt", "Numeric 3"=w1739, "Numeric 2"=w1754, "Numeric"=w1755, "Path"=w1760) -> ("path"=w1758:path)  [unwired: 5 in, 1 out]
                                n1274 = Build Array(w1779, w1738, w1752, w1751, w1750, w1749) -> (w1756:dbl[])
                                n1275 = call "Salvar_txt.vi"("path"=w1758, "Array"=w1757, "Array 3"=w1756) -> ()  [unwired: 3 in]
                                }
                                frame "Item 1" {
                                (unwired) FALSE
                                n1276 = local read "Vazio"() -> (w1821:dbl)
                                n1277 = local read "Vazio Misto erro"() -> (w1820:dbl)
                                n1278 = local read "Hw"() -> (w1819:dbl)
                                n1279 = local read "Hw Misto erro"() -> (w1818:dbl)
                                n1280 = local read "Hk"() -> (w1817:dbl)
                                n1281 = local read "Hk  Misto erro"() -> (w1816:dbl)
                                n1282 = local read "Vazio  Free"() -> (w1815:dbl)
                                n1283 = local read "Vazio Free erro"() -> (w1814:dbl)
                                n1284 = local read "Hw Free"() -> (w1813:dbl)
                                n1285 = local read "Hw Free erro"() -> (w1812:dbl)
                                n1286 = local read "Hk Free"() -> (w1811:dbl)
                                n1287 = local read "Hk Free erro"() -> (w1810:dbl)
                                n1288 = local read "Altura Líquido"() -> (w1803:dbl)
                                n1289 = local read "Altura Liquido erro"() -> (w1802:dbl)
                                n1290 = local read "Altura Água"() -> (w1801:dbl)
                                n1291 = local read "Altura Água erro"() -> (w1800:dbl)
                                n1292 = local read "Altura Kerosene"() -> (w1799:dbl)
                                n1293 = local read "Altura Kerosene erro"() -> (w1798:dbl)
                                n1294 = local read "Vazio Mer"() -> (w1809:dbl)
                                n1295 = local read "Vazio Mer erro"() -> (w1808:dbl)
                                n1296 = local read "Hw Mer"() -> (w1807:dbl)
                                n1297 = local read "Hw Mer erro"() -> (w1806:dbl)
                                n1298 = local read "Hk Mer"() -> (w1805:dbl)
                                n1299 = local read "Hk Mer erro"() -> (w1804:dbl)
                                n1300 = local read "JW [m/s]"() -> (w1793:dbl)
                                n1301 = local read "JK [m/s]"() -> (w1792:dbl)
                                n1302 = local read "JG [m/s]"() -> (w1791:dbl)
                                n1303 = local read "SHD-PI-02-AUX"() -> (w1786:dbl)
                                n1304 = local read "SHD-PI-01"() -> (w1787:dbl)
                                n1305 = local read "P_Bar [KPa]"() -> (w1785:dbl)
                                n1306 = local read "T_W [°C]"() -> (w1784:dbl)
                                n1307 = local read "T_Atm [°C]"() -> (w1782:dbl)
                                n1308 = local read "T_K [°C]"() -> (w1783:dbl)
                                n1309 = local read "Lw"() -> (w1789:dbl)
                                n1310 = local read "Lk"() -> (w1788:dbl)
                                n1311 = local read "Ll"() -> (w1790:dbl)
                                n1312 = local read "JG_Lam [m/s]"() -> (w1781:dbl)
                                n1313 = Build Array(w1793, w1792, w1791, w1821, w1820, w1819, w1818, w1817, w1816, w1815, w1814, w1813, w1812, w1811, w1810, w1809, w1808, w1807, w1806, w1805, w1804, w1803, w1802, w1801, w1800, w1799, w1798, w1790, w1789, w1788, w1787, w1786, w1785, w1784, w1783, w1782) -> (w1794:dbl[])
                                n1314 = local read "Cluster 2"() -> (w1822:T2)
                                n1315 = Unbundle By Name(w1822) -> ("File Path Control"=w1797:path)
                                n1316 = call "Nome_Arquivo.vi"("formato"="xlsx" ("input 10"), "Numeric 3"=w1781, "Numeric 2"=w1792, "Numeric"=w1793, "Path"=w1797) -> ("path"=w1795:path)  [unwired: 5 in, 1 out]
                                n1317 = call "Salvar_excel.vi"("Array"=w1794, "Filename"=w1795) -> ()  [unwired: 10 in]
                                }
                                }
                              }
                              frame #1 {
                                w1823 = T5."Enabled" ("Disabled")
                                n1318 = local write "Gravar teste"(FALSE ("Gravar teste")) -> ()
                                n1319 = property on="Cluster 2" class="Clust (strict)"("DisabledEnum"=w1823) -> ()  [unwired: 2 in, 2 out]
                                n1320 = property on="Gravar teste" class="Bool (strict)"("DisabledEnum"=w1823) -> ()  [unwired: 2 in, 2 out]
                              }
                            }
                          }
                        }
                      }
                      frame #6 {
                        n1321 = flat-sequence {
                          frame #0 {
                            n1322 = local write "MWU1100"(i16 200 ("MWU1100")) -> ()
                            n1323 = One Button Dialog(message="O sensor foi enviado para HOME, aguarde ele retornar", button name ("OK")="OK") -> ()  [unwired: 1 out]
                          }
                          frame #1 {
                            n1324 = Wait (ms)(milliseconds to wait=u32 250) -> ()  [unwired: 1 out]
                          }
                        }
                      }
                      frame #7 {
                        n1325 = local read "Cluster"() -> (w1830:T3)
                        n1326 = Unbundle By Name(w1830) -> ("Progresso Sensor"=w1829:dbl)
                        n1327 = while {
                          tunnel: w1831 -> [w1838]
                          shift-right: [w1835] -> _
                          shift-left: w1829 -> [w1836]
                          stop <- w1843 stop-if-true
                          n1328 = local read "Gravar teste"() -> (w1854:bool)
                          n1329 = invoke class="VI" method="Ctrl Val.Get"(reference=w1838, "Control Name"="STRING") -> ("Get Control Value Variant"=w1841:variant)  [unwired: 2 in, 3 out]
                          n1330 = case shown="True" w1854 {
                            frame False {
                            }
                            frame True {
                              n1331 = stacked-sequence {
                                frame #0 {
                                w1922 = T5."Disabled and Grayed Out" ("Disabled")
                                n1332 = local read "Cluster 2"() -> (w1924:T2)
                                n1333 = local write "SIT-CV-AT"(FALSE ("SKT 3")) -> ()
                                n1334 = property on="Cluster 2" class="Clust (strict)"("DisabledEnum"=w1922) -> ()  [unwired: 2 in, 2 out]
                                n1335 = property on="Gravar teste" class="Bool (strict)"("DisabledEnum"=w1922) -> ()  [unwired: 2 in, 2 out]
                                n1336 = Unbundle By Name(w1924) -> ("Formato"=w1923:enum32{"Item 0", "Item 1"})
                                n1337 = case shown="\"Item 1\"" w1923 {
                                frame "Item 0", Default {
                                n1338 = local read "Vazio"() -> (w1952:dbl)
                                n1339 = local read "Vazio Misto erro"() -> (w1951:dbl)
                                n1340 = local read "Hw"() -> (w1950:dbl)
                                n1341 = local read "Hw Misto erro"() -> (w1949:dbl)
                                n1342 = local read "Hk"() -> (w1948:dbl)
                                n1343 = local read "Hk  Misto erro"() -> (w1947:dbl)
                                n1344 = local read "Vazio  Free"() -> (w1946:dbl)
                                n1345 = local read "Vazio Free erro"() -> (w1945:dbl)
                                n1346 = local read "Hw Free"() -> (w1944:dbl)
                                n1347 = local read "Hw Free erro"() -> (w1943:dbl)
                                n1348 = local read "Hk Free"() -> (w1942:dbl)
                                n1349 = local read "Hk Free erro"() -> (w1941:dbl)
                                n1350 = local read "Vazio Mer"() -> (w1940:dbl)
                                n1351 = local read "Vazio Mer erro"() -> (w1939:dbl)
                                n1352 = local read "Hw Mer"() -> (w1938:dbl)
                                n1353 = local read "Hw Mer erro"() -> (w1937:dbl)
                                n1354 = local read "Hk Mer"() -> (w1936:dbl)
                                n1355 = local read "Hk Mer erro"() -> (w1935:dbl)
                                n1356 = local read "JW [m/s]"() -> (w1928:dbl)
                                n1357 = local read "JK [m/s]"() -> (w1927:dbl)
                                n1358 = local read "JG [m/s]"() -> (w1926:dbl)
                                n1359 = Build Array(w1928, w1927, w1926, w1952, w1951, w1950, w1949, w1948, w1947, w1946, w1945, w1944, w1943, w1942, w1941, w1940, w1939, w1938, w1937, w1936, w1935) -> (w1930:dbl[])
                                n1360 = local read "Altura Líquido"() -> (w1958:dbl)
                                n1361 = local read "Altura Liquido erro"() -> (w1957:dbl)
                                n1362 = local read "Altura Água"() -> (w1956:dbl)
                                n1363 = local read "Altura Água erro"() -> (w1955:dbl)
                                n1364 = local read "Altura Kerosene"() -> (w1954:dbl)
                                n1365 = local read "Altura Kerosene erro"() -> (w1953:dbl)
                                n1366 = Build Array(w1958, w1957, w1956, w1955, w1954, w1953) -> (w1931:dbl[])
                                n1367 = local read "Cluster 2"() -> (w1961:T2)
                                n1368 = local read "SHD-PI-02-AUX"() -> (w1960:dbl)
                                n1369 = Unbundle By Name(w1961) -> ("File Path Control"=w1934:path)
                                n1370 = local read "SHD-PI-01"() -> (w1959:dbl)
                                n1371 = call "Nome_Arquivo.vi"("formato"="txt" ("input 10"), "Numeric 3"=w1926, "Numeric 2"=w1927, "Numeric"=w1928, "Path"=w1934) -> ("path"=w1929:path)  [unwired: 5 in, 1 out]
                                n1372 = Build Array(w1959, w1960) -> (w1932:dbl[])
                                n1373 = call "Salvar_txt.vi"("path"=w1929, "Array"=w1930, "Array 2"=w1931, "Array 3"=w1932) -> ()  [unwired: 2 in]
                                }
                                frame "Item 1" {
                                n1374 = local read "SHD-PI-02-AUX"() -> (w1965:dbl)
                                n1375 = local read "JW [m/s]"() -> (w1964:dbl)
                                n1376 = local read "JK [m/s]"() -> (w1963:dbl)
                                n1377 = local read "JG [m/s]"() -> (w1962:dbl)
                                n1378 = local read "Vazio"() -> (w1994:dbl)
                                n1379 = local read "Vazio Misto erro"() -> (w1993:dbl)
                                n1380 = local read "Hw"() -> (w1992:dbl)
                                n1381 = local read "Hw Misto erro"() -> (w1991:dbl)
                                n1382 = local read "Hk"() -> (w1990:dbl)
                                n1383 = local read "Hk  Misto erro"() -> (w1989:dbl)
                                n1384 = local read "Vazio  Free"() -> (w1988:dbl)
                                n1385 = local read "Vazio Free erro"() -> (w1987:dbl)
                                n1386 = local read "Hw Free"() -> (w1986:dbl)
                                n1387 = local read "Hw Free erro"() -> (w1985:dbl)
                                n1388 = local read "Hk Free"() -> (w1984:dbl)
                                n1389 = local read "Hk Free erro"() -> (w1983:dbl)
                                n1390 = local read "Vazio Mer"() -> (w1982:dbl)
                                n1391 = local read "Vazio Mer erro"() -> (w1981:dbl)
                                n1392 = local read "Hw Mer"() -> (w1980:dbl)
                                n1393 = local read "Hw Mer erro"() -> (w1979:dbl)
                                n1394 = local read "Hk Mer"() -> (w1978:dbl)
                                n1395 = local read "Hk Mer erro"() -> (w1977:dbl)
                                n1396 = local read "Altura Líquido"() -> (w1976:dbl)
                                n1397 = local read "Altura Liquido erro"() -> (w1975:dbl)
                                n1398 = local read "Altura Água"() -> (w1974:dbl)
                                n1399 = local read "Altura Água erro"() -> (w1973:dbl)
                                n1400 = local read "Altura Kerosene"() -> (w1972:dbl)
                                n1401 = local read "Altura Kerosene erro"() -> (w1971:dbl)
                                n1402 = local read "SHD-PI-01"() -> (w1970:dbl)
                                n1403 = Build Array(w1964, w1963, w1962, w1994, w1993, w1992, w1991, w1990, w1989, w1988, w1987, w1986, w1985, w1984, w1983, w1982, w1981, w1980, w1979, w1978, w1977, w1976, w1975, w1974, w1973, w1972, w1971, w1970, w1965) -> (w1967:dbl[])
                                n1404 = local read "Cluster 2"() -> (w1995:T2)
                                n1405 = Unbundle By Name(w1995) -> ("File Path Control"=w1968:path)
                                n1406 = call "Nome_Arquivo.vi"("formato"="xlsx" ("input 10"), "Numeric 3"=w1962, "Numeric 2"=w1963, "Numeric"=w1964, "Path"=w1968) -> ("path"=w1966:path)  [unwired: 5 in, 1 out]
                                n1407 = call "Salvar_excel.vi"("Array"=w1967, "Filename"=w1966) -> ()  [unwired: 10 in]
                                }
                                }
                                }
                                frame #1 {
                                w1996 = T5."Enabled" ("Disabled")
                                n1408 = local write "Gravar teste"(FALSE ("Gravar teste")) -> ()
                                n1409 = property on="Cluster 2" class="Clust (strict)"("DisabledEnum"=w1996) -> ()  [unwired: 2 in, 2 out]
                                n1410 = property on="Gravar teste" class="Bool (strict)"("DisabledEnum"=w1996) -> ()  [unwired: 2 in, 2 out]
                                }
                              }
                            }
                          }
                          n1411 = local read "STRING"() -> (w1840:string)
                          n1412 = Variant To Data(type=w1840, Variant=w1841) -> (data=w1837:string)  [unwired: 1 in, 1 out]
                          n1413 = local write "STRING"(w1837) -> ()
                          n1414 = case shown="True" FALSE {
                            tunnel: [w1856 w1857] -> w1849
                            tunnel: w1837 -> [w1856 _]
                            frame False {
                            }
                            frame True {
                              n1415 = local read "MWU2975"() -> (w1873:i16)
                              n1416 = local read "MWU2976"() -> (w1872:i16)
                              n1417 = local read "MWU2977"() -> (w1871:i16)
                              n1418 = local read "MWU2978"() -> (w1870:i16)
                              n1419 = local read "MWU2979"() -> (w1869:i16)
                              n1420 = local read "MWU2980"() -> (w1868:i16)
                              n1421 = local read "MWU2981"() -> (w1867:i16)
                              n1422 = local read "MWU2982"() -> (w1866:i16)
                              n1423 = local read "MWU2983"() -> (w1865:i16)
                              n1424 = local read "MWU2984"() -> (w1864:i16)
                              n1425 = local read "MWU2985"() -> (w1863:i16)
                              n1426 = local read "MWU2986"() -> (w1862:i16)
                              n1427 = local read "MWU2987"() -> (w1861:i16)
                              n1428 = call "Conversor-bin-hex.vi"("Numeric"=w1873) -> ("hex integer string"=w1895:string)  [unwired: 9 in, 1 out]
                              n1429 = call "Conversor-bin-hex.vi"("Numeric"=w1872) -> ("hex integer string"=w1893:string, "hex integer string 2"=w1894:string)  [unwired: 9 in]
                              n1430 = call "Conversor-bin-hex.vi"("Numeric"=w1871) -> ("hex integer string"=w1891:string, "hex integer string 2"=w1892:string)  [unwired: 9 in]
                              n1431 = call "Conversor-bin-hex.vi"("Numeric"=w1870) -> ("hex integer string"=w1889:string, "hex integer string 2"=w1890:string)  [unwired: 9 in]
                              n1432 = call "Conversor-bin-hex.vi"("Numeric"=w1869) -> ("hex integer string"=w1887:string, "hex integer string 2"=w1888:string)  [unwired: 9 in]
                              n1433 = call "Conversor-bin-hex.vi"("Numeric"=w1868) -> ("hex integer string"=w1885:string, "hex integer string 2"=w1886:string)  [unwired: 9 in]
                              n1434 = call "Conversor-bin-hex.vi"("Numeric"=w1867) -> ("hex integer string"=w1883:string, "hex integer string 2"=w1884:string)  [unwired: 9 in]
                              n1435 = call "Conversor-bin-hex.vi"("Numeric"=w1866) -> ("hex integer string"=w1881:string, "hex integer string 2"=w1882:string)  [unwired: 9 in]
                              n1436 = call "Conversor-bin-hex.vi"("Numeric"=w1865) -> ("hex integer string"=w1879:string, "hex integer string 2"=w1880:string)  [unwired: 9 in]
                              n1437 = call "Conversor-bin-hex.vi"("Numeric"=w1864) -> ("hex integer string"=w1877:string, "hex integer string 2"=w1878:string)  [unwired: 9 in]
                              n1438 = call "Conversor-bin-hex.vi"("Numeric"=w1863) -> ("hex integer string"=w1875:string, "hex integer string 2"=w1876:string)  [unwired: 9 in]
                              n1439 = call "Conversor-bin-hex.vi"("Numeric"=w1862) -> ("hex integer string"=w1860:string, "hex integer string 2"=w1874:string)  [unwired: 9 in]
                              n1440 = call "Conversor-bin-hex.vi"("Numeric"=w1861) -> ("hex integer string"=w1858:string, "hex integer string 2"=w1859:string)  [unwired: 9 in]
                              n1441 = Concatenate Strings(w1895, w1894, w1893, w1892, w1891, w1890, w1889, w1888, w1887, w1886, w1885, w1884, w1883, w1882, w1881, w1880, w1879, w1878, w1877, w1876, w1875, w1874, w1860, w1859, w1858) -> (w1896:string)
                              n1442 = call "string_inteira_carater.vi"("String in"=w1896) -> ("String out"=w1857:string)  [unwired: 10 in]
                            }
                          }
                          n1443 = String Subset(string=w1849, offset (0)=3, length (rest)=1 ("length (rest)")) -> (substring=w1846:string)
                          n1444 = local write "String Caracter de Comunicação"(w1849) -> ()
                          n1445 = Equal?(x=w1846, y="H") -> (x = y?=w1844:bool)
                          n1446 = case shown="True" w1844 {
                            tunnel: [FALSE TRUE] -> w1843
                            tunnel: w1836 -> [w1898 _]
                            tunnel: [w1897 0.0] -> w1835
                            frame False {
                              n1447 = flat-sequence {
                                tunnel: w1898 -> [w1905]
                                tunnel: [w1904] -> w1897
                                frame #0 {
                                n1448 = local write "MWU1100"(i16 123 ("MWU1100")) -> ()
                                }
                                frame #1 {
                                n1449 = Wait (ms)(milliseconds to wait=u32 500) -> ()  [unwired: 1 out]
                                }
                                frame #2 {
                                n1450 = local write "MWU1100"(i16 456 ("MWU1100")) -> ()
                                }
                                frame #3 {
                                n1451 = Wait (ms)(milliseconds to wait=u32 500) -> ()  [unwired: 1 out]
                                }
                                frame #4 {
                                n1452 = Subtract(x=w1905, y=1.0) -> (x-y=w1904:dbl)
                                n1453 = local read "Cluster"() -> (w1907:T3)
                                n1454 = Bundle By Name(cluster=w1907, "Progresso Sensor"=w1904) -> (w1908:T3)
                                n1455 = local write "Cluster"(w1908) -> ()
                                }
                              }
                            }
                            frame True {
                              n1456 = local read "Cluster"() -> (w1910:T3)
                              n1457 = Bundle By Name(cluster=w1910, "Progresso Sensor"=0.0) -> (w1911:T3)
                              n1458 = local write "Cluster"(w1911) -> ()
                            }
                          }
                          n1459 = property on="Home" class="Bool (strict)"("DisabledEnum"=T5."Disabled and Grayed Out" ("Disabled")) -> ()  [unwired: 2 in, 2 out]
                          n1460 = case shown="False" FALSE {
                            tunnel: [w1919 w1921] -> w1853
                            tunnel: [w1918 w1920] -> w1833
                            frame False {
                              n1461 = local read "Pressão02-CLP[0-4095]"() -> (w1916:dbl)
                              n1462 = local read "Pressão01_CLP[0-4095]"() -> (w1917:dbl)
                              n1463 = local read "Valores"() -> (w1914:T4)
                              n1464 = call "Calculo_Pressao.vi"("X2"=w1916, "Valores"=w1914, "Calibrador"=TRUE, "X"=w1917) -> ("Pressao 2"=w1918:dbl, "Pressao"=w1919:dbl)  [unwired: 2 in]
                            }
                            frame True {
                              n1465 = call "TESTE_PRESSAO_OFICINA.vi"() -> ("Pressão 2"=w1920:dbl, "Pressão 1"=w1921:dbl)  [unwired: 10 in]
                            }
                          }
                          n1466 = local read "P_Bar [KPa]"() -> (w1834:dbl)
                          n1467 = Add(x=w1833, y=w1834) -> (x+y=w1832:dbl)
                          n1468 = Build Array(w1853, w1832) -> (w1852:dbl[])
                          n1469 = local write "SHD-PI-01-Ind."(w1853) -> ()
                          n1470 = local write "SHD-PI-01"(w1853) -> ()
                          n1471 = local write "SHD-PI-02-Ind."(w1832) -> ()
                          n1472 = local write "SHD-PI-02"(w1832) -> ()
                          n1473 = Build Array(w1852) -> (w1851:dbl[][])
                          n1474 = local write "Gráfico"(w1851) -> ()
                        }
                      }
                      frame #8 {
                        w1998 = T5."Enabled" ("Disabled")
                        n1475 = property on="Medição" class="Bool (strict)"("DisabledEnum"=w1998) -> ()  [unwired: 2 in, 2 out]
                        n1476 = local write "Medição"(FALSE ("Medição")) -> ()
                        n1477 = property on="Home" class="Bool (strict)"("Visible"=FALSE) -> ()  [unwired: 2 in, 2 out]
                        n1478 = property on="Parar Teste" class="Bool"("DisabledEnum"=w1998) -> ()  [unwired: 2 in, 2 out]
                      }
                    }
                  }
                }
                n1479 = case shown="False" FALSE {
                  tunnel: [w667 w674] -> w628
                  tunnel: [w668 w673] -> w631
                  frame False {
                    n1480 = local read "Pressão01_CLP[0-4095]"() -> (w672:dbl)
                    n1481 = local read "Pressão02-CLP[0-4095]"() -> (w671:dbl)
                    n1482 = local read "Valores"() -> (w669:T4)
                    n1483 = call "Calculo_Pressao.vi"("X2"=w671, "Valores"=w669, "Calibrador"=TRUE, "X"=w672) -> ("Pressao 2"=w667:dbl, "Pressao"=w668:dbl)  [unwired: 2 in]
                  }
                  frame True {
                    n1484 = call "TESTE_PRESSAO_OFICINA.vi"() -> ("Pressão 2"=w674:dbl, "Pressão 1"=w673:dbl)  [unwired: 10 in]
                  }
                }
                n1485 = local read "P_Bar [KPa]"() -> (w626:dbl)
                n1486 = Add(x=w628, y=w626) -> (x+y=w627:dbl)
                n1487 = call "Media_pressao.vi"("Pressao 2"=w627, "Pressao 1"=w631) -> ("Diferenca pressao"=w633:dbl, "Pressao media"=w634:dbl)  [unwired: 8 in]
                n1488 = local write "SHD-PI-02-Ind."(w627) -> ()
                n1489 = local write "SHD-PI-02"(w627) -> ()
                n1490 = local write "SHD-PI-01-Ind."(w631) -> ()
                n1491 = Build Array(w631, w627) -> (w636:dbl[])
                n1492 = local write "SHD-PI-01"(w631) -> ()
                n1493 = local write "P1-P2"(w633) -> ()
                n1494 = local write "PM"(w634) -> ()
                n1495 = Build Array(w636) -> (w635:dbl[][])
                n1496 = Divide(x=w633, y=w634) -> (x/y=w641:dbl)
                n1497 = Absolute Value(x=w641) -> (abs(x)=w640:dbl)
                n1498 = local write "Gráfico"(w635) -> ()
                n1499 = Greater?(x=w640, y=0.05) -> (0:w639:bool)
                n1500 = case shown="True" w639 {
                  tunnel: [FALSE w678] -> w638
                  frame False {
                    n1501 = property on="HELP-SIT" class="Bool"("Visible"=FALSE) -> ()  [unwired: 2 in, 2 out]
                    n1502 = local write "JANELA"(FALSE ("JANELA")) -> ()
                  }
                  frame True {
                    w678 = TRUE
                    n1503 = property on="HELP-SIT" class="Bool"("Visible"=w678) -> ()  [unwired: 2 in, 2 out]
                  }
                }
              }
              frame 2 {
                n1504 = flat-sequence {
                  frame #0 {
                    n1505 = Current VI's Path() -> (path=w2008:path)
                    n1506 = Strip Path(path=w2008) -> (stripped path=w2009:path)  [unwired: 1 out]
                    n1507 = Build Path(base path=w2009, name or relative path="Alinhamento.vi") -> (appended path=w2004:path)
                    n1508 = Open VI Reference(vi path=w2004, error in (no error)=errorcluster {"status"=FALSE, "code"=0, "source"=""}) -> (vi reference=w2006:refnum<vi>, error out=w2005:errorcluster)  [unwired: 4 in]
                    n1509 = invoke class="VI" method="Run VI"(reference=w2006, error in=w2005, "Wait until done"=FALSE ("Wait Until Done"), "Auto Dispose Ref"=TRUE ("Auto Dispose Reference")) -> ()  [unwired: 1 in, 5 out]
                  }
                  frame #1 {
                    n1510 = local write "Alinhamento"(FALSE ("Alinhamento")) -> ()
                  }
                }
                n1511 = local read "stop VI"() -> (w2002:bool)
              }
              frame 4 {
                n1512 = flat-sequence {
                  frame #0 {
                    n1513 = Current VI's Path() -> (path=w2020:path)
                    n1514 = Strip Path(path=w2020) -> (stripped path=w2021:path)  [unwired: 1 out]
                    n1515 = Build Path(base path=w2021, name or relative path="Teste234.vi") -> (appended path=w2016:path)
                    n1516 = Open VI Reference(vi path=w2016, error in (no error)=errorcluster {"status"=FALSE, "code"=0, "source"=""}) -> (vi reference=w2018:refnum<vi>, error out=w2017:errorcluster)  [unwired: 4 in]
                    n1517 = invoke class="VI" method="Run VI"(reference=w2018, error in=w2017, "Wait until done"=FALSE ("Wait Until Done"), "Auto Dispose Ref"=TRUE ("Auto Dispose Reference")) -> ()  [unwired: 1 in, 5 out]
                  }
                  frame #1 {
                    n1518 = local write "Teste 234"(FALSE ("Alinhamento")) -> ()
                  }
                }
                n1519 = local read "stop VI"() -> (w2014:bool)
              }
            }
            n1520 = Get Variant Attribute(Variant=w513, name="Valores") -> (duplicate Variant=w510:variant, error out=w511:errorcluster)  [unwired: 2 in, 2 out]
            n1521 = local read "Valores"() -> (w509:T4)
            n1522 = Variant To Data(error in=w511, type=w509, Variant=w510) -> (data=→"Valores":T4)  [unwired: 1 out]
            n1523 = local read "JANELA"() -> (w494:bool)
            n1524 = Not(x=w494) -> (.not. x?=w493:bool)
            n1525 = And(x=w493, y=w489) -> (x .and. y?=w491:bool)
            n1526 = Or(x=w491, y="HELP-SIT") -> (x .or. y?=w492:bool)
            n1527 = case shown="False" w492 {
              tunnel: w508 -> [w532 w536]
              tunnel: w507 -> [w531 w535]
              tunnel: [w532 w534] -> w506
              tunnel: [w531 w533] -> w504
              frame False {
              }
              frame True {
                n1528 = stacked-sequence {
                  tunnel: w536 -> [w540 _]
                  tunnel: w535 -> [w539 _]
                  tunnel: [w538 _] -> w534
                  tunnel: [w537 _] -> w533
                  frame #0 {
                    n1529 = invoke class="VI" method="FP.Open"(reference=w540, error in=w539, "State"=T6."Standard") -> (reference out=w538:refnum<vi>, error out=w537:errorcluster)  [unwired: 2 in, 3 out]
                  }
                  frame #1 {
                    n1530 = local write "JANELA"(TRUE ("ERRO-AUX")) -> ()
                  }
                }
              }
            }
            n1531 = invoke class="VI" method="Ctrl Val.Set"(reference=w506, error in=w504, "Control Name"="Erro SIT", "Value"=w489) -> (reference out=w505:refnum<vi>, error out=w503:errorcluster)  [unwired: 1 in, 3 out]
            n1532 = invoke class="VI" method="Ctrl Val.Get"(reference=w505, error in=w503, "Control Name"="led SIT") -> (reference out=w502:refnum<vi>, error out=w501:errorcluster, "Get Control Value Variant"=w498:variant)  [unwired: 1 in, 1 out]
            n1533 = To Variant(anything=TRUE) -> (Variant=w497:variant)
            n1534 = Equal?(x=w498, y=w497) -> (x = y?=→"led SHD":bool)
            n1535 = case shown="True" "Parar Teste" {
              frame False {
              }
              frame True {
                n1536 = local write "Teste"(FALSE ("Teste")) -> ()
              }
            }
          }
        }
        frame #3 {
          w2025 = FALSE ("SKT 2")
          w2026 = T5."Disabled and Grayed Out" ("Disabled")
          w2027 = T5."Disabled and Grayed Out" ("Disabled")
          w2028 = FALSE ("stop VI")
          w2029 = TRUE
          n1537 = local write "cano amarelo"(w2029) -> ()
          n1538 = local write "cano azul h"(w2029) -> ()
          n1539 = local write "cano azul v"(w2029) -> ()
          n1540 = local write "cano roxo"(w2029) -> ()
          n1541 = local write "cano roxo h"(w2029) -> ()
          n1542 = local write "cano verde"(w2029) -> ()
          n1543 = local write "T azul"(w2029) -> ()
          n1544 = local write "T roxo"(w2029) -> ()
          n1545 = local write "SIT-CV-ST"(w2025) -> ()
          n1546 = local write "SIT-CV-ST"(w2025) -> ()
          n1547 = local write "stop VI"(w2028) -> ()
          n1548 = local write "caixinha"(w2028) -> ()
          n1549 = local write "Teste"(w2028) -> ()
          n1550 = local write "Alinhamento"(w2028) -> ()
          n1551 = local write "Calibração"(w2028) -> ()
          n1552 = property on="Medição" class="Bool (strict)"("DisabledEnum"=w2027) -> ()  [unwired: 2 in, 2 out]
          n1553 = property on="Gravar teste" class="Bool (strict)"("DisabledEnum"=w2026) -> ()  [unwired: 2 in, 2 out]
          n1554 = property on="Cluster" class="Clust (strict)"("DisabledEnum"=w2027) -> ()  [unwired: 2 in, 2 out]
          n1555 = property on="Cluster 2" class="Clust (strict)"("DisabledEnum"=w2026) -> ()  [unwired: 2 in, 2 out]
        }
      }
    }
    frame #3 {
      n1556 = invoke class="VI" method="Abort VI"(reference=w2032) -> ()  [unwired: 2 in, 3 out]
      n1557 = invoke class="VI" method="Abort VI"(reference=w2030) -> ()  [unwired: 2 in, 3 out]
      n1558 = invoke class="VI" method="Abort VI"(reference=w2031) -> ()  [unwired: 2 in, 3 out]
      n1559 = flat-sequence {
        frame #0 {
          n1560 = local read "reference"() -> (w2034:refnum<vi>)
          n1561 = To Variant(anything=TRUE) -> (Variant=w2036:variant)
          n1562 = invoke class="VI" method="Ctrl Val.Set"(reference=w2034, "Control Name"="STOP", "Value"=w2036) -> ()  [unwired: 2 in, 5 out]
          n1563 = Wait (ms)(milliseconds to wait=u32 500) -> ()  [unwired: 1 out]
        }
      }
    }
  }
  n1564 = property class="VI"(error in=w25, "Front Panel.Open"=TRUE ("Front Panel Window:Open")) -> ()  [unwired: 1 in, 2 out]
